vi "MultiOpto_1.2_Host.vi"() -> ()   [LabVIEW 2018]
uses:
  D:/NI LabVIEW/MultiOpto/MultiOpto_1.2/AT lib/Spels.AutomationTools.Utility.Wcf.dll
  AT lib/Spels.AutomationTools.Utility.Wcf.dll
  D:/NI LabVIEW/MultiOpto/MultiOpto_1.2/AT lib/AmateurStepperMotor.dll
  AT lib/AmateurStepperMotor.dll
  <instrlib>/niDMM/nidmm.llb/niDMM Resolution in Digits.ctl
  <instrlib>/niDMM/nidmm.llb/niDMM Function.ctl
  <instrlib>/niDCPower/nidcpower.llb/niDCPower Measurement Type.ctl
  <instrlib>/niDMM/nidmm.llb/niDMM Configure Measurement Digits.vi
  <instrlib>/niScope/Configure/Trigger/niScope Configure Trigger Window.vi
  <instrlib>/niScope/Acquire/Fetch/niScope Multi Fetch Cluster.vi
  <instrlib>/niScope/Acquire/Fetch/niScope Fetch.vi
panel:
  in  "SIM_SEL":bool
  in  "SEL path":path=path "D:/NI LabVIEW/MultiOpto/MultiOpto_1.2/Logs/SEL" caption="SEL Path"
  in  "SEL Time Cycle":u32=100
  in  "Считать SIM_SEL":bool
  in  "Desicion Panel":enum32{"Decision Panel", "System Panel"}(tab)
  in  "HMI Stop":bool
  out "SEU":bool caption="SEL"
  out "SEL":bool
  out "DC Power 2 Status":bool caption="DC Power 2"
  out "DC Power 1 Status":bool caption="DC Power 1"
  out "NI DMM 3 Status":bool caption="NI DMM 3"
  out "NI DMM 2 Status":bool caption="NI DMM 2"
  out "NI DMM 1 Status":bool caption="NI DMM 1"
  out "NI Scope Status":bool caption="NI Scope"
  out "Stepper Motor Status":bool caption="Stepper Motor"
  out "Ophir 1 Status":bool caption="Ophir 1"
  out "Ophir 2 Status":bool caption="Ophir 2"
  in  "System Stop":bool=TRUE
  out "Ready Status":bool=TRUE
  out "Power OFF":bool=TRUE
  in  "Tab DC Power 2":enum32{"DC Power 2", "System Panel"}(tab)
  in  "P2 CH2_selcur, A":dbl=0.2 caption="current limit" format="%_6p"
  out "P2 CH2_warning":bool caption="VCC_warning"
  out "P2 CH2_counter":u32 caption="VCC_counter"
  in  "P2 CH2 Used":bool caption="CH2"
  in  "P2 CH2_curlim, A":dbl=0.015 caption="current limit" min=0.01 max=1.0 format="%_6p"
  out "P2 CH2_cur, A":dbl=-2.6497095286784e-07 caption="measurement" format="%_6g"
  in  "P2 CH2, V":dbl caption="voltage level" min=-20.0 max=0.0 format="%_6p"
  out "P2 CH2_char":dbl(graph)=-2.6497095286784e-07
  in  "P2 CH2":bool
  in  "P2 CH0 Used":bool caption="CH0"
  in  "DC POWER 2":refnum<k15>="PXI1Slot3_3" caption="PRBS"
  out "P2 CH0_char":dbl(graph)=0.00011627237241327378
  in  "P2 CH0, V":dbl=1.2000000000000002 caption="voltage level" min=0.0 max=6.0 format="%_6p"
  out "P2 CH0_cur, A":dbl=0.00011627237241327378 caption="measurement" format="%_6g"
  in  "P2 CH0_curlim, A":dbl=0.04 caption="current limit" min=0.01 max=1.0 format="%_6p"
  in  "P2 CH0":bool
  out "P2 CH0_warning":bool caption="VCC_warning"
  out "P2 CH0_counter":u32 caption="VCC_counter"
  in  "P2 CH0_selcur, A":dbl=0.2 caption="current limit" format="%_6p"
  in  "P2 CH1_curlim, A":dbl=0.1 caption="current limit" min=0.01 max=1.0 format="%_6p"
  out "P2 CH1_cur, A":dbl=-6.586231837824974e-06 caption="measurement" format="%_6g"
  in  "P2 CH1, V":dbl=20.0 caption="voltage level" min=0.0 max=20.0 format="%_6p"
  out "P2 CH1_char":dbl(graph)=-6.586231837824974e-06
  in  "P2 CH1":bool
  in  "P2 CH1 Used":bool caption="CH1"
  in  "P2 CH1_selcur, A":dbl=0.2 caption="current limit" format="%_6p"
  out "P2 CH1_counter":u32 caption="VCC_counter"
  out "P2 CH1_warning":bool caption="VCC_warning"
  out "DC Power 2 error out":errorcluster
  in  "Tab DC Power 1":enum32{"DC Power 1", "System Panel"}(tab)
  out "P1 CH2_counter":u32 caption="VCC_counter"
  out "P1 CH2_warning":bool caption="VCC_warning"
  in  "P1 CH2_selcur, A":dbl=0.2 caption="current limit" format="%_6p"
  in  "P1 CH2 Used":bool caption="CH2"
  in  "P1 CH2_curlim, A":dbl=0.01 caption="current limit" min=0.01 max=1.0 format="%_6p"
  out "P1 CH2_cur, A":dbl=1.4003158139382402e-06 caption="measurement" format="%_6g"
  in  "P1 CH2, V":dbl=-5.0 caption="voltage level" min=-20.0 max=0.0 format="%_6p"
  out "P1 CH2_char":dbl(graph)=1.4003158139382402e-06
  in  "P1 CH2":bool
  in  "P1 CH1 Used":bool caption="CH1"
  in  "P1 CH0 Used":bool caption="CH0"
  in  "DC POWER 1":refnum<k15>="PXI1Slot2_2" caption="VСС_+5"
  out "P1 CH0_char":dbl(graph)=8.200132019086688e-05
  in  "P1 CH0, V":dbl=3.3000000000000003 caption="voltage level" min=0.0 max=6.0 format="%_6p"
  out "P1 CH0_cur, A":dbl=8.200132019086688e-05 caption="measurement" format="%_6g"
  in  "P1 CH0_curlim, A":dbl=0.08 caption="current limit" min=0.01 max=1.0 format="%_6p"
  out "P1 CH1_char":dbl(graph)=9.464711192498274e-07
  in  "P1 CH1, V":dbl=2.0 caption="voltage level" min=0.0 max=20.0 format="%_6p"
  out "P1 CH1_cur, A":dbl=9.464711192498274e-07 caption="measurement" format="%_6g"
  in  "P1 CH1_curlim, A":dbl=0.1 caption="current limit" min=0.01 max=1.0 format="%_6p"
  in  "P1 CH0":bool
  in  "P1 CH1":bool
  out "P1 CH0_warning":bool caption="VCC_warning"
  out "P1 CH0_counter":u32 caption="VCC_counter"
  out "P1 CH1_warning":bool caption="VCC_warning"
  out "P1 CH1_counter":u32 caption="VCC_counter"
  in  "P1 CH1_selcur, A":dbl=0.2 caption="current limit" format="%_6p"
  in  "P1 CH0_selcur, A":dbl=0.2 caption="current limit" format="%_6p"
  out "DC Power 1 error out":errorcluster
  out "SEL output file refnum":refnum<file>
  in  "Table Tab":enum32{"Glass Table", "Var", "Log"}(tab)
  in  "Add Log Remark":bool
  in  "Glass Table":string[][](table)=[["", "455 nm", "808 nm", "1550 nm"], ["Glass 1 (H-ZLaF90)", "", "", ""], ["Glass 2 (H-K9L)", "", "", ""], ["Glass 3 (H-ZF7LA)", "", "", ""], ["Glass 4 (H-LaK7A)", "", "", ""]]
  in  "Clear Table":bool
  out "Num of Meas":u32
  in  "Log Remark":string
  out "WL 808":dbl format="%#_4g"
  out "WL 455":dbl format="%#_4g"
  out "WL 1550":dbl format="%#_4g"
  out "WL 1550 Ref":dbl=1.0 format="%#_4g"
  out "WL 455 Ref":dbl=1.0 format="%#_4g"
  out "WL 808 Ref":dbl=1.0 format="%#_4g"
  out "WL 455 Absolute/Reference":string="-" caption="WL 455 Abs/Ref"
  out "WL 808 Absolute/Reference":string="-" caption="WL 808 Abs/Ref"
  out "WL 1550 Absolute/Reference":string="-" caption="WL 1550 Abs/Ref"
  in  "Set Last Meas As Ref":bool
  out "Образец №":string="0"
  in  "All Glass Path":path=path "D:/NI LabVIEW/MultiOpto/MultiOpto_1.2/Logs/All Glass"
  in  "NI Scope":refnum<k15>="PXI1Slot9_2" caption="Scope"
  in  "NI DMM 3":refnum<k15>="PXI1Slot6_3" caption="NI DMM 2"
  in  "Stepper Motor Control":enum32{"Stepper Motor", "System Panel", "Var"}(tab)
  out "Текущая позиция":dbl
  in  "Куда едем?":T1(ring)
  in  "Glass Meas":bool caption="Glass Measurement"
  out "Meas Running":bool
  out "Glass Meas Cycle Running":bool caption="Cycle Running"
  in  "Погнали!":bool
  out "Готово":bool
  in  "Glass Meas Cycle":bool caption="Glass Measament Cycle"
  out "Meas Progress Bar":u8(slide) caption="Measurement Progress Bar" scale=0.0..100.0
  in  "StepDivisor":i32(ring)=8 items=["D1"=1, "D2"=2, "D4"=4, "D8"=8, "D16"=16, "D32"=32]
  in  "Speed":dbl=1000.0
  in  "StepMultiplicationFactor":dbl=1.0
  in  "Стоп_тест":bool
  in  "Тест":bool
  in  "Стоп GoTo":bool
  in  "Meas Wait":u32=500
  out "Av Cur Data String":string="0,000016350563\t"
  out "Glass Num Output File":refnum<file>
  out "Glass 1 Output File":refnum<file>
  out "CH Data String":string="1,200000000000\t0,040047418764\t"
  out "All Cur Data String":string="0,000016366024\t0,000016373619\t0,000016386890\t0,000016310874\t0,000016315407\t"
  out "Meas Time String":string="19:17:01:,978\t"
  out "Glass Meas Path":refnum<file>
  out "Glass 2 Output File":refnum<file>
  out "Glass 3 Output File":refnum<file>
  out "Glass 4 Output File":refnum<file>
  out "Glass Full Log Output File":refnum<file>
  out "Save Glass Log Done":bool=TRUE
  in  "Save Glass Log Data":bool
  out "WL-i":i32
  out "Single Meas Output File":refnum<file>
  in  "NI DMM 3 Tab":enum32{"Amp", "Ohm", "System Panel", "Var"}(tab)
  in  "NI DMM 3 Ampermeter path":path=path "D:/NI LabVIEW/MultiOpto/MultiOpto_1.2/Logs/DMM 3" caption="Ampermeter Path"
  out "NI DMM 3 Current Char":dbl(graph)=0.00060711613514286
  in  "NI DMM 3 Current Wait":u32=100 caption="Wait"
  out "NI DMM 3 Current":dbl=0.00060711613514286 caption="Current" format="%_6g"
  in  "NI DMM 3 units":string(combo)="1000000" caption="Units"
  in  "NI DMM 3 Current Range":string(combo)="-1" caption="Range"
  in  "NI DMM 3 Ohmmeter path":path=path "D:/NI LabVIEW/MultiOpto/MultiOpto_1.2/Logs/DMM 3" caption="Ohmmeter Path"
  out "NI DMM 3 Resistance Char":dbl(graph)=6.67426339573744e-05
  in  "NI DMM 3 Resistance Wait":u32=100 caption="Wait"
  out "NI DMM 3 Resistance":dbl caption="Resistance" format="%_6g"
  in  "NI DMM 3 Resistance units":string(combo)="1" caption="Units"
  in  "NI DMM 3 Resistance Range":string(combo)="-1" caption="Range"
  out "NI DMM 3 Current output file":refnum<file>
  out "NI DMM 3 Resistance output file":refnum<file>
  in  "NI DMM 3 error in":errorcluster
  out "NI DMM 3 Option Return":enum32{"Ampermeter button", "Ohmmeter button"}(ring)
  out "NI DMM 3 error out":errorcluster
  out "DMM 3 Real Current":dbl=6.0711613514286e-10 format="%.15f"
  in  "NI DMM 1":refnum<k15>="PXI1Slot4"
  in  "NI DMM 2":refnum<k15>="PXI1Slot5"
  in  "Ophir 2 Tab":T2(tab)
  out "Ophir 2 Initialization":bool caption="Initialization"
  in  "Ophir 2 Clear":bool caption="Clear"
  out "Ophir 2 MAX":dbl caption="MAX" format="%#_5g"
  out "Ophir 2 Optical Power":dbl caption="Power" format="%#_4g"
  in  "Ophir 2 units":string(combo)="1000" caption="Units"
  in  "Ophir 2 Info":u16(ring)=1 caption="Info" items=["Device : JUNO; s/n:903794", "Head : PD300-IRG-v1; s/n:908004"]
  in  "Ophir 2 Wait":u32=100 caption="Wait"
  out "Ophir 2 Char":dbl(graph)=6.67426339573744e-05
  out "Ophir 2 Over Range":bool caption="Over Range"
  out "Ophir 2 dup Visa Session":refnum<visa-resource-name>="USB0::0x0BD3::0x0777::NI-VISA-10003::RAW" caption="dup Visa Session"
  in  "Ophir 2 GPIB Address (10)":string="10" caption="GPIB Address (10)"
  in  "Ophir 2 Select Communication Protocol":u16(ring) caption="Select Communication Protocol" items=["USB", "RS232", "GPIB"]
  in  "Ophir 2 usb channel":i16 caption="usb channel"
  in  "Ophir 2 Baud Rate (3:9600)":i16(ring)=3 caption="Baud Rate (3:9600)" items=["300", "1200", "4800", "9600", "19200", "38400"]
  in  "Ophir 2 Port Number (default 2)":i16=2 caption="Port Number (default 2)" min=0 max=20
  out "Ophir 2 Real Optical Power":dbl format="%.6e"
  out "Ophir 2 error out":errorcluster caption="error out"
  in  "Ophir 2 error in (no error)":errorcluster caption="error in (no error)"
  in  "Ophir 1 Tab":T3(tab)
  out "Ophir 1 Initialization":bool caption="Initialization"
  in  "Ophir 1 units":string(combo)="1000" caption="Units"
  out "Ophir 1 Optical Power":dbl caption="Power" format="%#_4g"
  out "Ophir 1 MAX":dbl caption="MAX" format="%#_5g"
  in  "Ophir 1 Clear":bool caption="Clear"
  in  "Ophir 1 Info":u16(ring)=1 caption="Info" items=["Device : JUNO; s/n:903795", "Head : PD300R-IR   ; s/n:873888"]
  in  "Ophir 1 Wait":u32=100 caption="Wait"
  out "Ophir 1 Char":dbl(graph)=6.67426339573744e-05
  out "Ophir 1 Over Range":bool caption="Over Range"
  in  "Ophir 1 Select Communication Protocol":u16(ring) caption="Select Communication Protocol" items=["USB", "RS232", "GPIB"]
  in  "Ophir 1 usb channel":i16 caption="usb channel"
  in  "Ophir 1 Port Number (default 2)":i16=1 caption="Port Number (default 2)" min=0 max=20
  in  "Ophir 1 Baud Rate (3:9600)":i16(ring)=3 caption="Baud Rate (3:9600)" items=["300", "1200", "4800", "9600", "19200", "38400"]
  in  "Ophir 1 GPIB Address (10)":string="10" caption="GPIB Address (10)"
  out "Ophir 1 dup Visa Session":refnum<visa-resource-name>="USB0::0x0BD3::0x0777::NI-VISA-10003::RAW" caption="dup Visa Session"
  out "Ophir 1 Real Optical Power":dbl format="%.6e"
  out "Ophir 1 error out":errorcluster caption="error out"
  in  "Ophir 1 error in (no error)":errorcluster caption="error in (no error)"
  in  "NI DMM 2 Tab":enum32{"Amp", "Ohm", "System Panel", "Var"}(tab)
  out "NI DMM 2 Current":dbl=0.7074877999002638 caption="Current" format="%_4g"
  out "NI DMM 2 Current Char":dbl(graph)=0.7074877999002638
  in  "NI DMM 2 Ampermeter path":path=path "D:/NI LabVIEW/MultiOpto/MultiOpto_1.2/Logs/DMM 2" caption="Ampermeter Path"
  in  "NI DMM 2 units":string(combo)="1000000" caption="Units"
  in  "NI DMM 2 Current Range":string(combo)="-1" caption="Range"
  in  "NI DMM 2 Current Wait":u32=100 caption="Wait"
  in  "NI DMM 2 Ohmmeter path":path=path "D:/NI LabVIEW/MultiOpto/MultiOpto_1.2/Logs/DMM 2" caption="Ohmmeter Path"
  out "NI DMM 2 Resistance":dbl caption="Resistance" format="%_6g"
  out "NI DMM 2 Resistance Char":dbl(graph)=6.67426339573744e-05
  in  "NI DMM 2 Resistance units":string(combo)="1" caption="Units"
  in  "NI DMM 2 Resistance Range":string(combo)="-1" caption="Range"
  in  "NI DMM 2 Resistance Wait":u32=100 caption="Wait"
  out "NI DMM 2 Current output file":refnum<file>
  out "NI DMM 2 error out":errorcluster
  in  "NI DMM 2 error in":errorcluster
  out "NI DMM 2 Option Return":enum32{"Ampermeter button", "Ohmmeter button"}(ring)
  out "NI DMM 2 Resistance output file":refnum<file>
  out "DMM 2 Real Current":dbl=7.074877999002638e-07 format="%.15f"
  in  "NI DMM 1 Tab":enum32{"Amp", "Ohm", "System Panel", "Var"}(tab)
  out "NI DMM 1 Current Char":dbl(graph)=0.6705812438667635
  out "NI DMM 1 Current":dbl=0.6705812438667635 caption="Current" format="%_6g"
  in  "NI DMM 1 Ampermeter path":path=path "D:/NI LabVIEW/MultiOpto/MultiOpto_1.2/Logs/DMM 1" caption="Ampermeter Path"
  in  "NI DMM 1 units":string(combo)="1000000" caption="Units"
  in  "NI DMM 1 Current Range":string(combo)="-1" caption="Range"
  in  "NI DMM 1 Current Wait":u32=100 caption="Wait"
  in  "NI DMM 1 Ohmmeter path":path=path "D:/NI LabVIEW/MultiOpto/MultiOpto_1.2/Logs/DMM 1" caption="Ohmmeter Path"
  out "NI DMM 1 Resistance":dbl caption="Resistance" format="%_6g"
  out "NI DMM 1 Resistance Char":dbl(graph)=6.67426339573744e-05
  in  "NI DMM 1 Resistance units":string(combo)="1" caption="Units"
  in  "NI DMM 1 Resistance Range":string(combo)="-1" caption="Range"
  in  "NI DMM 1 Resistance Wait":u32=100 caption="Wait"
  out "NI DMM 1 Current output file":refnum<file>
  out "NI DMM 1 error out":errorcluster
  in  "NI DMM 1 error in":errorcluster
  out "NI DMM 1 Option Return":enum32{"Ampermeter button", "Ohmmeter button"}(ring)
  out "NI DMM 1 Resistance output file":refnum<file>
  out "DMM 1 Real Current":dbl=6.705812438667635e-07 format="%.15f"
  in  "NI Scope Tab":enum32{"NI Scope", "System Panel"}(tab)
  in  "vertical range":dbl=2.0 caption="Vertical Range" format="%.2f"
  out "RealTime Waveform":T4(graph) caption="PC_MON Waveform"
  out "SEU Waveform":T4(graph) caption="SHUTDOWN Waveform"
  in  "Low Level":dbl=0.35 format="%.2f"
  in  "High Level":dbl=0.65 format="%.2f"
  in  "AC/DC/Groun":i32(ring)=1 items=["AC", "DC", "Ground"]
  in  "Trigger Source":string(combo)="0"
  in  "SEU path":path=path "D:/NI LabVIEW/MultiOpto 1.1/Logs/SEU" caption="SEU Path"
  in  "Channel for SEU":T5(radio)
  out "SEU Last Level":dbl
  out "SEU_Counter":u32 caption="SEU counter"
  out "SEU_warning":bool caption="Find SEL"
  out "SEU output file refnum":refnum<file>
  out "NI Scope error out":errorcluster
  in  "NI Scope error in":errorcluster
  # "Отожми кнопку для\nединичного промера!"
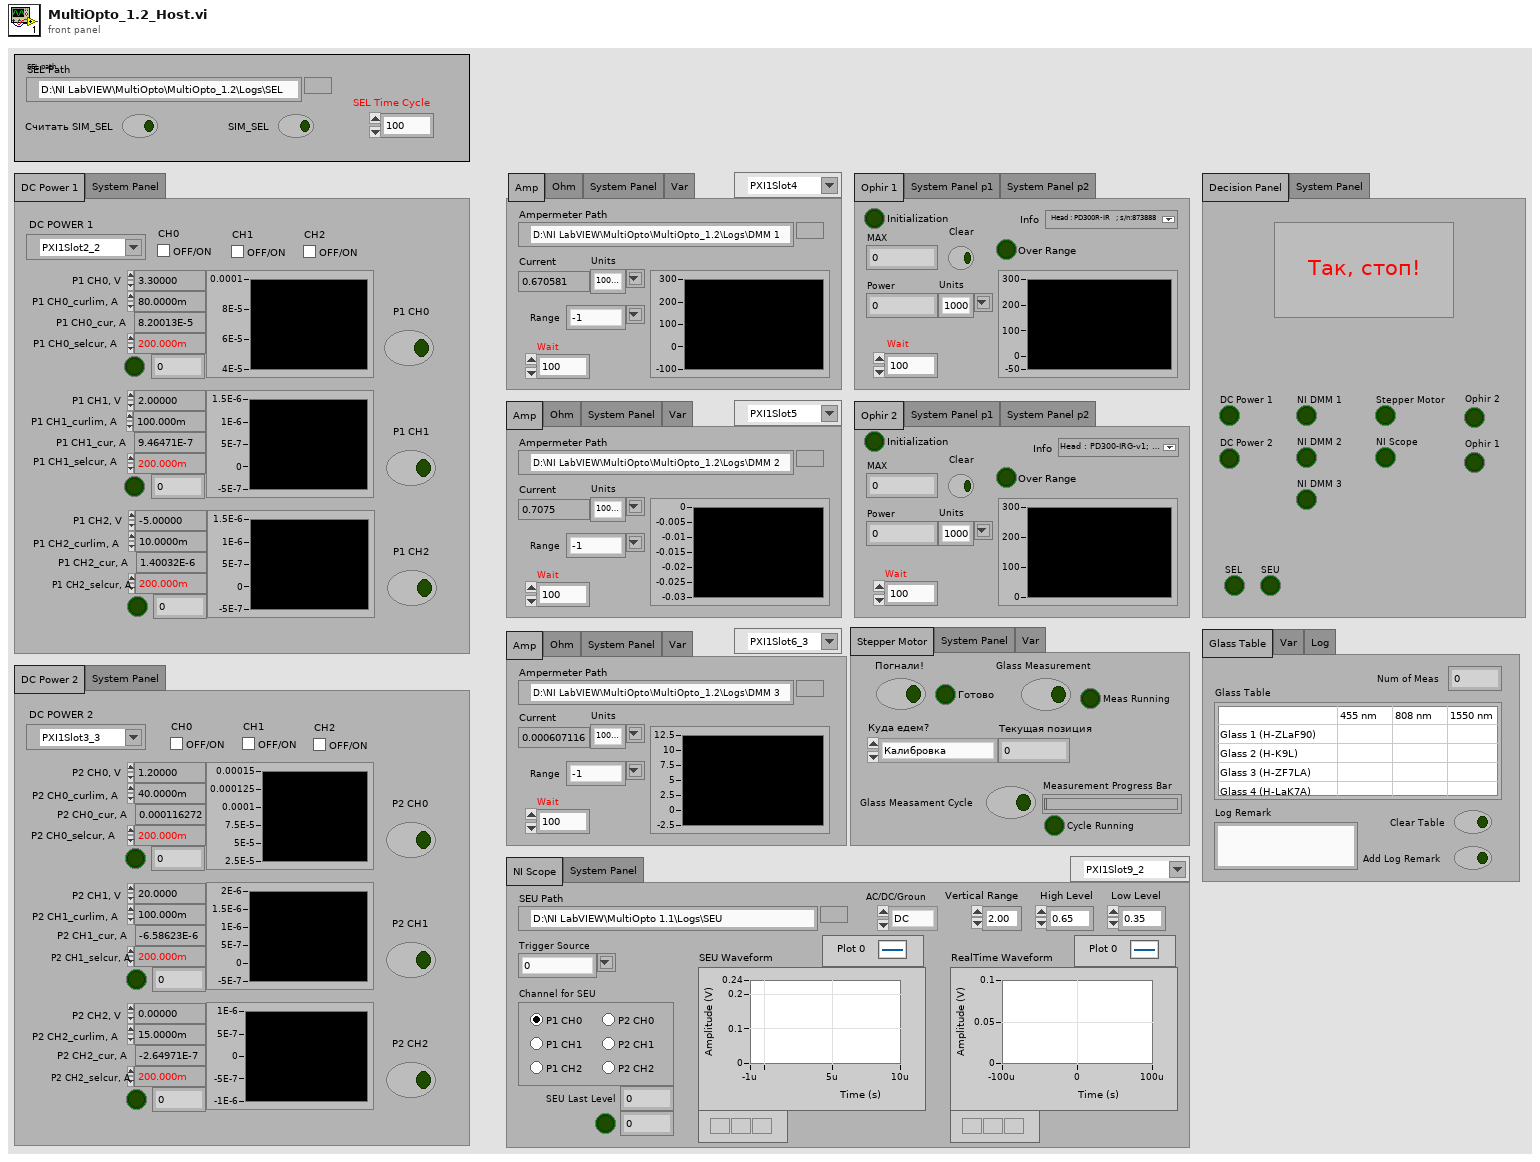
[diagram p1: front panel]
types:
  T1 = enum16{"Калибровка", "Первое стекло", "Второе стекло", "Третье стекло", "Четвертое стекло"}
  T2 = enum32{"Ophir 2", "System Panel p1", "System Panel p2"}
  T3 = enum32{"Ophir 1", "System Panel p1", "System Panel p2"}
  T4 = cluster{"relativeInitialX":dbl, "xIncrement":dbl, "wfm":dbl[]}[]
  T5 = enum32{"Radio Selection P1 CH0", "Radio Selection P1 CH1", "Radio Selection P2 CH0", "Radio Selection P2 CH1", "Radio Selection P2 CH2", "Radio Selection P1 CH2"}
  T6 = enum16{"open", "replace", "create", "open or create", "replace or create", "replace or create with confirmation"}
  T7 = enum8{"Enabled", "Disabled", "Disabled and Grayed Out"}
  T8 = typedef "niDMM Function.ctl" = enum16{"DC Volts", "AC Volts", "DC Current", "AC Current", "2-wire Resistance", "4-wire Resistance", "Diode", "Frequency", "Period", "AC Volts DC Coupled", "Capacitance", "Inductance", "Temperature"}
  T9 = typedef "niDMM Resolution in Digits.ctl" = dbl
  T10 = typedef "niDCPower Measurement Type.ctl" = i32
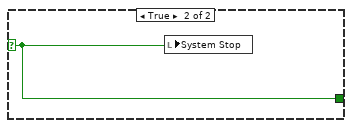
[diagram p5: hidden frame]
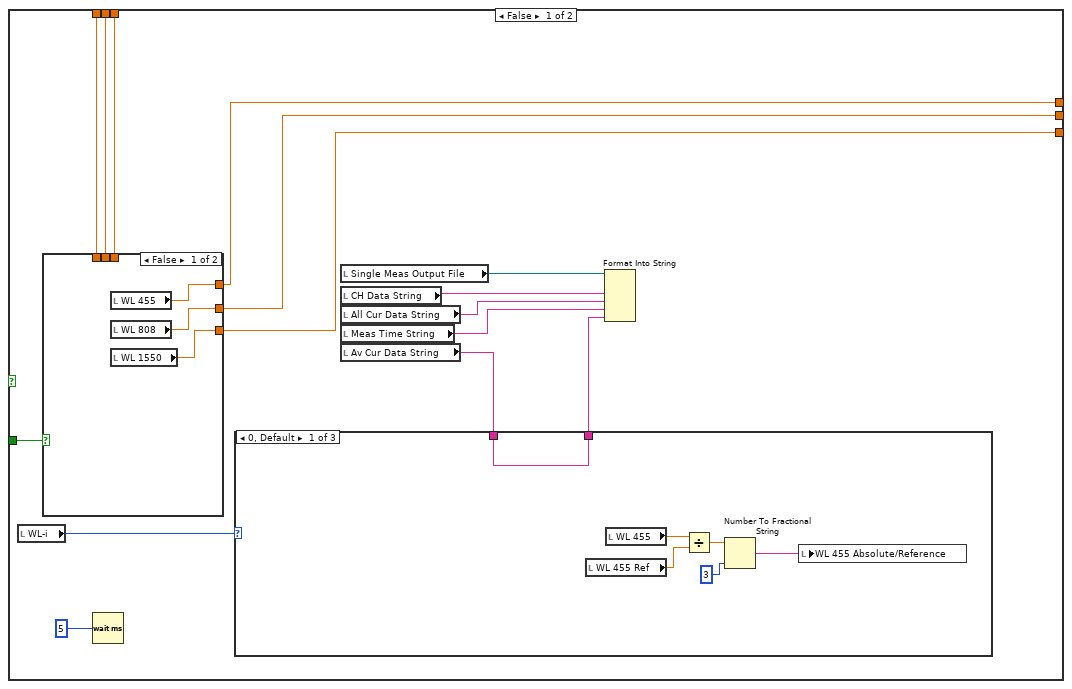
[diagram p9: hidden frame]
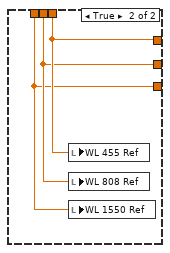
[diagram p10: hidden frame]
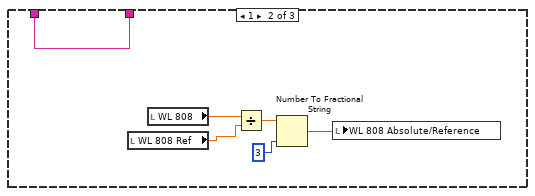
[diagram p11: hidden frame]
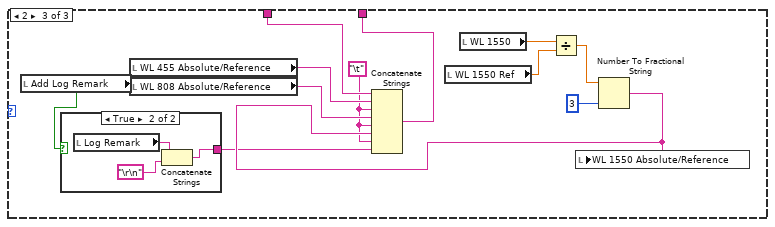
[diagram p12: hidden frame]
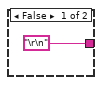
[diagram p13: hidden frame]
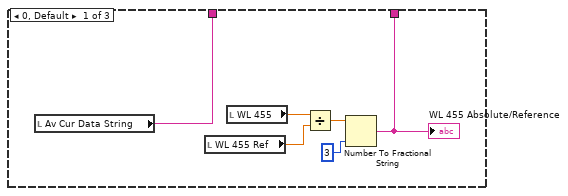
[diagram p14: hidden frame]
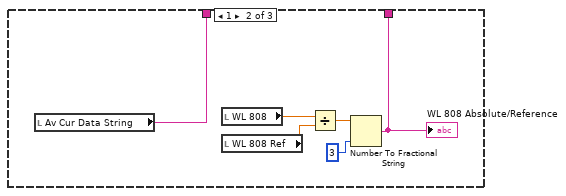
[diagram p15: hidden frame]
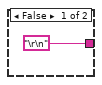
[diagram p16: hidden frame]
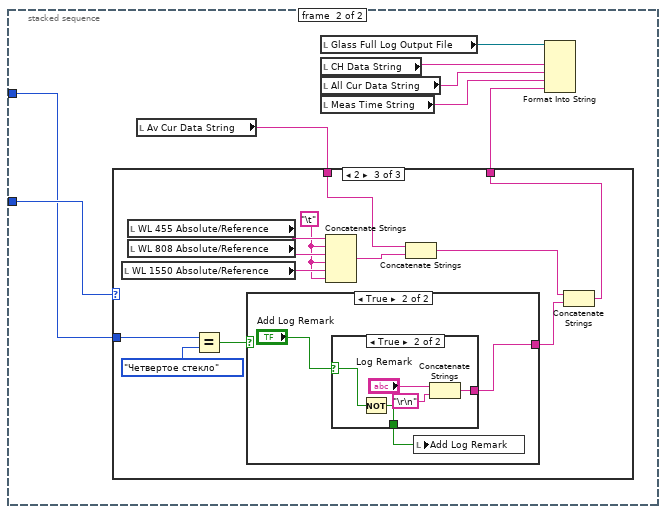
[diagram p17: hidden frame]
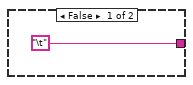
[diagram p20: hidden frame]
diagram:
  # "DMM 3"
  # "DMM 2"
  # "DMM 1"
  n1 = stacked-sequence {
    tunnel: [_ _ _ _ _ w336 _ _ _ _ _ _] -> w36
    tunnel: [_ _ _ _ _ w335 _ _ _ _ _ _] -> w34
    tunnel: [_ _ _ _ _ w334 _ _ _ _ _ _] -> w7
    tunnel: [_ _ _ _ _ _ _ _ _ _ _ w687] -> w8
    tunnel: [_ _ _ _ _ _ _ _ _ _ _ w687] -> w10
    tunnel: [_ _ _ _ _ _ w361 _ _ _ _ _] -> w33
    tunnel: [_ _ _ _ _ _ _ w420 _ _ _ _] -> w32
    tunnel: [_ _ _ _ _ _ _ w423 _ _ _ _] -> w31
    tunnel: [_ _ _ _ _ _ w360 _ _ _ _ _] -> w30
    tunnel: [_ _ _ _ _ _ _ w419 _ _ _ _] -> w29
    tunnel: [_ _ _ _ _ _ _ w418 _ _ _ _] -> w28
    tunnel: [_ _ _ _ _ _ w359 _ _ _ _ _] -> w27
    tunnel: [_ _ _ _ _ _ _ w422 _ _ _ _] -> w26
    tunnel: [_ _ _ _ _ _ _ w421 _ _ _ _] -> w25
    tunnel: [_ _ _ _ _ _ _ _ w616 _ _ _] -> w24
    tunnel: [_ _ _ _ _ _ _ _ _ w639 _ _] -> w23
    tunnel: [_ _ _ _ _ _ _ w417 _ _ _ _] -> w9
    tunnel: [_ _ _ _ _ _ _ w416 _ _ _ _] -> w22
    tunnel: [_ _ _ _ _ _ _ w415 _ _ _ _] -> w21
    tunnel: [_ _ _ _ _ _ _ _ _ _ w665 _] -> w20
    tunnel: [_ _ _ _ _ _ _ _ _ _ w664 _] -> w19
    tunnel: [_ _ _ _ _ _ _ _ _ _ w663 _] -> w18
    tunnel: [_ _ _ _ _ _ _ _ _ _ w662 _] -> w17
    tunnel: [_ _ _ _ _ w333 _ _ _ _ _ _] -> w6
    tunnel: [_ _ _ _ _ w332 _ _ _ _ _ _] -> w3
    tunnel: [_ _ _ _ _ w331 _ _ _ _ _ _] -> w2
    frame #0 {
      w51 = FALSE ("Clear Table")
      w54 = "-" ("WL 455 Absolute/Reference")
      w55 = 0.0 ("WL 455 Ref")
      w56 = 1.0 ("WL 455")
      w58 = "\t" ("Meas Time String")
      w60 = FALSE ("Save Glass Log Done")
      w62 = FALSE ("Погнали!")
      w66 = FALSE
      w65 = FALSE ("NI Scope Status")
      w69 = u32 0 ("SEU_Counter")
      w59 = FALSE ("STOP")
      # "Начальная конфигурация переменных"
      n2 = local write "Текущая позиция"(0.0 ("Текущая позиция")) -> ()
      n3 = local write "Куда едем?"(T1."Калибровка" ("Куда едем?")) -> ()
      n4 = local write "Погнали!"(w62) -> ()
      n5 = local write "Тест"(w62) -> ()
      n6 = local write "Стоп GoTo"(w62) -> ()
      n7 = local write "Стоп_тест"(w62) -> ()
      n8 = local write "Готово"(w62) -> ()
      n9 = local write "Num of Meas"(u32 0 ("Num of Meas")) -> ()
      n10 = local write "WL 455"(w56) -> ()
      n11 = local write "WL 808"(w56) -> ()
      n12 = local write "WL 1550"(w56) -> ()
      n13 = local write "WL 455 Ref"(w55) -> ()
      n14 = local write "WL 808 Ref"(w55) -> ()
      n15 = local write "WL 1550 Ref"(w55) -> ()
      n16 = local write "WL 455 Absolute/Reference"(w54) -> ()
      n17 = local write "WL 808 Absolute/Reference"(w54) -> ()
      n18 = local write "WL 1550 Absolute/Reference"(w54) -> ()
      n19 = local write "Ophir 2 Over Range"(w66) -> ()
      n20 = local write "Ophir 1 Over Range"(w66) -> ()
      n21 = local write "Ophir 1 Initialization"(w66) -> ()
      n22 = local write "Ophir 2 Initialization"(w66) -> ()
      n23 = local write "Ophir 1 Clear"(w66) -> ()
      n24 = local write "Ophir 2 Clear"(w66) -> ()
      n25 = local write "Meas Time String"(w58) -> ()
      n26 = local write "All Cur Data String"(w58) -> ()
      n27 = local write "Av Cur Data String"(w58) -> ()
      n28 = local write "CH Data String"(w58) -> ()
      n29 = local write "WL-i"(0 ("i-WL")) -> ()
      n30 = local write "Save Glass Log Data"(w60) -> ()
      n31 = local write "Save Glass Log Done"(w60) -> ()
      n32 = local write "Glass Meas Cycle"(w60) -> ()
      n33 = local write "Glass Meas"(w60) -> ()
      n34 = local write "Meas Running"(w60) -> ()
      n35 = local write "Glass Meas Cycle Running"(w60) -> ()
      n36 = local write "HMI Stop"(w59) -> ()
      n37 = local write "System Stop"(w59) -> ()
      n38 = local write "P1 CH0"(w59) -> ()
      n39 = local write "P1 CH1"(w59) -> ()
      n40 = local write "P2 CH0"(w59) -> ()
      n41 = local write "P2 CH1"(w59) -> ()
      n42 = local write "Power OFF"(w59) -> ()
      n43 = local write "P1 CH0 Used"(w59) -> ()
      n44 = local write "P1 CH1 Used"(w59) -> ()
      n45 = local write "P1 CH2 Used"(w59) -> ()
      n46 = local write "P2 CH0 Used"(w59) -> ()
      n47 = local write "P2 CH1 Used"(w59) -> ()
      n48 = local write "P2 CH2 Used"(w59) -> ()
      n49 = local write "Считать SIM_SEL"(w59) -> ()
      n50 = local write "SEL"(w59) -> ()
      n51 = local write "SEU"(w59) -> ()
      n52 = local write "SEU_warning"(w59) -> ()
      n53 = local write "P1 CH0_warning"(w59) -> ()
      n54 = local write "P1 CH1_warning"(w59) -> ()
      n55 = local write "P2 CH0_warning"(w59) -> ()
      n56 = local write "P2 CH1_warning"(w59) -> ()
      n57 = local write "SEU_warning"(w59) -> ()
      n58 = local write "Log Remark"("" ("Log Remark")) -> ()
      n59 = local write "Set Last Meas As Ref"(w51) -> ()
      n60 = local write "Clear Table"(w51) -> ()
      n61 = local write "Add Log Remark"(w51) -> ()
      n62 = local write "SEU Last Level"(0.0 ("SEU Level")) -> ()
      n63 = local write "SEU_Counter"(w69) -> ()
      n64 = local write "P1 CH0_counter"(w69) -> ()
      n65 = local write "P1 CH1_counter"(w69) -> ()
      n66 = local write "P2 CH0_counter"(w69) -> ()
      n67 = local write "P2 CH1_counter"(w69) -> ()
      n68 = local write "Образец №"("" ("Образец №")) -> ()
      n69 = local write "Ready Status"(FALSE ("Ready Status")) -> ()
      n70 = local write "NI Scope Status"(w65) -> ()
      n71 = local write "NI DMM 2 Status"(w65) -> ()
      n72 = local write "NI DMM 1 Status"(w65) -> ()
      n73 = local write "NI DMM 3 Status"(w65) -> ()
      n74 = local write "Ophir 1 Status"(w65) -> ()
      n75 = local write "Ophir 2 Status"(w65) -> ()
      n76 = local write "Stepper Motor Status"(w65) -> ()
      "Meas Progress Bar" <- u8 0 ("Measuering Progress Bar")
    }
    frame #1 {
      n77 = stacked-sequence {
        frame #0 {
          w71 = T7."Disabled and Grayed Out" ("Disabled")
          n78 = property on="P1 CH0" class="Bool (strict)"("DisabledEnum"=w71) -> ()  [unwired: 2 in, 2 out]
          n79 = property on="P1 CH0_char" class="WFChart (strict)"("DisabledEnum"=w71) -> ()  [unwired: 2 in, 2 out]
          n80 = property on="P1 CH0, V" class="DigNum (strict)"("DisabledEnum"=w71) -> ()  [unwired: 2 in, 2 out]
          n81 = property on="P1 CH0_curlim, A" class="DigNum (strict)"("DisabledEnum"=w71) -> ()  [unwired: 2 in, 2 out]
          n82 = property on="P1 CH0_cur, A" class="DigNum (strict)"("DisabledEnum"=w71) -> ()  [unwired: 2 in, 2 out]
          n83 = property on="P1 CH0_selcur, A" class="DigNum (strict)"("DisabledEnum"=w71) -> ()  [unwired: 2 in, 2 out]
          n84 = property on="P1 CH0_counter" class="DigNum (strict)"("DisabledEnum"=w71) -> ()  [unwired: 2 in, 2 out]
          n85 = property on="P1 CH0_warning" class="Bool (strict)"("DisabledEnum"=w71) -> ()  [unwired: 2 in, 2 out]
        }
        frame #1 {
          w72 = T7."Disabled and Grayed Out" ("Disabled")
          n86 = property on="P1 CH1" class="Bool (strict)"("DisabledEnum"=w72) -> ()  [unwired: 2 in, 2 out]
          n87 = property on="P1 CH1_char" class="WFChart (strict)"("DisabledEnum"=w72) -> ()  [unwired: 2 in, 2 out]
          n88 = property on="P1 CH1, V" class="DigNum (strict)"("DisabledEnum"=w72) -> ()  [unwired: 2 in, 2 out]
          n89 = property on="P1 CH1_curlim, A" class="DigNum (strict)"("DisabledEnum"=w72) -> ()  [unwired: 2 in, 2 out]
          n90 = property on="P1 CH1_cur, A" class="DigNum (strict)"("DisabledEnum"=w72) -> ()  [unwired: 2 in, 2 out]
          n91 = property on="P1 CH1_selcur, A" class="DigNum (strict)"("DisabledEnum"=w72) -> ()  [unwired: 2 in, 2 out]
          n92 = property on="P1 CH1_counter" class="DigNum (strict)"("DisabledEnum"=w72) -> ()  [unwired: 2 in, 2 out]
          n93 = property on="P1 CH1_warning" class="Bool (strict)"("DisabledEnum"=w72) -> ()  [unwired: 2 in, 2 out]
        }
        frame #2 {
          w73 = T7."Disabled and Grayed Out" ("Disabled")
          n94 = property on="P1 CH2" class="Bool (strict)"("DisabledEnum"=w73) -> ()  [unwired: 2 in, 2 out]
          n95 = property on="P1 CH2_char" class="WFChart (strict)"("DisabledEnum"=w73) -> ()  [unwired: 2 in, 2 out]
          n96 = property on="P1 CH2, V" class="DigNum (strict)"("DisabledEnum"=w73) -> ()  [unwired: 2 in, 2 out]
          n97 = property on="P1 CH2_curlim, A" class="DigNum (strict)"("DisabledEnum"=w73) -> ()  [unwired: 2 in, 2 out]
          n98 = property on="P1 CH2_cur, A" class="DigNum (strict)"("DisabledEnum"=w73) -> ()  [unwired: 2 in, 2 out]
          n99 = property on="P1 CH2_selcur, A" class="DigNum (strict)"("DisabledEnum"=w73) -> ()  [unwired: 2 in, 2 out]
          n100 = property on="P1 CH2_counter" class="DigNum (strict)"("DisabledEnum"=w73) -> ()  [unwired: 2 in, 2 out]
          n101 = property on="P1 CH2_warning" class="Bool (strict)"("DisabledEnum"=w73) -> ()  [unwired: 2 in, 2 out]
        }
        frame #3 {
          w74 = T7."Disabled and Grayed Out" ("Disabled")
          n102 = property on="P2 CH0" class="Bool (strict)"("DisabledEnum"=w74) -> ()  [unwired: 2 in, 2 out]
          n103 = property on="P2 CH0_char" class="WFChart (strict)"("DisabledEnum"=w74) -> ()  [unwired: 2 in, 2 out]
          n104 = property on="P2 CH0, V" class="DigNum (strict)"("DisabledEnum"=w74) -> ()  [unwired: 2 in, 2 out]
          n105 = property on="P2 CH0_curlim, A" class="DigNum (strict)"("DisabledEnum"=w74) -> ()  [unwired: 2 in, 2 out]
          n106 = property on="P2 CH0_cur, A" class="DigNum (strict)"("DisabledEnum"=w74) -> ()  [unwired: 2 in, 2 out]
          n107 = property on="P2 CH0_selcur, A" class="DigNum (strict)"("DisabledEnum"=w74) -> ()  [unwired: 2 in, 2 out]
          n108 = property on="P2 CH0_counter" class="DigNum (strict)"("DisabledEnum"=w74) -> ()  [unwired: 2 in, 2 out]
          n109 = property on="P2 CH0_warning" class="Bool (strict)"("DisabledEnum"=w74) -> ()  [unwired: 2 in, 2 out]
        }
        frame #4 {
          w75 = T7."Disabled and Grayed Out" ("Disabled")
          n110 = property on="P2 CH1" class="Bool (strict)"("DisabledEnum"=w75) -> ()  [unwired: 2 in, 2 out]
          n111 = property on="P2 CH1_char" class="WFChart (strict)"("DisabledEnum"=w75) -> ()  [unwired: 2 in, 2 out]
          n112 = property on="P2 CH1, V" class="DigNum (strict)"("DisabledEnum"=w75) -> ()  [unwired: 2 in, 2 out]
          n113 = property on="P2 CH1_curlim, A" class="DigNum (strict)"("DisabledEnum"=w75) -> ()  [unwired: 2 in, 2 out]
          n114 = property on="P2 CH1_cur, A" class="DigNum (strict)"("DisabledEnum"=w75) -> ()  [unwired: 2 in, 2 out]
          n115 = property on="P2 CH1_selcur, A" class="DigNum (strict)"("DisabledEnum"=w75) -> ()  [unwired: 2 in, 2 out]
          n116 = property on="P2 CH1_counter" class="DigNum (strict)"("DisabledEnum"=w75) -> ()  [unwired: 2 in, 2 out]
          n117 = property on="P2 CH1_warning" class="Bool (strict)"("DisabledEnum"=w75) -> ()  [unwired: 2 in, 2 out]
        }
        frame #5 {
          w76 = T7."Disabled and Grayed Out" ("Disabled")
          n118 = property on="P2 CH2" class="Bool (strict)"("DisabledEnum"=w76) -> ()  [unwired: 2 in, 2 out]
          n119 = property on="P2 CH2_char" class="WFChart (strict)"("DisabledEnum"=w76) -> ()  [unwired: 2 in, 2 out]
          n120 = property on="P2 CH2, V" class="DigNum (strict)"("DisabledEnum"=w76) -> ()  [unwired: 2 in, 2 out]
          n121 = property on="P2 CH2_curlim, A" class="DigNum (strict)"("DisabledEnum"=w76) -> ()  [unwired: 2 in, 2 out]
          n122 = property on="P2 CH2_cur, A" class="DigNum (strict)"("DisabledEnum"=w76) -> ()  [unwired: 2 in, 2 out]
          n123 = property on="P2 CH2_selcur, A" class="DigNum (strict)"("DisabledEnum"=w76) -> ()  [unwired: 2 in, 2 out]
          n124 = property on="P2 CH2_counter" class="DigNum (strict)"("DisabledEnum"=w76) -> ()  [unwired: 2 in, 2 out]
          n125 = property on="P2 CH2_warning" class="Bool (strict)"("DisabledEnum"=w76) -> ()  [unwired: 2 in, 2 out]
        }
        frame #6 {
          w77 = T7."Enabled" ("Disabled")
          n126 = property on="P1 CH0 Used" class="Bool (strict)"("DisabledEnum"=w77) -> ()  [unwired: 2 in, 2 out]
          n127 = property on="P1 CH1 Used" class="Bool (strict)"("DisabledEnum"=w77) -> ()  [unwired: 2 in, 2 out]
          n128 = property on="P1 CH2 Used" class="Bool (strict)"("DisabledEnum"=w77) -> ()  [unwired: 2 in, 2 out]
          n129 = property on="P2 CH0 Used" class="Bool (strict)"("DisabledEnum"=w77) -> ()  [unwired: 2 in, 2 out]
          n130 = property on="P2 CH1 Used" class="Bool (strict)"("DisabledEnum"=w77) -> ()  [unwired: 2 in, 2 out]
          n131 = property on="P2 CH2 Used" class="Bool (strict)"("DisabledEnum"=w77) -> ()  [unwired: 2 in, 2 out]
          n132 = property on="Glass Meas" class="Bool (strict)"("DisabledEnum"=w77) -> ()  [unwired: 2 in, 2 out]
        }
      }
    }
    frame #2 {
      n133 = call "MultiOpto_1.2_Begin.vi"() -> ("Текущий Образец №"=→"Образец №":string, "NI Scope Status"=→"NI Scope Status":bool, "Ophir 1 Status"=→"Ophir 1 Status":bool, "Ophir 2 Status"=→"Ophir 2 Status":bool, "DC Power 1 Status"=→"DC Power 1 Status":bool, "DC Power 2 Status"=→"DC Power 2 Status":bool, "NI DMM 1 Status"=→"NI DMM 1 Status":bool, "NI DMM 2 Status"=→"NI DMM 2 Status":bool, "Stepper Motor Status"=→"Stepper Motor Status":bool, "NI DMM 3 option return"=→"NI DMM 3 Option Return":enum32{"Ampermeter button", "Ohmmeter button"}, "NI DMM 2 option return"=→"NI DMM 2 Option Return":enum32{"Ampermeter button", "Ohmmeter button"}, "NI DMM 1 option return"=→"NI DMM 1 Option Return":enum32{"Ampermeter button", "Ohmmeter button"}, "NI DMM 3 Status"=→"NI DMM 3 Status":bool)  [unwired: 3 in]
    }
    frame #3 {
      n134 = local read "Образец №"() -> (w96:string)
      n135 = Build Path(base path="All Glass Path", name or relative path=w96) -> (appended path=w93:path)
      n136 = call <vilib>:"Check if File or Folder Exists.vi"("path"=w93) -> ("file or folder exists?"=w94:bool, "dup path"=w95:path)  [unwired: 8 in, 1 out]
      n137 = case shown="False" w94 {
        tunnel: w95 -> [w98 w99]
        tunnel: [w97 w99] -> w92
        frame False {
          n138 = Create Folder(path (use dialog)=w98) -> (created path=w97:path)  [unwired: 2 in, 2 out]
        }
        frame True {
        }
      }
      n139 = stacked-sequence {
        tunnel: w92 -> [w152 w182 w229]
        frame #0 {
          w150 = "\t"
          w102 = "\t"
          n140 = local read "Glass Table"() -> (w108:string[][])
          n141 = Index Array(array=w108, index (row)=4 ("disabled index (row)"), index (col)=0 ("disabled index (col)")) -> (element=w106:string)
          n142 = local read "Glass Table"() -> (w113:string[][])
          n143 = Index Array(array=w113, index (row)=3 ("disabled index (row)"), index (col)=0 ("disabled index (col)")) -> (element=w107:string)
          n144 = local read "Glass Table"() -> (w119:string[][])
          n145 = Index Array(array=w119, index (row)=2 ("disabled index (row)"), index (col)=0 ("disabled index (col)")) -> (element=w118:string)
          n146 = Build Path(base path=w152, name or relative path="Full Log") -> (appended path=w169:path)
          n147 = Get Date/Time In Seconds() -> (seconds since 1Jan1904=w165:timestamp)
          n148 = local read "Glass Table"() -> (w117:string[][])
          n149 = call <vilib>:"Check if File or Folder Exists.vi"("path"=w169) -> ("file or folder exists?"=w168:bool, "dup path"=w167:path)  [unwired: 8 in, 1 out]
          n150 = Index Array(array=w117, index (row)=1 ("disabled index (row)"), index (col)=0 ("disabled index (col)")) -> (element=w114:string)
          n151 = Format Date/Time String(time format string (%c)="Full Log %d %m %y %H.%M.%S", seconds (now)=w165) -> (date/time string=w164:string)  [unwired: 1 in]
          n152 = case shown="False" w168 {
            tunnel: w167 -> [w171 w172]
            tunnel: [w170 w172] -> w166
            frame False {
              n153 = Create Folder(path (use dialog)=w171) -> (created path=w170:path)  [unwired: 2 in, 2 out]
            }
            frame True {
            }
          }
          n154 = Concatenate Strings(w164, ".xls" ("string")) -> (w163:string)
          n155 = Build Path(base path=w166, name or relative path=w163) -> (appended path=w162:path)
          n156 = Concatenate Strings("P1 CH0, V" ("string"), w102, "P1 CH0 Current, A" ("string"), w102, "DMM1_1" ("string"), w102, "DMM1_2" ("string"), w102, "DMM1_3" ("string"), w102, "DMM1_4" ("string"), w102, "DMM1_5" ("string"), w102, "Time" ("string"), w102, "455 nm Current Averaged, A" ("string"), w102, "P2 CH0, V" ("string"), w102, "P2 CH0 Current, A" ("string"), w102, "DMM2_1" ("string"), w102, "DMM2_2" ("string"), w102, "DMM2_3" ("string"), w102, "DMM2_4" ("string"), w102, "DMM2_5" ("string"), w102, "Time" ("string"), w102, "808 nm Current Averaged, A" ("string"), w102, "P2 CH1, V" ("string"), w102, "P2 CH2 Current, A" ("string"), w102, "DMM3_1" ("string"), w102, "DMM3_2" ("string"), w102, "DMM3_3" ("string"), w102, "DMM3_4" ("string"), w102, "DMM3_5" ("string"), w102, "Time" ("string"), w102, "1550 nm Current Averaged, A" ("string"), w102, "455 nm Absolute/Reference" ("string"), w102, "808 nm Absolute/Reference" ("string"), w102, "1550 nm Absolute/Reference" ("string"), w102) -> (w149:string)
          n157 = Open/Create/Replace File(file path (use dialog)=w162, operation (0:open)=T6."open or create", access (0:read/write)=enum16{"read/write", "read-only", "write-only"}."read/write") -> (refnum out=w161:refnum<file>)  [unwired: 3 in, 2 out]
          n158 = Set File Position(refnum=w161, from (0:start)=enum16{"start", "end", "current"}."end") -> (refnum out=w159:refnum<file>)  [unwired: 2 in, 1 out]
          n159 = Concatenate Strings(w149, w114, w150, w149, w118, w150, w149, w107, w150, w149, w106, w150, w149, "Log Remarks" ("string"), "\r\n") -> (w158:string)
          n160 = Format Into String(initial string=w159, w158) -> (resulting string=→"Glass Full Log Output File":refnum<file>)  [unwired: 2 in, 1 out]
        }
        frame #1 {
          w175 = "\t"
          n161 = Build Path(base path=w182, name or relative path="Single Measurements") -> (appended path=w224:path)
          n162 = Get Date/Time In Seconds() -> (seconds since 1Jan1904=w220:timestamp)
          n163 = call <vilib>:"Check if File or Folder Exists.vi"("path"=w224) -> ("file or folder exists?"=w223:bool, "dup path"=w222:path)  [unwired: 8 in, 1 out]
          n164 = Format Date/Time String(time format string (%c)="Single Measurements %d %m %y %H.%M.%S", seconds (now)=w220) -> (date/time string=w219:string)  [unwired: 1 in]
          n165 = case shown="False" w223 {
            tunnel: w222 -> [w226 w227]
            tunnel: [w225 w227] -> w221
            frame False {
              n166 = Create Folder(path (use dialog)=w226) -> (created path=w225:path)  [unwired: 2 in, 2 out]
            }
            frame True {
            }
          }
          n167 = Concatenate Strings(w219, ".xls" ("string")) -> (w218:string)
          n168 = Build Path(base path=w221, name or relative path=w218) -> (appended path=w217:path)
          n169 = Concatenate Strings("P1 CH0, V" ("string"), w175, "P1 CH0 Current, A" ("string"), w175, "DMM1_1" ("string"), w175, "DMM1_2" ("string"), w175, "DMM1_3" ("string"), w175, "DMM1_4" ("string"), w175, "DMM1_5" ("string"), w175, "Time" ("string"), w175, "455 nm Current Averaged, A" ("string"), w175, "P1 CH1, V" ("string"), w175, "P1 CH1 Current, A" ("string"), w175, "DMM2_1" ("string"), w175, "DMM2_2" ("string"), w175, "DMM2_3" ("string"), w175, "DMM2_4" ("string"), w175, "DMM2_5" ("string"), w175, "Time" ("string"), w175, "808 nm Current Averaged, A" ("string"), w175, "P2 CH0, V" ("string"), w175, "P2 CH0 Current, A" ("string"), w175, "DMM3_1" ("string"), w175, "DMM3_2" ("string"), w175, "DMM3_3" ("string"), w175, "DMM3_4" ("string"), w175, "DMM3_5" ("string"), w175, "Time" ("string"), w175, "1550 nm Current Averaged, A" ("string"), w175, "455 nm Absolute/Reference" ("string"), w175, "808 nm Absolute/Reference" ("string"), w175, "1550 nm Absolute/Reference" ("string"), w175, "Log Remarks" ("string"), "\r\n") -> (w180:string)
          n170 = Open/Create/Replace File(file path (use dialog)=w217, operation (0:open)=T6."open or create", access (0:read/write)=enum16{"read/write", "read-only", "write-only"}."read/write") -> (refnum out=w216:refnum<file>)  [unwired: 3 in, 2 out]
          n171 = Set File Position(refnum=w216, from (0:start)=enum16{"start", "end", "current"}."end") -> (refnum out=w215:refnum<file>)  [unwired: 2 in, 1 out]
          n172 = Format Into String(initial string=w215, w180) -> (resulting string=→"Single Meas Output File":refnum<file>)  [unwired: 2 in, 1 out]
        }
        frame #2 {
          n173 = for {
            N: 4 -> [_]
            tunnel: w229 -> [w248]
            i -> [w240]
            w232 = "\t"
            w237 = "\t"
            n174 = local read "Glass Table"() -> (w243:string[][])
            n175 = Increment(x=w240) -> (x+1=w239:i32)
            n176 = Index Array(array=w243, index (row)=w239, index (col)=0 ("disabled index (col)")) -> (element=w242:string)
            n177 = Concatenate Strings(w242, " %d %m %y %H.%M.%S" ("time format string (%c)")) -> (w244:string)
            n178 = Build Path(base path=w248, name or relative path=w242) -> (appended path=w275:path)
            n179 = Get Date/Time In Seconds() -> (seconds since 1Jan1904=w271:timestamp)
            n180 = call <vilib>:"Check if File or Folder Exists.vi"("path"=w275) -> ("file or folder exists?"=w274:bool, "dup path"=w273:path)  [unwired: 8 in, 1 out]
            n181 = Format Date/Time String(time format string (%c)=w244, seconds (now)=w271) -> (date/time string=w270:string)  [unwired: 1 in]
            n182 = case shown="False" w274 {
              tunnel: w273 -> [w281 w282]
              tunnel: [w280 w282] -> w272
              frame False {
                n183 = Create Folder(path (use dialog)=w281) -> (created path=w280:path)  [unwired: 2 in, 2 out]
              }
              frame True {
              }
            }
            n184 = Concatenate Strings("P1 CH0, V" ("string"), w237, "P1 CH0 Current, A" ("string"), w237, "Time" ("string"), w237, "455 nm Current Averaged, A" ("string"), w237, "P1 CH1, V" ("string"), w237, "P1 CH1 Current, A" ("string"), w237, "Time" ("string"), w237, "808 nm Current Averaged, A" ("string"), w237, "P2 CH0, V" ("string"), w237, "P2 CH0 Current, A" ("string"), w237, "Time" ("string"), w237, "1550 nm Current Averaged, A" ("string"), w237) -> (w238:string)
            n185 = Concatenate Strings(w270, ".xls" ("string")) -> (w269:string)
            n186 = Build Path(base path=w272, name or relative path=w269) -> (appended path=w268:path)
            n187 = Open/Create/Replace File(file path (use dialog)=w268, operation (0:open)=T6."open or create", access (0:read/write)=enum16{"read/write", "read-only", "write-only"}."read/write") -> (refnum out=w267:refnum<file>)  [unwired: 3 in, 2 out]
            n188 = Concatenate Strings(w238, "455 nm Absolute/Reference" ("string"), w232, "808 nm Absolute/Reference" ("string"), w232, "1550 nm Absolute/Reference" ("string"), w232) -> (w233:string)
            n189 = Set File Position(refnum=w267, from (0:start)=enum16{"start", "end", "current"}."end") -> (refnum out=w262:refnum<file>)  [unwired: 2 in, 1 out]
            n190 = Concatenate Strings(w233, w242, "\t", w233, "Log Remarks" ("string"), "\r\n") -> (w249:string)
            n191 = Format Into String(initial string=w262, w249) -> (resulting string=w247:refnum<file>)  [unwired: 2 in, 1 out]
            n192 = case shown="3" w240 {
              tunnel: w247 -> [w276 w277 w278 w279]
              frame 0, Default {
                "Glass 1 Output File" <- w276
              }
              frame 1 {
                "Glass 2 Output File" <- w277
              }
              frame 2 {
                "Glass 3 Output File" <- w278
              }
              frame 3 {
                "Glass 4 Output File" <- w279
              }
            }
          }
        }
      }
    }
    frame #4 {
      w285 = "\t"
      # "Инициализация файла SEL"
      n193 = local read "Образец №"() -> (w312:string)
      n194 = Build Path(base path="SEL path", name or relative path=w312) -> (appended path=w327:path)
      n195 = Get Date/Time In Seconds() -> (seconds since 1Jan1904=w323:timestamp)
      n196 = call <vilib>:"Check if File or Folder Exists.vi"("path"=w327) -> ("file or folder exists?"=w326:bool, "dup path"=w325:path)  [unwired: 8 in, 1 out]
      n197 = Format Date/Time String(time format string (%c)="SEL %d %m %y %H.%M.%S", seconds (now)=w323) -> (date/time string=w322:string)  [unwired: 1 in]
      n198 = case shown="False" w326 {
        tunnel: w325 -> [w329 w330]
        tunnel: [w328 w330] -> w324
        frame False {
          n199 = Create Folder(path (use dialog)=w329) -> (created path=w328:path)  [unwired: 2 in, 2 out]
        }
        frame True {
        }
      }
      n200 = Concatenate Strings(w322, ".xls" ("string")) -> (w319:string)
      n201 = Build Path(base path=w324, name or relative path=w319) -> (appended path=w316:path)
      n202 = Open/Create/Replace File(file path (use dialog)=w316, operation (0:open)=T6."open or create", access (0:read/write)=enum16{"read/write", "read-only", "write-only"}."read/write") -> (refnum out=w315:refnum<file>)  [unwired: 3 in, 2 out]
      n203 = Set File Position(refnum=w315, from (0:start)=enum16{"start", "end", "current"}."end") -> (refnum out=w296:refnum<file>)  [unwired: 2 in, 1 out]
      n204 = Format Into String(initial string=w296, "Time" ("string"), w285, "P1 CH0, V" ("string"), w285, "P1 CH0_cur, A" ("string"), w285, "P1 CH0_counter" ("string"), w285, "!!!1_0" ("input 7"), w285, "P1 CH1, V" ("string"), w285, "P1 CH1_cur, A" ("string"), w285, "P1 CH1_counter" ("string"), w285, "!!!1_1" ("input 7"), w285, "P1 CH2, V" ("string"), w285, "P1 CH2_cur, A" ("string"), w285, "P1 CH2_counter" ("string"), w285, "!!!1_2" ("input 7"), w285, "P2 CH0, V" ("string"), w285, "P2 CH0_cur, A" ("string"), w285, "P2 CH0_counter" ("string"), w285, "!!!2_0" ("input 7"), w285, "P2 CH1, V" ("string"), w285, "P2 CH1_cur, A" ("string"), w285, "P2 CH1_counter" ("string"), w285, "!!!2_1" ("input 7"), w285, "P2 CH2, V" ("string"), w285, "P2 CH2_cur, A" ("string"), w285, "P2 CH2_counter" ("string"), w285, "!!!2_2" ("input 7"), "\r\n") -> (resulting string=→"SEL output file refnum":refnum<file>)  [unwired: 2 in, 1 out]
    }
    frame #5 {
      # "Инициализация источника"
      n205 = local read "DC Power 1 Status"() -> (w332:bool)
      n206 = local read "DC Power 2 Status"() -> (w331:bool)
      n207 = case shown="True" w332 {
        tunnel: [refnum<k15> refnum ("instrument handle out") w342] -> w336
        tunnel: [errorcluster {"status"=FALSE, "code"=0, "source"=""} ("error out") w341] -> w335
        frame False {
          n208 = property on="Tab DC Power 1" class="TabCtl (strict)"("DisabledEnum"=T7."Disabled and Grayed Out" ("Disabled")) -> ()  [unwired: 2 in, 2 out]
        }
        frame True {
          n209 = property on="Tab DC Power 1" class="TabCtl (strict)"("DisabledEnum"=T7."Enabled" ("Disabled")) -> ()  [unwired: 2 in, 2 out]
          n210 = call <instrlib>:"niDCPower Initialize.vi"("resource name"="DC POWER 1") -> ("error out"=w346:errorcluster, "instrument handle out"=w347:refnum<k15>)  [unwired: 3 in, 6 out]
          n211 = call <instrlib>:"niDCPower Configure Voltage Level.vi"("error in (no error)"=w346, "voltage level"=0.0, "channel name"="0,1", "instrument handle"=w347) -> ("error out"=w341:errorcluster, "instrument handle out"=w342:refnum<k15>)  [unwired: 6 in]
        }
      }
      n212 = case shown="True" w331 {
        tunnel: [refnum<k15> refnum ("instrument handle out") w353] -> w333
        tunnel: [errorcluster {"status"=FALSE, "code"=0, "source"=""} ("error out") w352] -> w334
        frame False {
          n213 = property on="Tab DC Power 2" class="TabCtl (strict)"("DisabledEnum"=T7."Disabled and Grayed Out" ("Disabled")) -> ()  [unwired: 2 in, 2 out]
        }
        frame True {
          n214 = property on="Tab DC Power 2" class="TabCtl (strict)"("DisabledEnum"=T7."Enabled" ("Disabled")) -> ()  [unwired: 2 in, 2 out]
          n215 = call <instrlib>:"niDCPower Initialize.vi"("resource name"="DC POWER 2") -> ("error out"=w357:errorcluster, "instrument handle out"=w358:refnum<k15>)  [unwired: 3 in, 6 out]
          n216 = call <instrlib>:"niDCPower Configure Voltage Level.vi"("error in (no error)"=w357, "voltage level"=0.0, "channel name"="0,1", "instrument handle"=w358) -> ("error out"=w352:errorcluster, "instrument handle out"=w353:refnum<k15>)  [unwired: 6 in]
        }
      }
    }
    frame #6 {
      n217 = local read "NI Scope Status"() -> (w359:bool)
      n218 = case shown="True" w359 {
        tunnel: [refnum<k15> refnum ("instrument handle out") w367] -> w361
        tunnel: [errorcluster {"status"=FALSE, "code"=0, "source"=""} ("error out") w366] -> w360
        frame False {
          n219 = Wait (ms)(milliseconds to wait=u32 1) -> ()  [unwired: 1 out]
          n220 = property on="NI Scope Tab" class="TabCtl (strict)"("DisabledEnum"=T7."Disabled and Grayed Out" ("Disabled")) -> ()  [unwired: 2 in, 2 out]
        }
        frame True {
          n221 = stacked-sequence {
            tunnel: [_ w399] -> w367
            tunnel: [_ w398] -> w366
            frame #0 {
              w378 = "\t"
              # "Инициализация файла SEU"
              n222 = local read "Образец №"() -> (w383:string)
              n223 = Build Path(base path="SEU path", name or relative path=w383) -> (appended path=w393:path)
              n224 = Get Date/Time In Seconds() -> (seconds since 1Jan1904=w389:timestamp)
              n225 = call <vilib>:"Check if File or Folder Exists.vi"("path"=w393) -> ("file or folder exists?"=w392:bool, "dup path"=w391:path)  [unwired: 8 in, 1 out]
              n226 = Format Date/Time String(time format string (%c)="SEU %d %m %y %H.%M.%S", seconds (now)=w389) -> (date/time string=w388:string)  [unwired: 1 in]
              n227 = case shown="True" w392 {
                tunnel: w391 -> [w395 w396]
                tunnel: [w394 w396] -> w390
                frame False {
                  n228 = Create Folder(path (use dialog)=w395) -> (created path=w394:path)  [unwired: 2 in, 2 out]
                }
                frame True {
                }
              }
              n229 = Concatenate Strings(w388, ".xls" ("string")) -> (w387:string)
              n230 = Build Path(base path=w390, name or relative path=w387) -> (appended path=w386:path)
              n231 = Open/Create/Replace File(file path (use dialog)=w386, operation (0:open)=T6."open or create", access (0:read/write)=enum16{"read/write", "read-only", "write-only"}."read/write") -> (refnum out=w385:refnum<file>)  [unwired: 3 in, 2 out]
              n232 = property on="NI Scope Tab" class="TabCtl (strict)"("DisabledEnum"=T7."Enabled" ("Disabled")) -> ()  [unwired: 2 in, 2 out]
              n233 = Set File Position(refnum=w385, from (0:start)=enum16{"start", "end", "current"}."end") -> (refnum out=w382:refnum<file>)  [unwired: 2 in, 1 out]
              n234 = Format Into String(initial string=w382, "Time" ("string"), w378, "Voltage, V" ("string"), w378, "Current, A" ("string"), w378, "SEU counter" ("string"), w378, "!!!" ("input 7"), "\r\n") -> (resulting string=→"SEU output file refnum":refnum<file>)  [unwired: 2 in, 1 out]
            }
            frame #1 {
              w404 = 2 items=["None"=1, "Auto Trigger"=2] ("Triggering:Trigger Modifier")
              w402 = u32 0 items=["1 mega ohm"=0, "50 ohms"=2] ("Input Impedance")
              w400 = FALSE  # Reset Device
              n235 = call <instrlib>:"niScope Initialize.vi"("resource name"="NI Scope", "reset device"=w400, "error in"="NI Scope error in") -> ("instrument handle"=w411:refnum<k15>, "error out"=w410:errorcluster)  [unwired: 11 in]
              n236 = call <instrlib>:"niScope Configure Chan Characteristics.vi"("instrument handle"=w411, "channels"="0" ("Channel Name"), "input impedance"=w402, "maximum input frequency"=20000000.0 ("Maximum Input Frequency"), "error in"=w410) -> ("instrument handle out"=w413:refnum<k15>, "error out"=w409:errorcluster)  [unwired: 9 in]
              n237 = call <instrlib>:"niScope Configure Horizontal Timing.vi"("instrument handle"=w413, "enforce realtime"=TRUE ("Enforce Realtime"), "min sample rate"=250000000.0 ("Min Sample Rate"), "reference position"=50.0 ("Reference\nPosition"), "error in"=w409, "min record length"=1000000 ("Min Record Length")) -> ("instrument handle out"=w412:refnum<k15>, "error out"=w398:errorcluster)  [unwired: 8 in]
              n238 = property on="Property Node" class="niScope"(reference=w412, "Trigger Modifier"=w404) -> (reference out=w399:refnum<k15>)  [unwired: 1 in, 1 out]
            }
          }
        }
      }
    }
    frame #7 {
      # "Инициализация DMM"
      n239 = local read "NI DMM 1 Status"() -> (w422:bool)
      n240 = local read "NI DMM 2 Status"() -> (w421:bool)
      n241 = local read "NI DMM 3 Status"() -> (w417:bool)
      n242 = case shown="True" w417 {
        tunnel: [refnum<k15> refnum ("instrument handle out") w428] -> w415
        tunnel: [errorcluster {"status"=FALSE, "code"=0, "source"=""} ("error out") w429] -> w416
        frame False {
          n243 = property on="NI DMM 3 Tab" class="TabCtl (strict)"("DisabledEnum"=T7."Disabled and Grayed Out" ("Disabled")) -> ()  [unwired: 2 in, 2 out]
        }
        frame True {
          n244 = local read "NI DMM 3 Option Return"() -> (w430:enum32{"Ampermeter button", "Ohmmeter button"})
          n245 = property on="NI DMM 3 Tab" class="TabCtl (strict)"("DisabledEnum"=T7."Enabled" ("Disabled")) -> ()  [unwired: 2 in, 2 out]
          n246 = stacked-sequence {
            tunnel: w430 -> [w431 _]
            tunnel: [_ w485] -> w429
            tunnel: [_ w484] -> w428
            frame #0 {
              n247 = case shown="\"Ampermeter button\", Default" w431 {
                frame "Ampermeter button", Default {
                  # "Инициализация файла SEU"
                  n248 = local read "Образец №"() -> (w447:string)
                  n249 = Build Path(base path="NI DMM 3 Ampermeter path", name or relative path=w447) -> (appended path=w454:path)
                  n250 = Get Date/Time In Seconds() -> (seconds since 1Jan1904=w450:timestamp)
                  n251 = call <vilib>:"Check if File or Folder Exists.vi"("path"=w454) -> ("file or folder exists?"=w453:bool, "dup path"=w452:path)  [unwired: 8 in, 1 out]
                  n252 = Format Date/Time String(time format string (%c)="NI DMM 3 %d %m %y %H.%M.%S", seconds (now)=w450) -> (date/time string=w449:string)  [unwired: 1 in]
                  n253 = case shown="True" w453 {
                    tunnel: w452 -> [w456 w457]
                    tunnel: [w455 w457] -> w451
                    frame False {
                      n254 = Create Folder(path (use dialog)=w456) -> (created path=w455:path)  [unwired: 2 in, 2 out]
                    }
                    frame True {
                    }
                  }
                  n255 = Concatenate Strings(w449, ".xls" ("string")) -> (w448:string)
                  n256 = Build Path(base path=w451, name or relative path=w448) -> (appended path=w433:path)
                  n257 = Open/Create/Replace File(file path (use dialog)=w433, operation (0:open)=T6."open or create", access (0:read/write)=enum16{"read/write", "read-only", "write-only"}."read/write") -> (refnum out=w444:refnum<file>)  [unwired: 3 in, 2 out]
                  n258 = Set File Position(refnum=w444, from (0:start)=enum16{"start", "end", "current"}."end") -> (refnum out=w436:refnum<file>)  [unwired: 2 in, 1 out]
                  n259 = Format Into String(initial string=w436, "Time" ("string"), "\t", "Current, A" ("string"), "\r\n") -> (resulting string=→"NI DMM 3 Current output file":refnum<file>)  [unwired: 2 in, 1 out]
                  n260 = local write "NI DMM 3 Tab"(enum32{"Amp", "Ohm", "System Panel"}."Amp" ("NI DMM 2 Tab")) -> ()
                }
                frame "Ohmmeter button" {
                  n261 = local read "Образец №"() -> (w473:string)
                  n262 = Build Path(base path="NI DMM 3 Ohmmeter path", name or relative path=w473) -> (appended path=w480:path)
                  n263 = Get Date/Time In Seconds() -> (seconds since 1Jan1904=w476:timestamp)
                  n264 = call <vilib>:"Check if File or Folder Exists.vi"("path"=w480) -> ("file or folder exists?"=w479:bool, "dup path"=w478:path)  [unwired: 8 in, 1 out]
                  n265 = Format Date/Time String(time format string (%c)="NI DMM 3 %d %m %y %H.%M.%S", seconds (now)=w476) -> (date/time string=w475:string)  [unwired: 1 in]
                  n266 = case shown="True" w479 {
                    tunnel: w478 -> [w482 w483]
                    tunnel: [w481 w483] -> w477
                    frame False {
                      n267 = Create Folder(path (use dialog)=w482) -> (created path=w481:path)  [unwired: 2 in, 2 out]
                    }
                    frame True {
                    }
                  }
                  n268 = Concatenate Strings(w475, ".xls" ("string")) -> (w474:string)
                  n269 = Build Path(base path=w477, name or relative path=w474) -> (appended path=w459:path)
                  n270 = Open/Create/Replace File(file path (use dialog)=w459, operation (0:open)=T6."open or create", access (0:read/write)=enum16{"read/write", "read-only", "write-only"}."read/write") -> (refnum out=w470:refnum<file>)  [unwired: 3 in, 2 out]
                  n271 = Set File Position(refnum=w470, from (0:start)=enum16{"start", "end", "current"}."end") -> (refnum out=w462:refnum<file>)  [unwired: 2 in, 1 out]
                  n272 = Format Into String(initial string=w462, "Time" ("string"), "\t", "Current, A" ("string"), "\r\n") -> (resulting string=→"NI DMM 3 Resistance output file":refnum<file>)  [unwired: 2 in, 1 out]
                  n273 = local write "NI DMM 3 Tab"(enum32{"Amp", "Ohm", "System Panel"}."Ohm" ("NI DMM 2 Tab")) -> ()
                }
              }
            }
            frame #1 {
              n274 = call <instrlib>:"niDMM Initialize.vi"("error in (no error)"="NI DMM 3 error in", "Instrument Descriptor"="NI DMM 3") -> ("error out"=w485:errorcluster, "instrument handle out"=w484:refnum<k15>)  [unwired: 8 in]
            }
          }
        }
      }
      "NI DMM 3 error out" <- w416
      n275 = case shown="True" w422 {
        tunnel: [refnum<k15> refnum ("instrument handle out") w556] -> w420
        tunnel: [errorcluster {"status"=FALSE, "code"=0, "source"=""} ("error out") w555] -> w419
        frame False {
          n276 = property on="NI DMM 1 Tab" class="TabCtl (strict)"("DisabledEnum"=T7."Disabled and Grayed Out" ("Disabled")) -> ()  [unwired: 2 in, 2 out]
        }
        frame True {
          n277 = local read "NI DMM 1 Option Return"() -> (w558:enum32{"Ampermeter button", "Ohmmeter button"})
          n278 = property on="NI DMM 1 Tab" class="TabCtl (strict)"("DisabledEnum"=T7."Enabled" ("Disabled")) -> ()  [unwired: 2 in, 2 out]
          n279 = stacked-sequence {
            tunnel: w558 -> [w559 _]
            tunnel: [_ w613] -> w556
            tunnel: [_ w612] -> w555
            frame #0 {
              n280 = case shown="\"Ampermeter button\", Default" w559 {
                frame "Ampermeter button", Default {
                  n281 = local read "Образец №"() -> (w575:string)
                  n282 = Build Path(base path="NI DMM 1 Ampermeter path", name or relative path=w575) -> (appended path=w582:path)
                  n283 = Get Date/Time In Seconds() -> (seconds since 1Jan1904=w578:timestamp)
                  n284 = call <vilib>:"Check if File or Folder Exists.vi"("path"=w582) -> ("file or folder exists?"=w581:bool, "dup path"=w580:path)  [unwired: 8 in, 1 out]
                  n285 = Format Date/Time String(time format string (%c)="NI DMM 1 %d %m %y %H.%M.%S", seconds (now)=w578) -> (date/time string=w577:string)  [unwired: 1 in]
                  n286 = case shown="True" w581 {
                    tunnel: w580 -> [w584 w585]
                    tunnel: [w583 w585] -> w579
                    frame False {
                      n287 = Create Folder(path (use dialog)=w584) -> (created path=w583:path)  [unwired: 2 in, 2 out]
                    }
                    frame True {
                    }
                  }
                  n288 = Concatenate Strings(w577, ".xls" ("string")) -> (w576:string)
                  n289 = Build Path(base path=w579, name or relative path=w576) -> (appended path=w561:path)
                  n290 = Open/Create/Replace File(file path (use dialog)=w561, operation (0:open)=T6."open or create", access (0:read/write)=enum16{"read/write", "read-only", "write-only"}."read/write") -> (refnum out=w572:refnum<file>)  [unwired: 3 in, 2 out]
                  n291 = local write "NI DMM 1 Tab"(enum32{"Amp", "Ohm", "System Panel"}."Amp" ("NI DMM 1 Tab")) -> ()
                  n292 = Set File Position(refnum=w572, from (0:start)=enum16{"start", "end", "current"}."end") -> (refnum out=w564:refnum<file>)  [unwired: 2 in, 1 out]
                  n293 = Format Into String(initial string=w564, "Time" ("string"), "\t", "Current, A" ("string"), "\r\n") -> (resulting string=→"NI DMM 1 Current output file":refnum<file>)  [unwired: 2 in, 1 out]
                }
                frame "Ohmmeter button" {
                  # "Инициализация файла SEU"
                  n294 = local read "Образец №"() -> (w601:string)
                  n295 = Build Path(base path="NI DMM 1 Ohmmeter path", name or relative path=w601) -> (appended path=w608:path)
                  n296 = Get Date/Time In Seconds() -> (seconds since 1Jan1904=w604:timestamp)
                  n297 = call <vilib>:"Check if File or Folder Exists.vi"("path"=w608) -> ("file or folder exists?"=w607:bool, "dup path"=w606:path)  [unwired: 8 in, 1 out]
                  n298 = Format Date/Time String(time format string (%c)="NI DMM 1 %d %m %y %H.%M.%S", seconds (now)=w604) -> (date/time string=w603:string)  [unwired: 1 in]
                  n299 = case shown="False" w607 {
                    tunnel: w606 -> [w610 w611]
                    tunnel: [w609 w611] -> w605
                    frame False {
                      n300 = Create Folder(path (use dialog)=w610) -> (created path=w609:path)  [unwired: 2 in, 2 out]
                    }
                    frame True {
                    }
                  }
                  n301 = Concatenate Strings(w603, ".xls" ("string")) -> (w602:string)
                  n302 = Build Path(base path=w605, name or relative path=w602) -> (appended path=w587:path)
                  n303 = Open/Create/Replace File(file path (use dialog)=w587, operation (0:open)=T6."open or create", access (0:read/write)=enum16{"read/write", "read-only", "write-only"}."read/write") -> (refnum out=w598:refnum<file>)  [unwired: 3 in, 2 out]
                  n304 = local write "NI DMM 1 Tab"(enum32{"Amp", "Ohm", "System Panel"}."Ohm" ("NI DMM 1 Tab")) -> ()
                  n305 = Set File Position(refnum=w598, from (0:start)=enum16{"start", "end", "current"}."end") -> (refnum out=w590:refnum<file>)  [unwired: 2 in, 1 out]
                  n306 = Format Into String(initial string=w590, "Time" ("string"), "\t", "Current, A" ("string"), "\r\n") -> (resulting string=→"NI DMM 1 Resistance output file":refnum<file>)  [unwired: 2 in, 1 out]
                }
              }
            }
            frame #1 {
              n307 = call <instrlib>:"niDMM Initialize.vi"("error in (no error)"="NI DMM 1 error in", "Instrument Descriptor"="NI DMM 1") -> ("error out"=w612:errorcluster, "instrument handle out"=w613:refnum<k15>)  [unwired: 8 in]
            }
          }
        }
      }
      "NI DMM 1 error out" <- w419
      n308 = case shown="True" w421 {
        tunnel: [refnum<k15> refnum ("instrument handle out") w491] -> w423
        tunnel: [errorcluster {"status"=FALSE, "code"=0, "source"=""} ("error out") w492] -> w418
        frame False {
          n309 = property on="NI DMM 2 Tab" class="TabCtl (strict)"("DisabledEnum"=T7."Disabled and Grayed Out" ("Disabled")) -> ()  [unwired: 2 in, 2 out]
        }
        frame True {
          n310 = local read "NI DMM 2 Option Return"() -> (w494:enum32{"Ampermeter button", "Ohmmeter button"})
          n311 = property on="NI DMM 2 Tab" class="TabCtl (strict)"("DisabledEnum"=T7."Enabled" ("Disabled")) -> ()  [unwired: 2 in, 2 out]
          n312 = stacked-sequence {
            tunnel: w494 -> [w495 _]
            tunnel: [_ w549] -> w492
            tunnel: [_ w548] -> w491
            frame #0 {
              n313 = case shown="\"Ampermeter button\", Default" w495 {
                frame "Ampermeter button", Default {
                  n314 = local read "Образец №"() -> (w511:string)
                  n315 = Build Path(base path="NI DMM 2 Ampermeter path", name or relative path=w511) -> (appended path=w518:path)
                  n316 = Get Date/Time In Seconds() -> (seconds since 1Jan1904=w514:timestamp)
                  n317 = call <vilib>:"Check if File or Folder Exists.vi"("path"=w518) -> ("file or folder exists?"=w517:bool, "dup path"=w516:path)  [unwired: 8 in, 1 out]
                  n318 = Format Date/Time String(time format string (%c)="NI DMM 2 %d %m %y %H.%M.%S", seconds (now)=w514) -> (date/time string=w513:string)  [unwired: 1 in]
                  n319 = case shown="True" w517 {
                    tunnel: w516 -> [w520 w521]
                    tunnel: [w519 w521] -> w515
                    frame False {
                      n320 = Create Folder(path (use dialog)=w520) -> (created path=w519:path)  [unwired: 2 in, 2 out]
                    }
                    frame True {
                    }
                  }
                  n321 = Concatenate Strings(w513, ".xls" ("string")) -> (w512:string)
                  n322 = Build Path(base path=w515, name or relative path=w512) -> (appended path=w497:path)
                  n323 = Open/Create/Replace File(file path (use dialog)=w497, operation (0:open)=T6."open or create", access (0:read/write)=enum16{"read/write", "read-only", "write-only"}."read/write") -> (refnum out=w508:refnum<file>)  [unwired: 3 in, 2 out]
                  n324 = Set File Position(refnum=w508, from (0:start)=enum16{"start", "end", "current"}."end") -> (refnum out=w500:refnum<file>)  [unwired: 2 in, 1 out]
                  n325 = Format Into String(initial string=w500, "Time" ("string"), "\t", "Current, A" ("string"), "\r\n") -> (resulting string=→"NI DMM 2 Current output file":refnum<file>)  [unwired: 2 in, 1 out]
                  n326 = local write "NI DMM 2 Tab"(enum32{"Amp", "Ohm", "System Panel"}."Amp" ("NI DMM 2 Tab")) -> ()
                }
                frame "Ohmmeter button" {
                  # "Инициализация файла SEU"
                  n327 = local read "Образец №"() -> (w537:string)
                  n328 = Build Path(base path="NI DMM 2 Ohmmeter path", name or relative path=w537) -> (appended path=w544:path)
                  n329 = Get Date/Time In Seconds() -> (seconds since 1Jan1904=w540:timestamp)
                  n330 = call <vilib>:"Check if File or Folder Exists.vi"("path"=w544) -> ("file or folder exists?"=w543:bool, "dup path"=w542:path)  [unwired: 8 in, 1 out]
                  n331 = Format Date/Time String(time format string (%c)="NI DMM 2 %d %m %y %H.%M.%S", seconds (now)=w540) -> (date/time string=w539:string)  [unwired: 1 in]
                  n332 = case shown="True" w543 {
                    tunnel: w542 -> [w546 w547]
                    tunnel: [w545 w547] -> w541
                    frame False {
                      n333 = Create Folder(path (use dialog)=w546) -> (created path=w545:path)  [unwired: 2 in, 2 out]
                    }
                    frame True {
                    }
                  }
                  n334 = Concatenate Strings(w539, ".xls" ("string")) -> (w538:string)
                  n335 = Build Path(base path=w541, name or relative path=w538) -> (appended path=w523:path)
                  n336 = Open/Create/Replace File(file path (use dialog)=w523, operation (0:open)=T6."open or create", access (0:read/write)=enum16{"read/write", "read-only", "write-only"}."read/write") -> (refnum out=w534:refnum<file>)  [unwired: 3 in, 2 out]
                  n337 = Set File Position(refnum=w534, from (0:start)=enum16{"start", "end", "current"}."end") -> (refnum out=w526:refnum<file>)  [unwired: 2 in, 1 out]
                  n338 = Format Into String(initial string=w526, "Time" ("string"), "\t", "Current, A" ("string"), "\r\n") -> (resulting string=→"NI DMM 2 Resistance output file":refnum<file>)  [unwired: 2 in, 1 out]
                  n339 = local write "NI DMM 2 Tab"(enum32{"Amp", "Ohm", "System Panel"}."Ohm" ("NI DMM 2 Tab")) -> ()
                }
              }
            }
            frame #1 {
              n340 = call <instrlib>:"niDMM Initialize.vi"("error in (no error)"="NI DMM 2 error in", "Instrument Descriptor"="NI DMM 2") -> ("error out"=w549:errorcluster, "instrument handle out"=w548:refnum<k15>)  [unwired: 8 in]
            }
          }
        }
      }
      "NI DMM 2 error out" <- w418
    }
    frame #8 {
      n341 = local read "Ophir 1 Status"() -> (w616:bool)
      n342 = case shown="True" w616 {
        frame False {
          n343 = property on="Ophir 1 Tab" class="TabCtl (strict)"("DisabledEnum"=T7."Disabled and Grayed Out" ("Disabled")) -> ()  [unwired: 2 in, 2 out]
        }
        frame True {
          n344 = call "Ophir InitCom.vi"("GPIB Address (default 10)"="Ophir 1 GPIB Address (10)", "Communication (default USB 0)"="Ophir 1 Select Communication Protocol", "USB Channel number (default 0)"="Ophir 1 usb channel", "Port Number (default 2)"="Ophir 1 Port Number (default 2)", "error in (no error)"="Ophir 1 error in (no error)", "Baud Rate (3:9600)"="Ophir 1 Baud Rate (3:9600)") -> ("dup Visa Session"=w624:refnum<visa-resource-name>, "error out"=w623:errorcluster)  [unwired: 1 out]
          n345 = call "Ophir InstrInfo.vi"("Visa Session"=w624, "error in (no error)"=w623) -> ("dup Visa Session"=w637:refnum<visa-resource-name>, "Instrument Info"=w633:string, "error out"=w635:errorcluster)
          n346 = call "Ophir HeadInfo.vi"("Visa Session"=w637, "error in (no error)"=w635) -> ("error out"=w634:errorcluster, "dup Visa Session"=w636:refnum<visa-resource-name>, "Head Info"=w632:string)  [unwired: 6 out]
          n347 = call "Ophir InfoStrings.vi"("error in (no error)"=w634, "Head Info"=w632, "Instrument Info"=w633) -> ("error out"=w631:errorcluster, "Strings Array"=w630:string[])
          n348 = property on="Ophir 1 Info" class="Ring (strict)"("Strings []"=w630) -> ()  [unwired: 2 in, 2 out]
          n349 = property on="Ophir 1 Tab" class="TabCtl (strict)"("DisabledEnum"=T7."Enabled" ("Disabled")) -> ()  [unwired: 2 in, 2 out]
          n350 = call "Ophir ConfigDevice.vi"("Visa Session"=w636, "Measure Choice (0:Power)"=u16 0, "error in (no error)"=w631) -> ("dup Visa Session"=→"Ophir 1 dup Visa Session":refnum<visa-resource-name>, "OK ?"=→"Ophir 1 Initialization":bool, "error out"=→"Ophir 1 error out":errorcluster)  [unwired: 1 out]
        }
      }
    }
    frame #9 {
      n351 = local read "Ophir 2 Status"() -> (w639:bool)
      n352 = case shown="True" w639 {
        frame False {
          n353 = property on="Ophir 2 Tab" class="TabCtl (strict)"("DisabledEnum"=T7."Disabled and Grayed Out" ("Disabled")) -> ()  [unwired: 2 in, 2 out]
        }
        frame True {
          n354 = call "Ophir InitCom.vi"("GPIB Address (default 10)"="Ophir 2 GPIB Address (10)", "Communication (default USB 0)"="Ophir 2 Select Communication Protocol", "USB Channel number (default 0)"="Ophir 2 usb channel", "Port Number (default 2)"="Ophir 2 Port Number (default 2)", "error in (no error)"="Ophir 2 error in (no error)", "Baud Rate (3:9600)"="Ophir 2 Baud Rate (3:9600)") -> ("dup Visa Session"=w647:refnum<visa-resource-name>, "error out"=w646:errorcluster)  [unwired: 1 out]
          n355 = call "Ophir InstrInfo.vi"("Visa Session"=w647, "error in (no error)"=w646) -> ("dup Visa Session"=w660:refnum<visa-resource-name>, "Instrument Info"=w656:string, "error out"=w658:errorcluster)
          n356 = call "Ophir HeadInfo.vi"("Visa Session"=w660, "error in (no error)"=w658) -> ("error out"=w657:errorcluster, "dup Visa Session"=w659:refnum<visa-resource-name>, "Head Info"=w655:string)  [unwired: 6 out]
          n357 = call "Ophir InfoStrings.vi"("error in (no error)"=w657, "Head Info"=w655, "Instrument Info"=w656) -> ("error out"=w654:errorcluster, "Strings Array"=w653:string[])
          n358 = property on="Ophir 2 Info" class="Ring (strict)"("Strings []"=w653) -> ()  [unwired: 2 in, 2 out]
          n359 = property on="Ophir 2 Tab" class="TabCtl (strict)"("DisabledEnum"=T7."Enabled" ("Disabled")) -> ()  [unwired: 2 in, 2 out]
          n360 = call "Ophir ConfigDevice.vi"("Visa Session"=w659, "Measure Choice (0:Power)"=u16 0, "error in (no error)"=w654) -> ("dup Visa Session"=→"Ophir 2 dup Visa Session":refnum<visa-resource-name>, "OK ?"=→"Ophir 2 Initialization":bool, "error out"=→"Ophir 2 error out":errorcluster)  [unwired: 1 out]
        }
      }
    }
    frame #10 {
      n361 = local read "Stepper Motor Status"() -> (w665:bool)
      n362 = case shown="True" w665 {
        tunnel: [_ w674] -> w664
        tunnel: [_ w673] -> w663
        tunnel: [_ w672] -> w662
        frame False {
          n363 = property on="Stepper Motor Control" class="TabCtl (strict)"("DisabledEnum"=T7."Disabled and Grayed Out" ("Disabled")) -> ()  [unwired: 2 in, 2 out]
          n364 = property on="Table Tab" class="TabCtl (strict)"("DisabledEnum"=T7."Disabled and Grayed Out" ("Disabled")) -> ()  [unwired: 2 in, 2 out]
        }
        frame True {
          n365 = property on="Stepper Motor Control" class="TabCtl (strict)"("DisabledEnum"=T7."Enabled" ("Disabled")) -> ()  [unwired: 2 in, 2 out]
          n366 = constructor class="NetTcpUrl"("host"="localhost", "port"=u32 8001, "urlPath"="AmateurStepperMotorInternal") -> (reference out=w685:refnum<k24>)  [unwired: 3 in, 5 out]
          n367 = constructor class="AmateurStepperMotorWcfClient"("serviceUrl"=w685) -> (reference out=w686:refnum<k24>)  [unwired: 3 in, 3 out]
          n368 = invoke class="AmateurStepperMotorWcfClient" method="RefreshParameters"(reference=w686) -> (reference out=w675:refnum<k24>)  [unwired: 2 in, 2 out]
          n369 = property on="Table Tab" class="TabCtl (strict)"("DisabledEnum"=T7."Enabled" ("Disabled")) -> ()  [unwired: 2 in, 2 out]
          n370 = property on="Glass Meas" class="Bool (strict)"("DisabledEnum"=T7."Enabled" ("Disabled")) -> ()  [unwired: 2 in, 2 out]
          n371 = property on="Погнали!" class="Bool (strict)"("DisabledEnum"=T7."Enabled" ("Disabled")) -> ()  [unwired: 2 in, 2 out]
          n372 = property class="AmateurStepperMotorWcfClient"(reference=w675, "Speed"="Speed", "StepDivisor"="StepDivisor", "StepMultiplicationFactor"="StepMultiplicationFactor", "AccelerationTime"=0.5, "DecelerationTime"=0.5, "HoldOn"=FALSE) -> (reference out=w674:refnum<k24>, "Position"=w673:dbl, "PositioningPrecision"=w672:dbl)  [unwired: 1 in, 1 out]
        }
      }
    }
    frame #11 {
      w687 = TRUE ("Boolean")
      "Ready Status" <- w687
    }
  }
  n373 = case shown="True" w20 {
    tunnel: w19 -> [_ w693]
    tunnel: w18 -> [_ w692]
    tunnel: w17 -> [_ w691]
    tunnel: w10 -> [_ _]
    frame False {
    }
    frame True {
      n374 = flat-sequence {
        frame #0 {
          n375 = local read "WL 455 Ref"() -> (w714:dbl)
          n376 = local read "WL 808 Ref"() -> (w713:dbl)
          n377 = local read "WL 1550 Ref"() -> (w712:dbl)
          n378 = while {
            shift-right: ["Save Glass Log Data"] -> _
            shift-left: FALSE ("Погнали!") -> [w724]
            shift-right: [w721] -> _
            shift-left: w714 -> [w717]
            shift-right: [w720] -> _
            shift-left: w713 -> [w718]
            shift-right: [w719] -> _
            shift-left: w712 -> [w716]
            stop <- w722 stop-if-true
            n379 = Wait (ms)(milliseconds to wait=u32 1) -> ()  [unwired: 1 out]
            n380 = Greater?(x="Save Glass Log Data", y=w724) -> (0:w725:bool)
            n381 = case shown="True" w725 {
              tunnel: [w729 w738] -> w721
              tunnel: [w728 w737] -> w720
              tunnel: [w727 w736] -> w719
              tunnel: w718 -> [w728 w735]
              tunnel: w717 -> [w729 w734]
              tunnel: w716 -> [w727 w733]
              frame False {
              }
              frame True {
                n382 = flat-sequence {
                  tunnel: w734 -> [w746]
                  tunnel: w735 -> [w745]
                  tunnel: w733 -> [w744]
                  tunnel: [w742] -> w732
                  tunnel: [w741] -> w731
                  tunnel: [w740] -> w730
                  tunnel: [w935] -> w738
                  tunnel: [w934] -> w737
                  tunnel: [w933] -> w736
                  tunnel: w732 -> [w935]
                  tunnel: w731 -> [w934]
                  tunnel: w730 -> [w933]
                  frame #0 {
                    "Save Glass Log Done" <- FALSE ("Save Glass Log Done")
                  }
                  frame #1 {
                    n383 = local read "Glass Meas Cycle Running"() -> (w747:bool)
                    n384 = case shown="True" w747 {
                      tunnel: w746 -> [w754 w799]
                      tunnel: w745 -> [w753 w798]
                      tunnel: w744 -> [w752 w797]
                      tunnel: "Set Last Meas As Ref" -> [w751 _]
                      tunnel: [w750 w799] -> w742
                      tunnel: [w749 w798] -> w741
                      tunnel: [w748 w797] -> w740
                      frame False {
                        n385 = local read "WL-i"() -> (w755:i32)
                        n386 = case shown="False" w751 {
                          tunnel: w754 -> [_ w768]
                          tunnel: w753 -> [_ w767]
                          tunnel: w752 -> [_ w766]
                          tunnel: [w765 w768] -> w750
                          tunnel: [w764 w767] -> w749
                          tunnel: [w763 w766] -> w748
                          frame False {
                            n387 = local read "WL 455"() -> (w765:dbl)
                            n388 = local read "WL 808"() -> (w764:dbl)
                            n389 = local read "WL 1550"() -> (w763:dbl)
                          }
                          frame True {
                            n390 = local write "WL 455 Ref"(w768) -> ()
                            n391 = local write "WL 808 Ref"(w767) -> ()
                            n392 = local write "WL 1550 Ref"(w766) -> ()
                          }
                        }
                        n393 = Wait (ms)(milliseconds to wait=u32 5) -> ()  [unwired: 1 out]
                        n394 = local read "Single Meas Output File"() -> (w759:refnum<file>)
                        n395 = local read "CH Data String"() -> (w760:string)
                        n396 = local read "All Cur Data String"() -> (w761:string)
                        n397 = local read "Meas Time String"() -> (w762:string)
                        n398 = local read "Av Cur Data String"() -> (w757:string)
                        n399 = case shown="0, Default" w755 {
                          tunnel: [w771 w777 w792] -> w756
                          tunnel: w757 -> [w771 w777 w786]
                          frame 0, Default {
                            n400 = local read "WL 455 Ref"() -> (w769:dbl)
                            n401 = local read "WL 455"() -> (w772:dbl)
                            n402 = Divide(x=w772, y=w769) -> (x/y=w774:dbl)
                            n403 = Number To Fractional String(number=w774, precision (6)=i16 3) -> (F-format string=w770:string)  [unwired: 2 in]
                            n404 = local write "WL 455 Absolute/Reference"(w770) -> ()
                          }
                          frame 1 {
                            n405 = local read "WL 808 Ref"() -> (w775:dbl)
                            n406 = local read "WL 808"() -> (w780:dbl)
                            n407 = Divide(x=w780, y=w775) -> (x/y=w779:dbl)
                            n408 = Number To Fractional String(number=w779, precision (6)=i16 3) -> (F-format string=w776:string)  [unwired: 2 in]
                            n409 = local write "WL 808 Absolute/Reference"(w776) -> ()
                          }
                          frame 2 {
                            w783 = "\t"
                            n410 = local read "Add Log Remark"() -> (w784:bool)
                            n411 = case shown="True" w784 {
                              tunnel: ["\r\n" w796] -> w782
                              frame False {
                              }
                              frame True {
                                n412 = local read "Log Remark"() -> (w794:string)
                                n413 = Concatenate Strings(w794, "\r\n") -> (w796:string)
                              }
                            }
                            n414 = local read "WL 455 Absolute/Reference"() -> (w788:string)
                            n415 = local read "WL 808 Absolute/Reference"() -> (w787:string)
                            n416 = local read "WL 1550 Ref"() -> (w781:dbl)
                            n417 = local read "WL 1550"() -> (w791:dbl)
                            n418 = Divide(x=w791, y=w781) -> (x/y=w790:dbl)
                            n419 = Number To Fractional String(number=w790, precision (6)=i16 3) -> (F-format string=w785:string)  [unwired: 2 in]
                            n420 = Concatenate Strings(w786, w788, w783, w787, w783, w785, w783, w782) -> (w792:string)
                            n421 = local write "WL 1550 Absolute/Reference"(w785) -> ()
                          }
                        }
                        n422 = Format Into String(initial string=w759, w760, w761, w762, w756) -> ()  [unwired: 2 in, 2 out]
                      }
                      frame True {
                        n423 = local read "WL-i"() -> (w804:i32)
                        n424 = local read "Куда едем?"() -> (w803:T1)
                        n425 = Wait (ms)(milliseconds to wait=u32 1) -> ()  [unwired: 1 out]
                        n426 = Equal?(x=w803, y=T1."Калибровка") -> (x = y?=w802:bool)
                        n427 = case shown="False" w802 {
                          tunnel: w804 -> [w805 w885]
                          tunnel: w803 -> [w806 _]
                          frame False {
                            n428 = stacked-sequence {
                              tunnel: w806 -> [w809 w846]
                              tunnel: w805 -> [w808 w847]
                              frame #0 {
                                n429 = case shown="2" w808 {
                                tunnel: [w823 w829 w841] -> w814
                                tunnel: [w820 w824 w833] -> w807
                                frame 0, Default {
                                n430 = local read "Av Cur Data String"() -> (w823:string)
                                n431 = local read "WL 455 Ref"() -> (w818:dbl)
                                n432 = local read "WL 455"() -> (w819:dbl)
                                n433 = Divide(x=w819, y=w818) -> (x/y=w822:dbl)
                                n434 = Number To Fractional String(number=w822, precision (6)=i16 3) -> (F-format string=w820:string)  [unwired: 2 in]
                                "WL 455 Absolute/Reference" <- w820
                                }
                                frame 1 {
                                n435 = local read "Av Cur Data String"() -> (w829:string)
                                n436 = local read "WL 808"() -> (w828:dbl)
                                n437 = local read "WL 808 Ref"() -> (w827:dbl)
                                n438 = Divide(x=w828, y=w827) -> (x/y=w826:dbl)
                                n439 = Number To Fractional String(number=w826, precision (6)=i16 3) -> (F-format string=w824:string)  [unwired: 2 in]
                                "WL 808 Absolute/Reference" <- w824
                                }
                                frame 2 {
                                w832 = "\t"
                                n440 = local read "Add Log Remark"() -> (w830:bool)
                                n441 = local read "Av Cur Data String"() -> (w836:string)
                                n442 = local read "WL 455 Absolute/Reference"() -> (w835:string)
                                n443 = local read "WL 808 Absolute/Reference"() -> (w834:string)
                                n444 = case shown="True" w830 {
                                tunnel: ["\r\n" w845] -> w831
                                frame False {
                                }
                                frame True {
                                n445 = local read "Log Remark"() -> (w843:string)
                                n446 = Concatenate Strings(w843, "\r\n") -> (w845:string)
                                }
                                }
                                n447 = local read "WL 1550 Ref"() -> (w839:dbl)
                                n448 = local read "WL 1550"() -> (w840:dbl)
                                n449 = Divide(x=w840, y=w839) -> (x/y=w838:dbl)
                                n450 = Number To Fractional String(number=w838, precision (6)=i16 3) -> (F-format string=w833:string)  [unwired: 2 in]
                                "WL 1550 Absolute/Reference" <- w833
                                n451 = Concatenate Strings(w836, w835, w832, w834, w832, w833, w832, w831) -> (w841:string)
                                }
                                }
                                n452 = local read "CH Data String"() -> (w817:string)
                                n453 = local read "Meas Time String"() -> (w816:string)
                                n454 = local read "Glass Meas Path"() -> (w815:refnum<file>)
                                n455 = Format Into String(initial string=w815, w817, w816, w814) -> ()  [unwired: 2 in, 2 out]
                                n456 = To Long Integer(number=w809) -> (32bit integer=w811:i32)
                                n457 = Increment(x=w808) -> (x+1=w810:i32)
                                n458 = Replace Array Subset(array="Glass Table", new element=w807, index (row)=w811, index (col)=w810) -> (w812:string[][])
                                n459 = local write "Glass Table"(w812) -> ()
                              }
                              frame #1 {
                                n460 = local read "Av Cur Data String"() -> (w849:string)
                                n461 = case shown="2" w847 {
                                tunnel: w846 -> [_ _ w864]
                                tunnel: [w854 w855 w863] -> w848
                                tunnel: w849 -> [w854 w855 w859]
                                frame 0, Default {
                                }
                                frame 1 {
                                }
                                frame 2 {
                                w856 = "\t"
                                n462 = local read "WL 1550 Absolute/Reference"() -> (w862:string)
                                n463 = local read "WL 455 Absolute/Reference"() -> (w860:string)
                                n464 = local read "WL 808 Absolute/Reference"() -> (w861:string)
                                n465 = Equal?(x=w864, y=T1."Четвертое стекло") -> (x = y?=w866:bool)
                                n466 = case shown="True" w866 {
                                tunnel: ["\t" w870] -> w865
                                frame False {
                                }
                                frame True {
                                n467 = case shown="True" "Add Log Remark" {
                                selector: "Add Log Remark" -> [_ w875]
                                tunnel: ["\r\n" w876] -> w870
                                tunnel: [w872 w874] -> w869
                                frame False {
                                n468 = local read "Add Log Remark"() -> (w872:bool)
                                }
                                frame True {
                                n469 = Not(x=w875) -> (.not. x?=w874:bool)
                                n470 = Concatenate Strings("Log Remark", "\r\n") -> (w876:string)
                                }
                                }
                                n471 = local write "Add Log Remark"(w869) -> ()
                                }
                                }
                                n472 = Concatenate Strings(w860, w856, w861, w856, w862, w856) -> (w858:string)
                                n473 = Concatenate Strings(w859, w858) -> (w857:string)
                                n474 = Concatenate Strings(w857, w865) -> (w863:string)
                                }
                                }
                                n475 = local read "Glass Full Log Output File"() -> (w852:refnum<file>)
                                n476 = local read "CH Data String"() -> (w850:string)
                                n477 = local read "All Cur Data String"() -> (w851:string)
                                n478 = local read "Meas Time String"() -> (w853:string)
                                n479 = Format Into String(initial string=w852, w850, w851, w853, w848) -> ()  [unwired: 2 in, 2 out]
                              }
                            }
                          }
                          frame True {
                            n480 = local read "CH Data String"() -> (w893:string)
                            n481 = local read "Meas Time String"() -> (w892:string)
                            n482 = local read "Glass 1 Output File"() -> (w891:refnum<file>)
                            n483 = local read "Glass 2 Output File"() -> (w890:refnum<file>)
                            n484 = local read "Glass 3 Output File"() -> (w889:refnum<file>)
                            n485 = local read "Glass 4 Output File"() -> (w888:refnum<file>)
                            n486 = local read "Glass Full Log Output File"() -> (w883:refnum<file>)
                            n487 = local read "CH Data String"() -> (w881:string)
                            n488 = local read "All Cur Data String"() -> (w882:string)
                            n489 = local read "Meas Time String"() -> (w884:string)
                            n490 = local read "Av Cur Data String"() -> (w880:string)
                            n491 = case shown="0, Default" w885 {
                              tunnel: [w897 w908 w916] -> w886
                              tunnel: w880 -> [w895 w907 w917]
                              tunnel: [w895 w907 w916] -> w879
                              frame 0, Default {
                                n492 = local read "Av Cur Data String"() -> (w897:string)
                                n493 = flat-sequence {
                                tunnel: [w898] -> w896
                                tunnel: w896 -> [w904]
                                tunnel: [w900] -> w894
                                frame #0 {
                                n494 = local read "WL 455 Ref"() -> (w898:dbl)
                                n495 = Wait (ms)(milliseconds to wait=u32 1) -> ()  [unwired: 1 out]
                                }
                                frame #1 {
                                n496 = local read "WL 455"() -> (w903:dbl)
                                "WL 455 Ref" <- w903
                                n497 = Divide(x=w904, y=w903) -> (x/y=w901:dbl)
                                n498 = Number To Fractional String(number=w901, precision (6)=i16 3) -> (F-format string=w900:string)  [unwired: 2 in]
                                }
                                }
                                n499 = local write "WL 455 Absolute/Reference"(w894) -> ()
                              }
                              frame 1 {
                                n500 = local read "Av Cur Data String"() -> (w908:string)
                                n501 = flat-sequence {
                                tunnel: [w909] -> w906
                                tunnel: w906 -> [w913]
                                tunnel: [w911] -> w905
                                frame #0 {
                                n502 = local read "WL 808 Ref"() -> (w909:dbl)
                                n503 = Wait (ms)(milliseconds to wait=u32 1) -> ()  [unwired: 1 out]
                                }
                                frame #1 {
                                n504 = local read "WL 808"() -> (w912:dbl)
                                "WL 808 Ref" <- w912
                                n505 = Divide(x=w913, y=w912) -> (x/y=w914:dbl)
                                n506 = Number To Fractional String(number=w914, precision (6)=i16 3) -> (F-format string=w911:string)  [unwired: 2 in]
                                }
                                }
                                n507 = local write "WL 808 Absolute/Reference"(w905) -> ()
                              }
                              frame 2 {
                                n508 = flat-sequence {
                                tunnel: [w919] -> w918
                                tunnel: w918 -> [w923]
                                tunnel: w917 -> [w928]
                                tunnel: [w927] -> w916
                                frame #0 {
                                n509 = local read "WL 1550 Ref"() -> (w919:dbl)
                                n510 = Wait (ms)(milliseconds to wait=u32 1) -> ()  [unwired: 1 out]
                                }
                                frame #1 {
                                n511 = local read "WL 1550"() -> (w922:dbl)
                                "WL 1550 Ref" <- w922
                                n512 = Divide(x=w923, y=w922) -> (x/y=w924:dbl)
                                n513 = Number To Fractional String(number=w924, precision (6)=i16 3) -> (F-format string=w921:string)  [unwired: 2 in]
                                n514 = local write "WL 1550 Absolute/Reference"(w921) -> ()
                                }
                                frame #2 {
                                w926 = "\t"
                                w929 = "\t"
                                n515 = local read "WL 455 Absolute/Reference"() -> (w932:string)
                                n516 = local read "WL 808 Absolute/Reference"() -> (w931:string)
                                n517 = local read "WL 1550 Absolute/Reference"() -> (w930:string)
                                n518 = Concatenate Strings(w928, w932, w929, w931, w929, w930, w926, w926) -> (w927:string)
                                }
                                }
                              }
                            }
                            n519 = Concatenate Strings(w893, w892, w886) -> (w887:string)
                            n520 = Format Into String(initial string=w891, w887) -> ()  [unwired: 2 in, 2 out]
                            n521 = Format Into String(initial string=w890, w887) -> ()  [unwired: 2 in, 2 out]
                            n522 = Format Into String(initial string=w889, w887) -> ()  [unwired: 2 in, 2 out]
                            n523 = Format Into String(initial string=w888, w887) -> ()  [unwired: 2 in, 2 out]
                            n524 = Format Into String(initial string=w883, w881, w882, w884, w879) -> ()  [unwired: 2 in, 2 out]
                          }
                        }
                      }
                    }
                  }
                  frame #2 {
                    n525 = local write "Save Glass Log Done"(TRUE ("Save Glass Log Done")) -> ()
                  }
                }
              }
            }
            n526 = local read "System Stop"() -> (w722:bool)
          }
        }
        frame #1 {
          n527 = local read "Glass Full Log Output File"() -> (w938:refnum<file>)
          n528 = local read "Glass 1 Output File"() -> (w942:refnum<file>)
          n529 = local read "Glass 2 Output File"() -> (w941:refnum<file>)
          n530 = local read "Glass 3 Output File"() -> (w940:refnum<file>)
          n531 = local read "Glass 4 Output File"() -> (w939:refnum<file>)
          n532 = local read "Single Meas Output File"() -> (w937:refnum<file>)
          n533 = Close File(refnum=w938) -> ()  [unwired: 1 in, 2 out]
          n534 = Close File(refnum=w942) -> ()  [unwired: 1 in, 2 out]
          n535 = Close File(refnum=w941) -> ()  [unwired: 1 in, 2 out]
          n536 = Close File(refnum=w940) -> ()  [unwired: 1 in, 2 out]
          n537 = Close File(refnum=w939) -> ()  [unwired: 1 in, 2 out]
          n538 = Close File(refnum=w937) -> ()  [unwired: 1 in, 2 out]
        }
      }
      n539 = while {
        stop <- w944 stop-if-true
        n540 = Wait (ms)(milliseconds to wait=u32 1) -> ()  [unwired: 1 out]
        n541 = case shown="True" "Glass Meas Cycle" {
          frame False {
          }
          frame True {
            n542 = while {
              stop <- w949 stop-if-true
              n543 = stacked-sequence {
                tunnel: [_ _ _ w1012] -> w947
                frame #0 {
                  n544 = flat-sequence {
                    tunnel: [w958] -> w953
                    tunnel: [w957] -> w950
                    tunnel: [w961] -> w954
                    tunnel: w953 -> [w961]
                    tunnel: [w960] -> w951
                    tunnel: w950 -> [w960]
                    tunnel: [w965] -> w955
                    tunnel: w954 -> [w965]
                    tunnel: [w964] -> w952
                    tunnel: w951 -> [w964]
                    tunnel: w955 -> [w969]
                    tunnel: w952 -> [w968]
                    frame #0 {
                      n545 = local read "P2 CH1 Used"() -> (w958:bool)
                      n546 = local read "P2 CH1"() -> (w957:bool)
                      "Glass Meas Cycle Running" <- TRUE ("Cycle Running")
                    }
                    frame #1 {
                      n547 = local write "Meas Progress Bar"(u8 0 ("Measuering Progress Bar")) -> ()
                      n548 = property on="Glass Meas" class="Bool (strict)"("DisabledEnum"=T7."Disabled and Grayed Out" ("Disabled")) -> ()  [unwired: 2 in, 2 out]
                      n549 = property on="Погнали!" class="Bool (strict)"("DisabledEnum"=T7."Disabled and Grayed Out" ("Disabled")) -> ()  [unwired: 2 in, 2 out]
                    }
                    frame #2 {
                      n550 = local write "P2 CH1 Used"(TRUE ("P1 CH0 Used")) -> ()
                      n551 = local write "P2 CH1"(TRUE ("P1 CH0")) -> ()
                    }
                    frame #3 {
                      n552 = Not(x=w969) -> (.not. x?=w971:bool)
                      n553 = Not(x=w968) -> (.not. x?=w970:bool)
                      n554 = Or(x=w971, y=w970) -> (x .or. y?=w972:bool)
                      n555 = case shown="True" w972 {
                        frame False {
                        }
                        frame True {
                          n556 = Wait (ms)(milliseconds to wait=u32 100) -> ()  [unwired: 1 out]
                        }
                      }
                    }
                  }
                }
                frame #1 {
                  n557 = for {
                    N: 5 -> [_]
                    i -> [w975]
                    n558 = flat-sequence {
                      tunnel: w975 -> [w976]
                      tunnel: w975 -> [w985]
                      tunnel: w975 -> [w999]
                      frame #0 {
                        n559 = local write "Куда едем?"(w976) -> ()
                      }
                      frame #1 {
                        n560 = local write "Погнали!"(TRUE ("Погнали!")) -> ()
                        n561 = Wait (ms)(milliseconds to wait=u32 200) -> ()  [unwired: 1 out]
                      }
                      frame #2 {
                        n562 = while {
                          stop <- w980 stop-if-true
                          n563 = local read "System Stop"() -> (w981:bool)
                          n564 = local read "Готово"() -> (w982:bool)
                          n565 = Wait (ms)(milliseconds to wait=u32 1) -> ()  [unwired: 1 out]
                          n566 = Compound Arithmetic op=OR(w982, w981) -> (w980:bool)
                        }
                      }
                      frame #3 {
                        n567 = local write "Погнали!"(FALSE ("Погнали!")) -> ()
                        n568 = Wait (ms)(milliseconds to wait=u32 200) -> ()  [unwired: 1 out]
                      }
                      frame #4 {
                        n569 = case shown="1" w985 {
                          frame 0, Default {
                          }
                          frame 1 {
                            n570 = local read "Glass 1 Output File"() -> (→"Glass Num Output File":refnum<file>)
                          }
                          frame 2 {
                            n571 = local read "Glass 2 Output File"() -> (w987:refnum<file>)
                            n572 = local write "Glass Num Output File"(w987) -> ()
                          }
                          frame 3 {
                            n573 = local read "Glass 3 Output File"() -> (w988:refnum<file>)
                            n574 = local write "Glass Num Output File"(w988) -> ()
                          }
                          frame 4 {
                            n575 = local read "Glass 4 Output File"() -> (w989:refnum<file>)
                            n576 = local write "Glass Num Output File"(w989) -> ()
                          }
                        }
                      }
                      frame #5 {
                        n577 = local write "Glass Meas"(TRUE ("Glass Measure")) -> ()
                        n578 = Wait (ms)(milliseconds to wait=u32 50) -> ()  [unwired: 1 out]
                      }
                      frame #6 {
                        n579 = while {
                          stop <- w995 stop-if-true
                          n580 = local read "Meas Running"() -> (w992:bool)
                          n581 = local read "System Stop"() -> (w996:bool)
                          n582 = Wait (ms)(milliseconds to wait=u32 1) -> ()  [unwired: 1 out]
                          n583 = Not(x=w992) -> (.not. x?=w993:bool)
                          n584 = Compound Arithmetic op=OR(w993, w996) -> (w995:bool)
                        }
                      }
                      frame #7 {
                        n585 = local write "Glass Meas"(FALSE ("Glass Measure")) -> ()
                      }
                      frame #8 {
                        n586 = Increment(x=w999) -> (x+1=w1000:i32)
                        n587 = Multiply(x=w1000, y=18) -> (x*y=w1001:i32)
                        n588 = To Unsigned Byte Integer(number=w1001) -> (unsigned 8bit integer=w1002:u8)
                        n589 = local write "Meas Progress Bar"(w1002) -> ()
                        n590 = Wait (ms)(milliseconds to wait=u32 100) -> ()  [unwired: 1 out]
                      }
                    }
                  }
                }
                frame #2 {
                  n591 = flat-sequence {
                    frame #0 {
                      n592 = local write "Куда едем?"(T1."Калибровка" ("Куда едем?")) -> ()
                    }
                    frame #1 {
                      n593 = local write "Погнали!"(TRUE ("Погнали!")) -> ()
                    }
                    frame #2 {
                      n594 = Wait (ms)(milliseconds to wait=u32 100) -> ()  [unwired: 1 out]
                    }
                    frame #3 {
                      n595 = local write "Погнали!"(FALSE ("Погнали!")) -> ()
                    }
                    frame #4 {
                      n596 = while {
                        stop <- w1008 stop-if-true
                        n597 = local read "System Stop"() -> (w1009:bool)
                        n598 = local read "Готово"() -> (w1010:bool)
                        n599 = Compound Arithmetic op=OR(w1010, w1009) -> (w1008:bool)
                      }
                    }
                    frame #5 {
                      n600 = Wait (ms)(milliseconds to wait=u32 200) -> ()  [unwired: 1 out]
                    }
                  }
                }
                frame #3 {
                  n601 = flat-sequence {
                    tunnel: [w1024] -> w1012
                    frame #0 {
                      n602 = local read "Glass Meas Cycle"() -> (w1013:bool)
                      n603 = case shown="False" w1013 {
                        frame False {
                          n604 = local write "P2 CH1 Used"(FALSE ("P1 CH0 Used")) -> ()
                        }
                        frame True {
                        }
                      }
                    }
                    frame #1 {
                      n605 = local read "Num of Meas"() -> (w1016:u32)
                      n606 = local read "Meas Progress Bar"() -> (w1020:u8)
                      n607 = Increment(x=w1016) -> (x+1=→"Num of Meas":u32)
                      n608 = Add(x=w1020, y=u8 10) -> (x+y=w1019:u8)
                      n609 = local write "Meas Progress Bar"(w1019) -> ()
                      n610 = Wait (ms)(milliseconds to wait=u32 100) -> ()  [unwired: 1 out]
                    }
                    frame #2 {
                      n611 = local write "Glass Meas Cycle Running"(FALSE ("Glass Meas Cycle Running")) -> ()
                      n612 = property on="Glass Meas" class="Bool (strict)"("DisabledEnum"=T7."Enabled" ("Disabled")) -> ()  [unwired: 2 in, 2 out]
                      n613 = property on="Погнали!" class="Bool (strict)"("DisabledEnum"=T7."Enabled" ("Disabled")) -> ()  [unwired: 2 in, 2 out]
                    }
                    frame #3 {
                      n614 = local read "Glass Meas Cycle"() -> (w1025:bool)
                      n615 = Not(x=w1025) -> (.not. x?=w1024:bool)
                    }
                  }
                }
              }
              n616 = Wait (ms)(milliseconds to wait=u32 1) -> ()  [unwired: 1 out]
              n617 = local read "System Stop"() -> (w948:bool)
              n618 = Or(x=w947, y=w948) -> (x .or. y?=w949:bool)
            }
          }
        }
        n619 = local read "System Stop"() -> (w944:bool)
      }
      n620 = while {
        shift-right: ["Glass Meas"] -> _
        shift-left: FALSE ("Glass Measure") -> [w1027]
        stop <- w1030 stop-if-true
        n621 = Wait (ms)(milliseconds to wait=u32 1) -> ()  [unwired: 1 out]
        n622 = Greater?(x="Glass Meas", y=w1027) -> (0:w1028:bool)
        n623 = case shown="True" w1028 {
          frame False {
          }
          frame True {
            n624 = stacked-sequence {
              frame #0 {
                n625 = flat-sequence {
                  frame #0 {
                    w1031 = T7."Disabled and Grayed Out" ("Disabled")
                    n626 = property on="P1 CH0 Used" class="Bool (strict)"("DisabledEnum"=w1031) -> ()  [unwired: 2 in, 2 out]
                    n627 = property on="P1 CH1 Used" class="Bool (strict)"("DisabledEnum"=w1031) -> ()  [unwired: 2 in, 2 out]
                    n628 = property on="P1 CH2 Used" class="Bool (strict)"("DisabledEnum"=w1031) -> ()  [unwired: 2 in, 2 out]
                    n629 = property on="P2 CH0 Used" class="Bool (strict)"("DisabledEnum"=w1031) -> ()  [unwired: 2 in, 2 out]
                    n630 = property on="P2 CH1 Used" class="Bool (strict)"("DisabledEnum"=w1031) -> ()  [unwired: 2 in, 2 out]
                    n631 = property on="P2 CH2 Used" class="Bool (strict)"("DisabledEnum"=w1031) -> ()  [unwired: 2 in, 2 out]
                    "Meas Running" <- TRUE ("Done")
                  }
                  frame #1 {
                    n632 = local write "P1 CH2 Used"(TRUE ("P1 CH0 Used")) -> ()
                    n633 = local write "P1 CH2"(TRUE ("P1 CH2")) -> ()
                    n634 = Wait (ms)(milliseconds to wait=u32 100) -> ()  [unwired: 1 out]
                  }
                }
              }
              frame #1 {
                n635 = for {
                  N: 3 -> [_]
                  i -> [w1038]
                  n636 = flat-sequence {
                    tunnel: w1038 -> [w1043]
                    tunnel: w1038 -> [w1047]
                    tunnel: w1038 -> [w1056]
                    tunnel: [w1054] -> w1037
                    tunnel: [w1074] -> w1041
                    tunnel: [w1073] -> w1040
                    tunnel: [w1072] -> w1039
                    tunnel: w1038 -> [w1070]
                    tunnel: w1037 -> [w1069]
                    tunnel: w1041 -> [w1109]
                    tunnel: w1040 -> [w1107]
                    tunnel: w1039 -> [w1098]
                    tunnel: w1038 -> [w1096]
                    tunnel: w1038 -> [w1115]
                    frame #0 {
                      n637 = case shown="0, Default" w1043 {
                        frame 0, Default {
                          n638 = local write "P1 CH0 Used"(TRUE ("P1 CH0 Used")) -> ()
                        }
                        frame 1 {
                          n639 = local write "P1 CH1 Used"(TRUE ("P1 CH0 Used")) -> ()
                        }
                        frame 2 {
                          n640 = local write "P2 CH0 Used"(TRUE ("P1 CH0 Used")) -> ()
                        }
                      }
                      n641 = Wait (ms)(milliseconds to wait=u32 100) -> ()  [unwired: 1 out]
                    }
                    frame #1 {
                      n642 = case shown="2" w1047 {
                        frame 0, Default {
                          n643 = local write "P1 CH0"(TRUE ("P1 CH0")) -> ()
                          n644 = Wait (ms)(milliseconds to wait=u32 2000) -> ()  [unwired: 1 out]
                        }
                        frame 1 {
                          n645 = local write "P1 CH1"(TRUE ("P1 CH0")) -> ()
                          n646 = Wait (ms)(milliseconds to wait=u32 2000) -> ()  [unwired: 1 out]
                        }
                        frame 2 {
                          n647 = local write "P2 CH0"(TRUE ("P1 CH0")) -> ()
                          n648 = Wait (ms)(milliseconds to wait=u32 12000) -> ()  [unwired: 1 out]
                        }
                      }
                    }
                    frame #2 {
                      w1062 = "\t"
                      w1057 = i16 12 ("precision (6)")
                      n649 = case shown="0, Default" w1056 {
                        tunnel: [w1064 w1066 w1068] -> w1061
                        tunnel: [w1063 w1065 w1067] -> w1059
                        frame 0, Default {
                          n650 = local read "P1 CH0, V"() -> (w1064:dbl)
                          n651 = local read "P1 CH0_cur, A"() -> (w1063:dbl)
                        }
                        frame 1 {
                          n652 = local read "P1 CH1_cur, A"() -> (w1065:dbl)
                          n653 = local read "P1 CH1, V"() -> (w1066:dbl)
                        }
                        frame 2 {
                          n654 = local read "P2 CH0_cur, A"() -> (w1067:dbl)
                          n655 = local read "P2 CH0, V"() -> (w1068:dbl)
                        }
                      }
                      n656 = local read "Glass Meas Cycle Running"() -> (w1054:bool)
                      n657 = Number To Fractional String(number=w1061, precision (6)=w1057) -> (F-format string=w1060:string)  [unwired: 2 in]
                      n658 = Number To Fractional String(number=w1059, precision (6)=w1057) -> (F-format string=w1058:string)  [unwired: 2 in]
                      n659 = Concatenate Strings(w1060, w1062, w1058, w1062) -> (→"CH Data String":string)
                    }
                    frame #3 {
                      w1073 = 5
                      n660 = for {
                        N: w1073 -> [_]
                        shift-right: [w1090] -> w1072
                        shift-left: "" -> [w1089]
                        shift-right: [w1086] -> w1074
                        shift-left: 0.0 -> [w1084]
                        tunnel: w1070 -> [w1083]
                        n661 = case shown="0, Default" w1083 {
                          tunnel: [w1092 w1093 w1094] -> w1085
                          frame 0, Default {
                            n662 = local read "DMM 1 Real Current"() -> (w1092:dbl)
                          }
                          frame 1 {
                            n663 = local read "DMM 2 Real Current"() -> (w1093:dbl)
                          }
                          frame 2 {
                            n664 = local read "DMM 3 Real Current"() -> (w1094:dbl)
                          }
                        }
                        n665 = Wait (ms)(milliseconds to wait="Meas Wait") -> ()  [unwired: 1 out]
                        n666 = Add(x=w1084, y=w1085) -> (x+y=w1086:dbl)
                        n667 = Number To Fractional String(number=w1085, precision (6)=i16 12) -> (F-format string=w1088:string)  [unwired: 2 in]
                        n668 = Concatenate Strings(w1089, w1088, "\t") -> (w1090:string)
                      }
                      n669 = case shown="False" w1069 {
                        tunnel: w1070 -> [w1076 _]
                        frame False {
                          n670 = local read "Set Last Meas As Ref"() -> (w1077:bool)
                          n671 = case shown="False" w1077 {
                            tunnel: w1076 -> [w1078 _]
                            frame False {
                              n672 = case shown="0, Default" w1078 {
                                frame 0, Default {
                                n673 = local read "WL 455"() -> (w1079:dbl)
                                n674 = local write "WL 455 Ref"(w1079) -> ()
                                }
                                frame 1 {
                                n675 = local read "WL 808"() -> (w1080:dbl)
                                n676 = local write "WL 808 Ref"(w1080) -> ()
                                }
                                frame 2 {
                                n677 = local read "WL 1550"() -> (w1081:dbl)
                                n678 = local write "WL 1550 Ref"(w1081) -> ()
                                }
                              }
                            }
                            frame True {
                            }
                          }
                        }
                        frame True {
                        }
                      }
                    }
                    frame #4 {
                      n679 = local read "Glass Meas Cycle Running"() -> (w1097:bool)
                      n680 = To Double Precision Float(number=w1107) -> (double precision float=w1108:dbl)
                      n681 = Divide(x=w1109, y=w1108) -> (x/y=w1106:dbl)
                      n682 = Wait (ms)(milliseconds to wait=u32 1) -> ()  [unwired: 1 out]
                      n683 = Number To Fractional String(number=w1106, precision (6)=i16 12) -> (F-format string=w1101:string)  [unwired: 2 in]
                      n684 = case shown="2" w1096 {
                        tunnel: w1106 -> [w1111 w1112 w1113]
                        frame 0, Default {
                          "WL 455" <- w1111
                        }
                        frame 1 {
                          "WL 808" <- w1112
                        }
                        frame 2 {
                          "WL 1550" <- w1113
                        }
                      }
                      n685 = case shown="True" w1097 {
                        frame False {
                        }
                        frame True {
                          n686 = local read "Glass Num Output File"() -> (→"Glass Meas Path":refnum<file>)
                        }
                      }
                      n687 = Concatenate Strings(w1101, "\t") -> (→"Av Cur Data String":string)
                      n688 = Format Date/Time String(time format string (%c)="%H:%M:%S:%3u") -> (date/time string=w1104:string)  [unwired: 2 in]
                      n689 = Concatenate Strings(w1104, "\t") -> (→"Meas Time String":string)
                      "All Cur Data String" <- w1098
                    }
                    frame #5 {
                      n690 = case shown="0, Default" w1115 {
                        frame 0, Default {
                          n691 = local write "P1 CH0 Used"(FALSE ("P1 CH0 Used")) -> ()
                        }
                        frame 1 {
                          n692 = local write "P1 CH1 Used"(FALSE ("P1 CH0 Used")) -> ()
                        }
                        frame 2 {
                          n693 = local write "P2 CH0 Used"(FALSE ("P1 CH0 Used")) -> ()
                        }
                      }
                      n694 = Wait (ms)(milliseconds to wait=u32 500) -> ()  [unwired: 1 out]
                    }
                    frame #6 {
                      n695 = local write "Save Glass Log Data"(TRUE ("Save Glass Log Data")) -> ()
                      n696 = Wait (ms)(milliseconds to wait=u32 50) -> ()  [unwired: 1 out]
                    }
                    frame #7 {
                      n697 = while {
                        stop <- w1123 stop-if-true
                        n698 = local read "System Stop"() -> (w1124:bool)
                        n699 = local read "Save Glass Log Done"() -> (w1125:bool)
                        n700 = Wait (ms)(milliseconds to wait=u32 1) -> ()  [unwired: 1 out]
                        n701 = Compound Arithmetic op=OR(w1125, w1124) -> (w1123:bool)
                      }
                    }
                    frame #8 {
                      n702 = local write "Save Glass Log Data"(FALSE ("Save Glass Log Data")) -> ()
                    }
                  }
                  "WL-i" <- w1038
                }
              }
              frame #2 {
                n703 = flat-sequence {
                  frame #0 {
                    n704 = local write "P1 CH2 Used"(FALSE ("P1 CH0 Used")) -> ()
                    n705 = Wait (ms)(milliseconds to wait=u32 100) -> ()  [unwired: 1 out]
                  }
                  frame #1 {
                    w1129 = T7."Enabled" ("Disabled")
                    n706 = local write "Meas Running"(FALSE ("Done")) -> ()
                    n707 = property on="P1 CH0 Used" class="Bool (strict)"("DisabledEnum"=w1129) -> ()  [unwired: 2 in, 2 out]
                    n708 = property on="P1 CH1 Used" class="Bool (strict)"("DisabledEnum"=w1129) -> ()  [unwired: 2 in, 2 out]
                    n709 = property on="P1 CH2 Used" class="Bool (strict)"("DisabledEnum"=w1129) -> ()  [unwired: 2 in, 2 out]
                    n710 = property on="P2 CH0 Used" class="Bool (strict)"("DisabledEnum"=w1129) -> ()  [unwired: 2 in, 2 out]
                    n711 = property on="P2 CH1 Used" class="Bool (strict)"("DisabledEnum"=w1129) -> ()  [unwired: 2 in, 2 out]
                    n712 = property on="P2 CH2 Used" class="Bool (strict)"("DisabledEnum"=w1129) -> ()  [unwired: 2 in, 2 out]
                  }
                }
              }
            }
          }
        }
        n713 = local read "System Stop"() -> (w1030:bool)
      }
      n714 = while {
        tunnel: w693 -> [w1177]
        shift-right: [w1167] -> _
        shift-left: FALSE ("Погнали!") -> [w1178]
        tunnel: [w1176] -> w694
        shift-right: [w1174] -> _
        shift-left: w692 -> [w1175]
        tunnel: w691 -> [w1173]
        stop <- w1170 stop-if-true
        n715 = Wait (ms)(milliseconds to wait=u32 1) -> ()  [unwired: 1 out]
        n716 = case shown="True" "Погнали!" {
          selector: "Погнали!" -> [w1179 _]
          tunnel: [w1179 w1180] -> w1167
          frame False {
          }
          frame True {
            n717 = local read "P2 CH1"() -> (w1181:bool)
            n718 = case shown="True" w1181 {
              selector: w1181 -> [_ w1185]
              tunnel: [w1182 w1185] -> w1180
              frame False {
                n719 = One Button Dialog(message="Power up the stepper motor.") -> (true=w1183:bool)  [unwired: 1 in]
                n720 = Not(x=w1183) -> (.not. x?=w1182:bool)
                n721 = local write "Погнали!"(w1182) -> ()
              }
              frame True {
              }
            }
          }
        }
        n722 = local read "System Stop"() -> (w1170:bool)
        n723 = case shown="\"Первое стекло\"" "Куда едем?" {
          tunnel: [0.0 -1550.0 -2700.0 -4100.0 -5250.0] -> w1171
          frame "Калибровка", Default {
          }
          frame "Первое стекло" {
          }
          frame "Второе стекло" {
          }
          frame "Третье стекло" {
          }
          frame "Четвертое стекло" {
          }
        }
        n724 = Greater?(x=w1167, y=w1178) -> (0:w1166:bool)
        n725 = case shown="True" w1166 {
          tunnel: w1171 -> [_ w1198]
          tunnel: w1177 -> [w1192 w1197]
          tunnel: [w1192 w1196] -> w1176
          tunnel: w1175 -> [w1191 _]
          tunnel: [w1191 w1195] -> w1174
          tunnel: w1173 -> [_ w1194]
          frame False {
            n726 = Wait (ms)(milliseconds to wait=u32 1) -> ()  [unwired: 1 out]
            "Текущая позиция" <- w1191
          }
          frame True {
            n727 = while {
              tunnel: w1198 -> [w1203]
              tunnel: w1197 -> [w1206]
              tunnel: [w1200] -> w1196
              tunnel: [w1205] -> w1195
              tunnel: w1194 -> [w1202]
              stop <- w1204 stop-if-true
              n728 = invoke class="AmateurStepperMotorWcfClient" method="GoTo"(reference=w1206, "destinationPosition"=w1203) -> (reference out=w1208:refnum<k24>, "GoTo"=w1209:refnum<k24>)  [unwired: 2 in, 2 out]
              n729 = invoke class="Task" method="ConfigureAwait"(reference=w1209, "continueOnCapturedContext"=FALSE) -> ()  [unwired: 2 in, 4 out]
              n730 = Wait (ms)(milliseconds to wait=u32 1) -> ()  [unwired: 1 out]
              n731 = while {
                tunnel: [w1212] -> w1205
                tunnel: w1208 -> [w1220]
                tunnel: [w1219] -> w1201
                tunnel: [w1211] -> w1204
                tunnel: w1203 -> [w1217]
                tunnel: w1202 -> [w1215]
                stop <- w1211 stop-if-true
                n732 = property class="AmateurStepperMotorWcfClient"(reference=w1220) -> (reference out=w1219:refnum<k24>, "Position"=w1212:dbl)  [unwired: 1 in, 1 out]
                n733 = Subtract(x=w1212, y=w1217) -> (x-y=w1218:dbl)
                n734 = Wait (ms)(milliseconds to wait=u32 1) -> ()  [unwired: 1 out]
                n735 = Absolute Value(x=w1218) -> (abs(x)=w1216:dbl)
                n736 = Less Or Equal?(x=w1216, y=w1215) -> (x <= y?=w1214:bool)
                n737 = local write "Текущая позиция"(w1212) -> ()
                n738 = Or(x=w1214, y="Стоп GoTo") -> (x .or. y?=w1211:bool)
                "Готово" <- w1211
              }
              n739 = invoke class="AmateurStepperMotorWcfClient" method="Stop"(reference=w1201) -> (reference out=w1200:refnum<k24>)  [unwired: 2 in, 2 out]
            }
          }
        }
      }
      n740 = while {
        stop <- w700 stop-if-true
        n741 = Wait (ms)(milliseconds to wait=u32 1) -> ()  [unwired: 1 out]
        n742 = case shown="True" "Clear Table" {
          frame False {
          }
          frame True {
            n743 = for {
              N: 4 -> [_]
              i -> [w703]
              n744 = for {
                N: 3 -> [_]
                tunnel: w703 -> [w705]
                i -> [w708]
                n745 = Increment(x=w705) -> (x+1=w706:i32)
                n746 = local read "Glass Table"() -> (w710:string[][])
                n747 = Increment(x=w708) -> (x+1=w707:i32)
                n748 = Replace Array Subset(array=w710, new element="" ("new element/subarray"), index (row)=w706, index (col)=w707) -> (w709:string[][])
                n749 = local write "Glass Table"(w709) -> ()
              }
            }
          }
        }
        n750 = local read "System Stop"() -> (w700:bool)
      }
      n751 = while {
        shift-right: [w1131] -> _
        shift-left: 0 ("t") -> [w1132]
        stop <- w1135 stop-if-true
        n752 = Wait (ms)(milliseconds to wait=u32 5) -> ()  [unwired: 1 out]
        n753 = case shown="True" "Тест" {
          tunnel: w1132 -> [w1138 w1145]
          tunnel: [w1138 w1142] -> w1131
          frame False {
          }
          frame True {
            n754 = flat-sequence {
              tunnel: w1145 -> [w1147]
              tunnel: [w1146] -> w1140
              tunnel: [w1152] -> w1141
              tunnel: w1140 -> [w1152]
              tunnel: [w1154] -> w1143
              tunnel: w1141 -> [w1154]
              tunnel: [w1155] -> w1144
              tunnel: w1143 -> [w1155]
              tunnel: w1144 -> [w1160]
              tunnel: [w1158] -> w1139
              tunnel: [w1165] -> w1142
              tunnel: w1139 -> [w1165]
              frame #0 {
                n755 = while {
                  tunnel: w1147 -> [w1150]
                  tunnel: [w1150] -> w1146
                  stop <- w1149 stop-if-true
                  n756 = local read "Готово"() -> (w1149:bool)
                  n757 = Wait (ms)(milliseconds to wait=u32 1) -> ()  [unwired: 1 out]
                }
              }
              frame #1 {
                n758 = local write "Куда едем?"(w1152) -> ()
                n759 = Wait (ms)(milliseconds to wait=u32 500) -> ()  [unwired: 1 out]
              }
              frame #2 {
                n760 = local write "Погнали!"(TRUE ("Погнали!")) -> ()
              }
              frame #3 {
                n761 = Wait (ms)(milliseconds to wait=u32 50) -> ()  [unwired: 1 out]
              }
              frame #4 {
                n762 = local write "Погнали!"(FALSE ("Погнали!")) -> ()
                n763 = Equal?(x=4, y=w1160) -> (x = y?=w1162:bool)
                n764 = Increment(x=w1160) -> (x+1=w1159:i32)
                n765 = Select(t=0, s=w1162, f=w1159) -> (s? t:f=w1158:i32)
              }
              frame #5 {
                n766 = Wait (ms)(milliseconds to wait=u32 50) -> ()  [unwired: 1 out]
              }
            }
          }
        }
        n767 = local read "System Stop"() -> (w1134:bool)
        n768 = Or(x=w1134, y="Стоп_тест") -> (x .or. y?=w1135:bool)
      }
      n769 = invoke class="AmateurStepperMotorWcfClient" method="Stop"(reference=w694) -> (reference out=w697:refnum<k24>, "Stop"=w698:refnum<k24>)  [unwired: 2 in, 1 out]
      n770 = invoke class="Task" method="Wait"(reference=w698) -> ()  [unwired: 2 in, 3 out]
      n771 = property class="AmateurStepperMotorWcfClient"(reference=w697, "HoldOn"=FALSE) -> (reference out=w696:refnum<k24>)  [unwired: 1 in, 1 out]
      n772 = invoke class="AmateurStepperMotorWcfClient" method="Dispose"(reference=w696) -> ()  [unwired: 2 in, 3 out]
    }
  }
  n773 = case shown="True" w26 {
    tunnel: w32 -> [_ w1227]
    tunnel: w10 -> [_ _]
    tunnel: w29 -> [_ w1224]
    frame False {
    }
    frame True {
      n774 = local read "NI DMM 1 Option Return"() -> (w1221:enum32{"Ampermeter button", "Ohmmeter button"})
      n775 = case shown="\"Ohmmeter button\"" w1221 {
        tunnel: w1227 -> [w1232 w1278]
        tunnel: [w1231 w1277] -> w1226
        tunnel: [w1230 w1276] -> w1225
        tunnel: w1224 -> [w1229 w1279]
        tunnel: [w1228 w1275] -> w1223
        frame "Ampermeter button", Default {
          n776 = while {
            tunnel: w1232 -> [w1244]
            tunnel: [w1242] -> w1231
            tunnel: [w1241] -> w1230
            tunnel: w1229 -> [w1239]
            tunnel: [w1235] -> w1228
            stop <- w1240 stop-if-true
            n777 = flat-sequence {
              tunnel: [w1250] -> w1245
              tunnel: w1244 -> [w1248]
              tunnel: w1239 -> [w1252]
              tunnel: [w1249] -> w1238
              tunnel: w1245 -> [w1255]
              tunnel: [w1260] -> w1243
              tunnel: w1238 -> [w1259]
              tunnel: [w1258] -> w1237
              tunnel: [w1254] -> w1233
              tunnel: w1243 -> [w1265]
              tunnel: [w1266] -> w1242
              tunnel: [w1265] -> w1241
              tunnel: [w1264] -> w1240
              tunnel: w1237 -> [w1263]
              tunnel: [w1263] -> w1236
              tunnel: w1233 -> [w1262]
              frame #0 {
                w1246 = T9 6.5 items=["3 1/2"=3.5, "4 1/2"=4.5, "5 1/2"=5.5, "6 1/2"=6.5, "7 1/2"=7.5] ("Resolution in Digits")
                n778 = Fract/Exp String To Number(string="NI DMM 1 Current Range") -> (number=w1251:dbl)  [unwired: 3 in, 1 out]
                n779 = call-poly <instrlib>:"niDMM Config Measurement.vi"("Range"=w1251, "Resolution in Digits"=w1246, "error in (no error)"=w1252, "Function"=niDMM_Function."DC Current" ("Measurement Type"), "instrument handle"=w1248) -> ("error out"=w1249:errorcluster, "instrument handle out"=w1250:refnum<k15>)  [unwired: 5 in]
              }
              frame #1 {
                n780 = call <instrlib>:"niDMM Read.vi"("error in (no error)"=w1259, "instrument handle"=w1255) -> ("error out"=w1258:errorcluster, "Measurement"=w1254:dbl, "instrument handle out"=w1260:refnum<k15>)  [unwired: 7 in]
                "DMM 1 Real Current" <- w1254
                n781 = Fract/Exp String To Number(string="NI DMM 1 units") -> (number=w1256:dbl)  [unwired: 3 in, 1 out]
                n782 = Multiply(x=w1256, y=w1254) -> (x*y=→"NI DMM 1 Current" →"NI DMM 1 Current Char":dbl)
              }
              frame #2 {
                w1274 = 15
                n783 = local read "NI DMM 1 Current output file"() -> (w1267:refnum<file>)
                n784 = Format Date/Time String(time format string (%c)="%H:%M:%S:%3u") -> (date/time string=w1272:string)  [unwired: 2 in]
                n785 = Number To Fractional String(number=w1262, width (-)=w1274, precision (6)=w1274) -> (F-format string=w1269:string)  [unwired: 1 in]
                n786 = local read "System Stop"() -> (w1264:bool)
                n787 = Concatenate Strings(w1272, "\t", w1269, "\r\n") -> (w1270:string)
                n788 = Format Into String(initial string=w1267, w1270) -> (resulting string=w1266:refnum<file>)  [unwired: 2 in, 1 out]
              }
            }
            n789 = Wait (ms)(milliseconds to wait="NI DMM 1 Current Wait") -> ()  [unwired: 1 out]
            n790 = call <vilib>:"Simple Error Handler.vi"("error in (no error)"=w1236) -> ("error out"=w1235:errorcluster)  [unwired: 1 in, 7 out]
          }
        }
        frame "Ohmmeter button" {
          n791 = while {
            tunnel: w1278 -> [w1291]
            tunnel: [w1289] -> w1277
            tunnel: [w1288] -> w1276
            tunnel: w1279 -> [w1286]
            tunnel: [w1282] -> w1275
            stop <- w1287 stop-if-true
            n792 = flat-sequence {
              tunnel: [w1298] -> w1292
              tunnel: w1291 -> [w1297]
              tunnel: w1286 -> [w1296]
              tunnel: [w1295] -> w1285
              tunnel: w1292 -> [w1308]
              tunnel: [w1306] -> w1290
              tunnel: w1285 -> [w1305]
              tunnel: [w1304] -> w1284
              tunnel: [w1301] -> w1280
              tunnel: w1290 -> [w1313]
              tunnel: [w1314] -> w1289
              tunnel: [w1313] -> w1288
              tunnel: [w1312] -> w1287
              tunnel: [w1311] -> w1283
              tunnel: w1284 -> [w1311]
              tunnel: w1280 -> [w1310]
              frame #0 {
                w1300 = T9 6.5 items=["3 1/2"=3.5, "4 1/2"=4.5, "5 1/2"=5.5, "6 1/2"=6.5, "7 1/2"=7.5] ("Resolution in Digits")
                n793 = Fract/Exp String To Number(string="NI DMM 1 Resistance Range") -> (number=w1293:dbl)  [unwired: 3 in, 1 out]
                n794 = call-poly <instrlib>:"niDMM Config Measurement.vi"("Range"=w1293, "Resolution in Digits"=w1300, "error in (no error)"=w1296, "Function"=niDMM_Function."2-wire Resistance" ("Measurement Type"), "instrument handle"=w1297) -> ("error out"=w1295:errorcluster, "instrument handle out"=w1298:refnum<k15>)  [unwired: 5 in]
              }
              frame #1 {
                n795 = call <instrlib>:"niDMM Read.vi"("error in (no error)"=w1305, "instrument handle"=w1308) -> ("error out"=w1304:errorcluster, "Measurement"=w1301:dbl, "instrument handle out"=w1306:refnum<k15>)  [unwired: 7 in]
                n796 = Fract/Exp String To Number(string="NI DMM 1 Resistance units") -> (number=w1302:dbl)  [unwired: 3 in, 1 out]
                n797 = Multiply(x=w1302, y=w1301) -> (x*y=→"NI DMM 1 Resistance" →"NI DMM 1 Resistance Char":dbl)
              }
              frame #2 {
                w1315 = 15
                n798 = local read "NI DMM 1 Resistance output file"() -> (w1321:refnum<file>)
                n799 = Format Date/Time String(time format string (%c)="%H:%M:%S:%3u") -> (date/time string=w1317:string)  [unwired: 2 in]
                n800 = Number To Fractional String(number=w1310, width (-)=w1315, precision (6)=w1315) -> (F-format string=w1309:string)  [unwired: 1 in]
                n801 = Concatenate Strings(w1317, "\t", w1309, "\r\n") -> (w1319:string)
                n802 = local read "System Stop"() -> (w1312:bool)
                n803 = Format Into String(initial string=w1321, w1319) -> (resulting string=w1314:refnum<file>)  [unwired: 2 in, 1 out]
              }
            }
            n804 = Wait (ms)(milliseconds to wait="NI DMM 1 Resistance Wait") -> ()  [unwired: 1 out]
            n805 = call <vilib>:"Simple Error Handler.vi"("error in (no error)"=w1283) -> ("error out"=w1282:errorcluster)  [unwired: 1 in, 7 out]
          }
        }
      }
      n806 = call <instrlib>:"niDMM Close.vi"("error in (no error)"=w1223, "instrument handle"=w1225) -> ("error out"=w1222:errorcluster)  [unwired: 9 in]
      n807 = local write "NI DMM 1 error out"(w1222) -> ()
      n808 = Close File(refnum=w1226) -> ()  [unwired: 1 in, 2 out]
      n809 = call <vilib>:"Simple Error Handler.vi"("error in (no error)"=w1222) -> ()  [unwired: 1 in, 8 out]
    }
  }
  n810 = case shown="True" w25 {
    tunnel: w31 -> [_ w1328]
    tunnel: w10 -> [_ _]
    tunnel: w28 -> [_ w1325]
    frame False {
    }
    frame True {
      n811 = local read "NI DMM 2 Option Return"() -> (w1322:enum32{"Ampermeter button", "Ohmmeter button"})
      n812 = case shown="\"Ohmmeter button\"" w1322 {
        tunnel: w1328 -> [w1333 w1380]
        tunnel: [w1332 w1378] -> w1327
        tunnel: [w1331 w1377] -> w1326
        tunnel: w1325 -> [w1330 w1379]
        tunnel: [w1329 w1376] -> w1324
        frame "Ampermeter button", Default {
          n813 = while {
            tunnel: w1333 -> [w1345]
            tunnel: [w1343] -> w1332
            tunnel: [w1342] -> w1331
            tunnel: w1330 -> [w1340]
            tunnel: [w1336] -> w1329
            stop <- w1341 stop-if-true
            n814 = flat-sequence {
              tunnel: [w1349] -> w1346
              tunnel: w1345 -> [w1347]
              tunnel: w1340 -> [w1353]
              tunnel: [w1348] -> w1339
              tunnel: w1346 -> [w1356]
              tunnel: [w1361] -> w1344
              tunnel: w1339 -> [w1360]
              tunnel: [w1359] -> w1338
              tunnel: [w1355] -> w1334
              tunnel: w1344 -> [w1366]
              tunnel: [w1367] -> w1343
              tunnel: [w1366] -> w1342
              tunnel: [w1365] -> w1341
              tunnel: [w1364] -> w1337
              tunnel: w1338 -> [w1364]
              tunnel: w1334 -> [w1363]
              frame #0 {
                w1350 = T9 6.5 items=["3 1/2"=3.5, "4 1/2"=4.5, "5 1/2"=5.5, "6 1/2"=6.5, "7 1/2"=7.5] ("Resolution in Digits")
                n815 = Fract/Exp String To Number(string="NI DMM 2 Current Range") -> (number=w1352:dbl)  [unwired: 3 in, 1 out]
                n816 = call-poly <instrlib>:"niDMM Config Measurement.vi"("Range"=w1352, "Resolution in Digits"=w1350, "error in (no error)"=w1353, "Function"=niDMM_Function."DC Current" ("Measurement Type"), "instrument handle"=w1347) -> ("error out"=w1348:errorcluster, "instrument handle out"=w1349:refnum<k15>)  [unwired: 5 in]
              }
              frame #1 {
                n817 = call <instrlib>:"niDMM Read.vi"("error in (no error)"=w1360, "instrument handle"=w1356) -> ("error out"=w1359:errorcluster, "Measurement"=w1355:dbl, "instrument handle out"=w1361:refnum<k15>)  [unwired: 7 in]
                "DMM 2 Real Current" <- w1355
                n818 = Fract/Exp String To Number(string="NI DMM 2 units") -> (number=w1357:dbl)  [unwired: 3 in, 1 out]
                n819 = Multiply(x=w1357, y=w1355) -> (x*y=→"NI DMM 2 Current" →"NI DMM 2 Current Char":dbl)
              }
              frame #2 {
                w1368 = 15
                n820 = local read "NI DMM 2 Current output file"() -> (w1375:refnum<file>)
                n821 = Format Date/Time String(time format string (%c)="%H:%M:%S:%3u") -> (date/time string=w1370:string)  [unwired: 2 in]
                n822 = Number To Fractional String(number=w1363, width (-)=w1368, precision (6)=w1368) -> (F-format string=w1373:string)  [unwired: 1 in]
                n823 = local read "System Stop"() -> (w1365:bool)
                n824 = Concatenate Strings(w1370, "\t", w1373, "\r\n") -> (w1372:string)
                n825 = Format Into String(initial string=w1375, w1372) -> (resulting string=w1367:refnum<file>)  [unwired: 2 in, 1 out]
              }
            }
            n826 = Wait (ms)(milliseconds to wait="NI DMM 2 Current Wait") -> ()  [unwired: 1 out]
            n827 = call <vilib>:"Simple Error Handler.vi"("error in (no error)"=w1337) -> ("error out"=w1336:errorcluster)  [unwired: 1 in, 7 out]
          }
        }
        frame "Ohmmeter button" {
          n828 = while {
            tunnel: w1380 -> [w1392]
            tunnel: [w1390] -> w1378
            tunnel: [w1389] -> w1377
            tunnel: w1379 -> [w1387]
            tunnel: [w1383] -> w1376
            stop <- w1388 stop-if-true
            n829 = flat-sequence {
              tunnel: [w1399] -> w1393
              tunnel: w1392 -> [w1398]
              tunnel: w1387 -> [w1397]
              tunnel: [w1396] -> w1386
              tunnel: w1393 -> [w1404]
              tunnel: [w1403] -> w1391
              tunnel: w1386 -> [w1408]
              tunnel: [w1407] -> w1385
              tunnel: [w1402] -> w1381
              tunnel: w1391 -> [w1414]
              tunnel: [w1415] -> w1390
              tunnel: [w1414] -> w1389
              tunnel: [w1413] -> w1388
              tunnel: [w1412] -> w1384
              tunnel: w1385 -> [w1412]
              tunnel: w1381 -> [w1411]
              frame #0 {
                w1401 = T9 6.5 items=["3 1/2"=3.5, "4 1/2"=4.5, "5 1/2"=5.5, "6 1/2"=6.5, "7 1/2"=7.5] ("Resolution in Digits")
                n830 = Fract/Exp String To Number(string="NI DMM 2 Resistance Range") -> (number=w1395:dbl)  [unwired: 3 in, 1 out]
                n831 = call-poly <instrlib>:"niDMM Config Measurement.vi"("Range"=w1395, "Resolution in Digits"=w1401, "error in (no error)"=w1397, "Function"=niDMM_Function."2-wire Resistance" ("Measurement Type"), "instrument handle"=w1398) -> ("error out"=w1396:errorcluster, "instrument handle out"=w1399:refnum<k15>)  [unwired: 5 in]
              }
              frame #1 {
                n832 = call <instrlib>:"niDMM Read.vi"("error in (no error)"=w1408, "instrument handle"=w1404) -> ("error out"=w1407:errorcluster, "Measurement"=w1402:dbl, "instrument handle out"=w1403:refnum<k15>)  [unwired: 7 in]
                n833 = Fract/Exp String To Number(string="NI DMM 2 Resistance units") -> (number=w1405:dbl)  [unwired: 3 in, 1 out]
                n834 = Multiply(x=w1405, y=w1402) -> (x*y=→"NI DMM 2 Resistance" →"NI DMM 2 Resistance Char":dbl)
              }
              frame #2 {
                w1416 = 15
                n835 = local read "NI DMM 2 Resistance output file"() -> (w1422:refnum<file>)
                n836 = Format Date/Time String(time format string (%c)="%H:%M:%S:%3u") -> (date/time string=w1418:string)  [unwired: 2 in]
                n837 = Number To Fractional String(number=w1411, width (-)=w1416, precision (6)=w1416) -> (F-format string=w1410:string)  [unwired: 1 in]
                n838 = Concatenate Strings(w1418, "\t", w1410, "\r\n") -> (w1420:string)
                n839 = Format Into String(initial string=w1422, w1420) -> (resulting string=w1415:refnum<file>)  [unwired: 2 in, 1 out]
                n840 = local read "System Stop"() -> (w1413:bool)
              }
            }
            n841 = Wait (ms)(milliseconds to wait="NI DMM 2 Resistance Wait") -> ()  [unwired: 1 out]
            n842 = call <vilib>:"Simple Error Handler.vi"("error in (no error)"=w1384) -> ("error out"=w1383:errorcluster)  [unwired: 1 in, 7 out]
          }
        }
      }
      n843 = call <instrlib>:"niDMM Close.vi"("error in (no error)"=w1324, "instrument handle"=w1326) -> ("error out"=w1323:errorcluster)  [unwired: 9 in]
      n844 = local write "NI DMM 2 error out"(w1323) -> ()
      n845 = Close File(refnum=w1327) -> ()  [unwired: 1 in, 2 out]
      n846 = call <vilib>:"Simple Error Handler.vi"("error in (no error)"=w1323) -> ()  [unwired: 1 in, 8 out]
    }
  }
  n847 = case shown="True" w9 {
    tunnel: w21 -> [_ w1429]
    tunnel: w22 -> [_ w1426]
    tunnel: w10 -> [_ _]
    frame False {
    }
    frame True {
      n848 = local read "NI DMM 3 Option Return"() -> (w1423:enum32{"Ampermeter button", "Ohmmeter button"})
      n849 = case shown="\"Ampermeter button\", Default" w1423 {
        tunnel: w1429 -> [w1434 w1481]
        tunnel: [w1433 w1479] -> w1428
        tunnel: [w1432 w1478] -> w1427
        tunnel: w1426 -> [w1431 w1480]
        tunnel: [w1430 w1477] -> w1425
        frame "Ampermeter button", Default {
          n850 = while {
            tunnel: w1434 -> [w1446]
            tunnel: [w1444] -> w1433
            tunnel: [w1443] -> w1432
            tunnel: w1431 -> [w1441]
            tunnel: [w1437] -> w1430
            stop <- w1442 stop-if-true
            n851 = flat-sequence {
              tunnel: [w1450] -> w1447
              tunnel: w1446 -> [w1448]
              tunnel: w1441 -> [w1454]
              tunnel: [w1449] -> w1440
              tunnel: w1447 -> [w1456]
              tunnel: [w1462] -> w1445
              tunnel: w1440 -> [w1461]
              tunnel: [w1460] -> w1439
              tunnel: [w1457] -> w1435
              tunnel: w1445 -> [w1468]
              tunnel: [w1469] -> w1444
              tunnel: [w1468] -> w1443
              tunnel: [w1467] -> w1442
              tunnel: [w1466] -> w1438
              tunnel: w1439 -> [w1466]
              tunnel: w1435 -> [w1464]
              frame #0 {
                w1451 = T9 6.5 items=["3 1/2"=3.5, "4 1/2"=4.5, "5 1/2"=5.5, "6 1/2"=6.5, "7 1/2"=7.5] ("Resolution in Digits")
                n852 = Fract/Exp String To Number(string="NI DMM 3 Current Range") -> (number=w1453:dbl)  [unwired: 3 in, 1 out]
                n853 = call-poly <instrlib>:"niDMM Config Measurement.vi"("Range"=w1453, "Resolution in Digits"=w1451, "error in (no error)"=w1454, "Function"=niDMM_Function."DC Current" ("Measurement Type"), "instrument handle"=w1448) -> ("error out"=w1449:errorcluster, "instrument handle out"=w1450:refnum<k15>)  [unwired: 5 in]
              }
              frame #1 {
                n854 = call <instrlib>:"niDMM Read.vi"("error in (no error)"=w1461, "instrument handle"=w1456) -> ("error out"=w1460:errorcluster, "Measurement"=w1457:dbl, "instrument handle out"=w1462:refnum<k15>)  [unwired: 7 in]
                "DMM 3 Real Current" <- w1457
                n855 = Fract/Exp String To Number(string="NI DMM 3 units") -> (number=w1458:dbl)  [unwired: 3 in, 1 out]
                n856 = Multiply(x=w1458, y=w1457) -> (x*y=→"NI DMM 3 Current" →"NI DMM 3 Current Char":dbl)
              }
              frame #2 {
                w1470 = 15
                n857 = local read "NI DMM 3 Current output file"() -> (w1476:refnum<file>)
                n858 = Format Date/Time String(time format string (%c)="%H:%M:%S:%3u") -> (date/time string=w1472:string)  [unwired: 2 in]
                n859 = Number To Fractional String(number=w1464, width (-)=w1470, precision (6)=w1470) -> (F-format string=w1465:string)  [unwired: 1 in]
                n860 = Concatenate Strings(w1472, "\t", w1465, "\r\n") -> (w1474:string)
                n861 = Format Into String(initial string=w1476, w1474) -> (resulting string=w1469:refnum<file>)  [unwired: 2 in, 1 out]
                n862 = local read "System Stop"() -> (w1467:bool)
              }
            }
            n863 = Wait (ms)(milliseconds to wait="NI DMM 3 Current Wait") -> ()  [unwired: 1 out]
            n864 = call <vilib>:"Simple Error Handler.vi"("error in (no error)"=w1438) -> ("error out"=w1437:errorcluster)  [unwired: 1 in, 7 out]
          }
        }
        frame "Ohmmeter button" {
          n865 = while {
            tunnel: w1481 -> [w1493]
            tunnel: [w1491] -> w1479
            tunnel: [w1490] -> w1478
            tunnel: w1480 -> [w1488]
            tunnel: [w1484] -> w1477
            stop <- w1489 stop-if-true
            n866 = flat-sequence {
              tunnel: [w1500] -> w1494
              tunnel: w1493 -> [w1499]
              tunnel: w1488 -> [w1498]
              tunnel: [w1497] -> w1487
              tunnel: w1494 -> [w1505]
              tunnel: [w1504] -> w1492
              tunnel: w1487 -> [w1509]
              tunnel: [w1508] -> w1486
              tunnel: [w1503] -> w1482
              tunnel: w1492 -> [w1514]
              tunnel: [w1515] -> w1491
              tunnel: [w1514] -> w1490
              tunnel: [w1513] -> w1489
              tunnel: [w1512] -> w1485
              tunnel: w1486 -> [w1512]
              tunnel: w1482 -> [w1511]
              frame #0 {
                w1502 = T9 6.5 items=["3 1/2"=3.5, "4 1/2"=4.5, "5 1/2"=5.5, "6 1/2"=6.5, "7 1/2"=7.5] ("Resolution in Digits")
                n867 = Fract/Exp String To Number(string="NI DMM 3 Resistance Range") -> (number=w1496:dbl)  [unwired: 3 in, 1 out]
                n868 = call-poly <instrlib>:"niDMM Config Measurement.vi"("Range"=w1496, "Resolution in Digits"=w1502, "error in (no error)"=w1498, "Function"=niDMM_Function."2-wire Resistance" ("Measurement Type"), "instrument handle"=w1499) -> ("error out"=w1497:errorcluster, "instrument handle out"=w1500:refnum<k15>)  [unwired: 5 in]
              }
              frame #1 {
                n869 = call <instrlib>:"niDMM Read.vi"("error in (no error)"=w1509, "instrument handle"=w1505) -> ("error out"=w1508:errorcluster, "Measurement"=w1503:dbl, "instrument handle out"=w1504:refnum<k15>)  [unwired: 7 in]
                n870 = Fract/Exp String To Number(string="NI DMM 3 Resistance units") -> (number=w1506:dbl)  [unwired: 3 in, 1 out]
                n871 = Multiply(x=w1506, y=w1503) -> (x*y=→"NI DMM 3 Resistance" →"NI DMM 3 Resistance Char":dbl)
              }
              frame #2 {
                w1516 = 15
                n872 = local read "NI DMM 3 Resistance output file"() -> (w1523:refnum<file>)
                n873 = Format Date/Time String(time format string (%c)="%H:%M:%S:%3u") -> (date/time string=w1518:string)  [unwired: 2 in]
                n874 = Number To Fractional String(number=w1511, width (-)=w1516, precision (6)=w1516) -> (F-format string=w1521:string)  [unwired: 1 in]
                n875 = local read "System Stop"() -> (w1513:bool)
                n876 = Concatenate Strings(w1518, "\t", w1521, "\r\n") -> (w1520:string)
                n877 = Format Into String(initial string=w1523, w1520) -> (resulting string=w1515:refnum<file>)  [unwired: 2 in, 1 out]
              }
            }
            n878 = Wait (ms)(milliseconds to wait="NI DMM 3 Resistance Wait") -> ()  [unwired: 1 out]
            n879 = call <vilib>:"Simple Error Handler.vi"("error in (no error)"=w1485) -> ("error out"=w1484:errorcluster)  [unwired: 1 in, 7 out]
          }
        }
      }
      n880 = call <instrlib>:"niDMM Close.vi"("error in (no error)"=w1425, "instrument handle"=w1427) -> ("error out"=w1424:errorcluster)  [unwired: 9 in]
      n881 = local write "NI DMM 3 error out"(w1424) -> ()
      n882 = Close File(refnum=w1428) -> ()  [unwired: 1 in, 2 out]
      n883 = call <vilib>:"Simple Error Handler.vi"("error in (no error)"=w1424) -> ()  [unwired: 1 in, 8 out]
    }
  }
  n884 = case shown="True" w27 {
    tunnel: w10 -> [_ w1529]
    tunnel: w33 -> [_ w1525]
    tunnel: w30 -> [_ w1524]
    frame False {
    }
    frame True {
      n885 = while {
        tunnel: w1525 -> [w1556]
        tunnel: [w1561] -> w1528
        tunnel: [w1550] -> w1527
        tunnel: [w1535] -> w1526
        tunnel: w1529 -> [_]
        tunnel: w1524 -> [w1537]
        stop <- w1557 stop-if-true
        n886 = flat-sequence {
          tunnel: w1556 -> [w1569]
          tunnel: [w1566] -> w1545
          tunnel: w1537 -> [w1563]
          tunnel: [w1562] -> w1543
          tunnel: [w1576] -> w1560
          tunnel: w1545 -> [w1575]
          tunnel: w1543 -> [w1572]
          tunnel: [w1571] -> w1542
          tunnel: [w1585] -> w1559
          tunnel: w1560 -> [w1584]
          tunnel: w1542 -> [w1583]
          tunnel: [w1582] -> w1541
          tunnel: w1559 -> [w1589]
          tunnel: [w1588] -> w1558
          tunnel: w1541 -> [w1587]
          tunnel: [w1586] -> w1540
          tunnel: [w1606] -> w1554
          tunnel: w1558 -> [w1608]
          tunnel: [w1605] -> w1552
          tunnel: [w1598] -> w1548
          tunnel: [w1600] -> w1547
          tunnel: [w1599] -> w1546
          tunnel: [w1595] -> w1544
          tunnel: w1540 -> [w1594]
          tunnel: [w1593] -> w1538
          tunnel: w1554 -> [w1670]
          tunnel: [w1670] -> w1553
          tunnel: w1552 -> [w1653]
          tunnel: [w1660] -> w1551
          tunnel: [w1658] -> w1549
          tunnel: w1548 -> [w1657]
          tunnel: w1547 -> [w1656]
          tunnel: w1546 -> [w1655]
          tunnel: w1544 -> [w1651]
          tunnel: [w1648] -> w1539
          tunnel: w1538 -> [w1648]
          tunnel: [w1676] -> w1561
          tunnel: w1553 -> [w1676]
          tunnel: [w1677] -> w1557
          tunnel: w1551 -> [w1675]
          tunnel: [w1675] -> w1550
          tunnel: w1549 -> [_]
          tunnel: w1539 -> [w1674]
          tunnel: [w1674] -> w1536
          frame #0 {
            n887 = call <instrlib>:"niScope Configure Vertical.vi"("instrument handle"=w1569, "probe attenuation"=1.0 ("Probe Attenuation"), "vertical coupling"="AC/DC/Groun", "channels"="0" ("Channel Name"), "vertical range"="vertical range", "vertical offset"=0.0, "error in"=w1563) -> ("instrument handle out"=w1566:refnum<k15>, "error out"=w1562:errorcluster)  [unwired: 7 in]
          }
          frame #1 {
            w1581 = 0 items=["Positive", "Negative"] ("Trigger Slope")
            w1580 = u16 1 items=["AC"=0, "DC"=1, "HF Reject"=3, "LF Reject"=4, "AC Plus HF Reject"=1001] ("Coupling")
            n888 = call-poly <instrlib>:"niScope Configure Trigger (poly).vi"("instrument handle"=w1575, "trigger window mode"=w1581, "trigger coupling"=w1580, "trigger source"="Trigger Source", "low level"="Low Level", "high level"="High Level", "error in"=w1572, "trigger holdoff"=0.0, "trigger delay"=0.0 ("Trigger Delay")) -> ("instrument handle out"=w1576:refnum<k15>, "error out"=w1571:errorcluster)  [unwired: 5 in]
          }
          frame #2 {
            n889 = call <instrlib>:"niScope Initiate Acquisition.vi"("instrument handle"=w1584, "error in"=w1583) -> ("instrument handle out"=w1585:refnum<k15>, "error out"=w1582:errorcluster)  [unwired: 12 in]
          }
          frame #3 {
            n890 = call-poly <instrlib>:"niScope Fetch (poly).vi"("timeout"=1.0, "error in"=w1587, "channels"="0", "instrument handle"=w1589) -> ("error out"=w1586:errorcluster, "waveform"=→"RealTime Waveform":T4, "instrument handle out"=w1588:refnum<k15>)  [unwired: 4 in, 1 out]
          }
          frame #4 {
            # "Во время триггера FALSE"
            n891 = property class="niScope" props=["Auto Triggered", "Trigger Hysteresis"](reference=w1608) -> (reference out=w1607:refnum<k15>, "Auto Triggered"=w1604:bool)  [unwired: 1 in, 2 out]
            n892 = case shown="\"Radio Selection P1 CH1\"" "Channel for SEU" {
              tunnel: [w1610 w1616 w1618 w1622] -> w1600
              tunnel: [w1611 w1615 w1619 w1623] -> w1599
              tunnel: [w1612 w1614 w1620 w1624] -> w1598
              tunnel: [w1609 w1613 w1617 w1621] -> w1596
              frame "Radio Selection P1 CH0", Default {
                n893 = local read "P1 CH0_warning"() -> (w1609:bool)
                n894 = local read "P1 CH0_cur, A"() -> (w1610:dbl)
                n895 = local read "P1 CH0, V"() -> (w1611:dbl)
                n896 = Get Date/Time In Seconds() -> (seconds since 1Jan1904=w1612:timestamp)
              }
              frame "Radio Selection P1 CH1" {
                n897 = local read "P1 CH1_warning"() -> (w1613:bool)
                n898 = local read "P1 CH1_cur, A"() -> (w1616:dbl)
                n899 = local read "P1 CH1, V"() -> (w1615:dbl)
                n900 = Get Date/Time In Seconds() -> (seconds since 1Jan1904=w1614:timestamp)
              }
              frame "Radio Selection P2 CH0" {
                n901 = local read "P2 CH0_warning"() -> (w1617:bool)
                n902 = local read "P2 CH0_cur, A"() -> (w1618:dbl)
                n903 = local read "P2 CH0, V"() -> (w1619:dbl)
                n904 = Get Date/Time In Seconds() -> (seconds since 1Jan1904=w1620:timestamp)
              }
              frame "Radio Selection P2 CH1" {
                n905 = local read "P1 CH1_warning"() -> (w1621:bool)
                n906 = local read "P2 CH1_cur, A"() -> (w1622:dbl)
                n907 = local read "P2 CH1, V"() -> (w1623:dbl)
                n908 = Get Date/Time In Seconds() -> (seconds since 1Jan1904=w1624:timestamp)
              }
            }
            n909 = Not(x=w1604) -> (.not. x?=w1603:bool)
            n910 = Not(x=w1596) -> (.not. x?=w1601:bool)
            n911 = And(x=w1601, y=w1603) -> (x .and. y?=w1602:bool)
            n912 = case shown="True" w1602 {
              tunnel: w1607 -> [w1628 w1643]
              tunnel: [w1628 w1635] -> w1606
              tunnel: [FALSE TRUE] -> w1605
              tunnel: ["" w1632] -> w1595
              tunnel: w1594 -> [w1625 w1631]
              tunnel: [w1625 w1629] -> w1593
              frame False {
              }
              frame True {
                w1634 = 6
                # "Регистрация SEU"
                n913 = call-poly <instrlib>:"niScope Fetch (poly).vi"("timeout"=1.0, "error in"=w1631, "channels"="0", "instrument handle"=w1643) -> ("error out"=w1630:errorcluster, "waveform"=→"SEU Waveform":T4, "instrument handle out"=w1636:refnum<k15>)  [unwired: 4 in, 1 out]
                n914 = call-poly <instrlib>:"niScope Fetch (poly).vi"("timeout"=1.0, "error in"=w1630, "numSamples"=1, "channels"="0", "instrument handle"=w1636) -> ("error out"=w1629:errorcluster, "wfm"=w1641:dbl[], "instrument handle out"=w1635:refnum<k15>)  [unwired: 3 in, 1 out]
                n915 = Index Array(array=w1641, index=0) -> (element=w1633:dbl)
                "SEU Last Level" <- w1633
                n916 = Number To Fractional String(number=w1633, width (-)=w1634, precision (6)=w1634) -> (F-format string=w1632:string)  [unwired: 1 in]
              }
            }
          }
          frame #5 {
            w1661 = 6
            w1665 = 0
            w1664 = 6
            w1652 = "\t"
            # "Регистрация SEU"
            n917 = case shown="True" w1653 {
              tunnel: [w1671 w1672] -> w1654
              frame False {
                n918 = local read "SEU_Counter"() -> (w1671:u32)
              }
              frame True {
                n919 = local read "SEU_Counter"() -> (w1673:u32)
                n920 = Increment(x=w1673) -> (x+1=w1672:u32)
                "SEU_Counter" <- w1672
              }
            }
            n921 = Format Date/Time String(time format string (%c)="%H:%M:%S:%3u", seconds (now)=w1657) -> (date/time string=w1667:string)  [unwired: 1 in]
            n922 = local read "SEU output file refnum"() -> (w1647:refnum<file>)
            n923 = Number To Fractional String(number=w1655, width (-)=w1661, precision (6)=w1661) -> (F-format string=w1666:string)  [unwired: 1 in]
            n924 = Number To Fractional String(number=w1656, width (-)=w1664, precision (6)=w1664) -> (F-format string=w1668:string)  [unwired: 1 in]
            n925 = Number To Fractional String(number=w1654, width (-)=w1665, precision (6)=w1665) -> (F-format string=w1669:string)  [unwired: 1 in]
            n926 = Select(t="???", s=w1653, f="") -> (s? t:f=w1650:string)
            n927 = Concatenate Strings(w1667, w1652, w1666, w1652, w1668, w1652, w1669, w1652, w1651, w1652, w1650, "\r\n") -> (w1658:string)
            n928 = Format Into String(initial string=w1647, w1658) -> (resulting string=w1660:refnum<file>)  [unwired: 2 in, 1 out]
            "SEU_warning" <- w1653
            "SEU" <- w1653
          }
          frame #6 {
            n929 = local read "System Stop"() -> (w1677:bool)
          }
        }
        n930 = Wait (ms)(milliseconds to wait=u32 1) -> ()  [unwired: 1 out]
        n931 = call <vilib>:"Simple Error Handler.vi"("error in (no error)"=w1536) -> ("error out"=w1535:errorcluster)  [unwired: 1 in, 7 out]
        "NI Scope error out" <- w1535
      }
      n932 = flat-sequence {
        tunnel: w1528 -> [w1534]
        tunnel: w1527 -> [w1533]
        tunnel: w1526 -> [w1532]
        frame #0 {
          n933 = Close File(refnum=w1533) -> ()  [unwired: 1 in, 2 out]
          n934 = call <instrlib>:"niScope Close.vi"("instrument handle"=w1534, "error in"=w1532) -> ("error out"=w1531:errorcluster)  [unwired: 13 in]
          n935 = call <vilib>:"Simple Error Handler.vi"("error in (no error)"=w1531) -> ("error out"=w1530:errorcluster)  [unwired: 1 in, 7 out]
          n936 = local write "NI Scope error out"(w1530) -> ()
        }
      }
    }
  }
  n937 = case shown="True" w2 {
    tunnel: w7 -> [w1678 w1683]
    tunnel: w6 -> [w1679 w1682]
    tunnel: [w1679 w1681] -> w5
    tunnel: [w1678 w1680] -> w4
    frame False {
    }
    frame True {
      n938 = while {
        tunnel: [w1689] -> _
        tunnel: w1683 -> [w1688]
        tunnel: w1682 -> [w1687]
        tunnel: [w1686] -> w1681
        tunnel: [w1684] -> w1680
        stop <- w1689 stop-if-true
        n939 = Wait (ms)(milliseconds to wait=u32 1) -> ()  [unwired: 1 out]
        n940 = flat-sequence {
          tunnel: [w1695] -> w1689
          tunnel: w1688 -> [w1694]
          tunnel: w1687 -> [w1693]
          tunnel: [w1692] -> w1686
          tunnel: [w1691] -> w1685
          frame #0 {
            w1696 = T10 0 items=["Current", "Voltage"] ("measurement type")
            n941 = call <instrlib>:"niDCPower Configure Current Limit.vi"("current limit"="P2 CH0_curlim, A", "channel name"="0", "instrument handle"=w1693) -> ("error out"=w1721:errorcluster, "instrument handle out"=w1740:refnum<k15>)  [unwired: 7 in]
            n942 = call <instrlib>:"niDCPower Configure Current Limit.vi"("error in (no error)"=w1694, "current limit"="P2 CH1_curlim, A", "channel name"="1", "instrument handle"=w1693) -> ("instrument handle out"=w1726:refnum<k15>)  [unwired: 6 in, 1 out]
            n943 = call <instrlib>:"niDCPower Configure Current Limit.vi"("current limit"="P2 CH2_curlim, A", "channel name"="2", "instrument handle"=w1693) -> ("instrument handle out"=w1706:refnum<k15>)  [unwired: 7 in, 1 out]
            n944 = local read "Power OFF"() -> (w1723:bool)
            n945 = local read "Power OFF"() -> (w1709:bool)
            n946 = local read "Power OFF"() -> (w1733:bool)
            n947 = call <instrlib>:"niDCPower Configure Voltage Level.vi"("error in (no error)"=w1721, "voltage level"="P2 CH0, V", "channel name"="0", "instrument handle"=w1740) -> ("error out"=w1737:errorcluster, "instrument handle out"=w1736:refnum<k15>)  [unwired: 6 in]
            n948 = call <instrlib>:"niDCPower Configure Voltage Level.vi"("voltage level"="P2 CH1, V", "channel name"="1", "instrument handle"=w1726) -> ("instrument handle out"=w1729:refnum<k15>)  [unwired: 7 in, 1 out]
            n949 = call <instrlib>:"niDCPower Configure Voltage Level.vi"("voltage level"="P2 CH2, V", "channel name"="2", "instrument handle"=w1706) -> ("instrument handle out"=w1703:refnum<k15>)  [unwired: 7 in, 1 out]
            n950 = Select(t=FALSE, s=w1723, f="P2 CH1") -> (s? t:f=w1722:bool)
            n951 = Select(t=FALSE, s=w1709, f="P2 CH2") -> (s? t:f=w1710:bool)
            n952 = Select(t=FALSE, s=w1733, f="P2 CH0") -> (s? t:f=w1732:bool)
            n953 = call <instrlib>:"niDCPower Configure Output Enabled.vi"("error in (no error)"=w1737, "output enabled"=w1732, "channel name"="0", "instrument handle"=w1736) -> ("error out"=w1734:errorcluster, "instrument handle out"=w1735:refnum<k15>)  [unwired: 6 in]
            n954 = call <instrlib>:"niDCPower Configure Output Enabled.vi"("output enabled"=w1722, "channel name"="1", "instrument handle"=w1729) -> ("instrument handle out"=w1730:refnum<k15>)  [unwired: 7 in, 1 out]
            n955 = call <instrlib>:"niDCPower Configure Output Enabled.vi"("output enabled"=w1710, "channel name"="2", "instrument handle"=w1703) -> ("instrument handle out"=w1702:refnum<k15>)  [unwired: 7 in, 1 out]
            n956 = call <instrlib>:"niDCPower Measure.vi"("error in (no error)"=w1734, "measurement type"=w1696, "channel name"="0", "instrument handle"=w1735) -> ("error out"=w1691:errorcluster, "measurement"=→"P2 CH0_cur, A" →"P2 CH0_char":dbl, "instrument handle out"=w1692:refnum<k15>)  [unwired: 5 in]
            n957 = call <instrlib>:"niDCPower Measure.vi"("measurement type"=w1696, "channel name"="1", "instrument handle"=w1730) -> ("measurement"=→"P2 CH1_cur, A" →"P2 CH1_char":dbl)  [unwired: 6 in, 2 out]
            n958 = call <instrlib>:"niDCPower Measure.vi"("measurement type"=w1696, "channel name"="2", "instrument handle"=w1702) -> ("measurement"=→"P2 CH2_cur, A" →"P2 CH2_char":dbl)  [unwired: 6 in, 2 out]
            n959 = local read "Power OFF"() -> (w1695:bool)
          }
        }
        n960 = call <vilib>:"Simple Error Handler.vi"("error in (no error)"=w1685) -> ("error out"=w1684:errorcluster)  [unwired: 1 in, 7 out]
        "DC Power 2 error out" <- w1684
      }
    }
  }
  n961 = case shown="True" w3 {
    tunnel: [w1743 w1748] -> w37
    tunnel: w36 -> [w1743 w1747]
    tunnel: [w1742 w1746] -> w35
    tunnel: w34 -> [w1742 w1745]
    tunnel: w8 -> [_ w1744]
    frame False {
    }
    frame True {
      n962 = while {
        tunnel: w1747 -> [w1755]
        tunnel: [w1754] -> _
        tunnel: [w1752] -> w1748
        tunnel: [w1749] -> w1746
        tunnel: w1745 -> [w1751]
        tunnel: w1744 -> [_]
        stop <- w1754 stop-if-true
        # "Инициализация источников"
        n963 = Wait (ms)(milliseconds to wait=u32 1) -> ()  [unwired: 1 out]
        n964 = flat-sequence {
          tunnel: w1755 -> [w1756]
          tunnel: [w1784] -> w1754
          tunnel: [w1775] -> w1752
          tunnel: [w1774] -> w1750
          tunnel: w1751 -> [w1773]
          frame #0 {
            w1757 = T10 0 items=["Current", "Voltage"] ("measurement type")
            n965 = local read "Power OFF"() -> (w1777:bool)
            n966 = call <instrlib>:"niDCPower Configure Current Limit.vi"("current limit"="P1 CH2_curlim, A", "channel name"="2", "instrument handle"=w1756) -> ("instrument handle out"=w1763:refnum<k15>)  [unwired: 7 in, 1 out]
            n967 = call <instrlib>:"niDCPower Configure Current Limit.vi"("error in (no error)"=w1773, "current limit"="P1 CH0_curlim, A", "channel name"="0", "instrument handle"=w1756) -> ("error out"=w1772:errorcluster, "instrument handle out"=w1798:refnum<k15>)  [unwired: 6 in]
            n968 = call <instrlib>:"niDCPower Configure Current Limit.vi"("current limit"="P1 CH1_curlim, A", "channel name"="1", "instrument handle"=w1756) -> ("instrument handle out"=w1795:refnum<k15>)  [unwired: 7 in, 1 out]
            n969 = local read "Power OFF"() -> (w1783:bool)
            n970 = local read "Power OFF"() -> (w1769:bool)
            n971 = call <instrlib>:"niDCPower Configure Voltage Level.vi"("voltage level"="P1 CH2, V", "channel name"="2", "instrument handle"=w1763) -> ("instrument handle out"=w1766:refnum<k15>)  [unwired: 7 in, 1 out]
            n972 = call <instrlib>:"niDCPower Configure Voltage Level.vi"("error in (no error)"=w1772, "voltage level"="P1 CH0, V", "channel name"="0", "instrument handle"=w1798) -> ("error out"=w1802:errorcluster, "instrument handle out"=w1803:refnum<k15>)  [unwired: 6 in]
            n973 = call <instrlib>:"niDCPower Configure Voltage Level.vi"("voltage level"="P1 CH1, V", "channel name"="1", "instrument handle"=w1795) -> ("instrument handle out"=w1801:refnum<k15>)  [unwired: 7 in, 1 out]
            n974 = Select(t=FALSE, s=w1777, f="P1 CH0") -> (s? t:f=w1776:bool)
            n975 = Select(t=FALSE, s=w1783, f="P1 CH1") -> (s? t:f=w1780:bool)
            n976 = Select(t=FALSE, s=w1769, f="P1 CH2") -> (s? t:f=w1770:bool)
            n977 = call <instrlib>:"niDCPower Configure Output Enabled.vi"("output enabled"=w1770, "channel name"="2", "instrument handle"=w1766) -> ("instrument handle out"=w1767:refnum<k15>)  [unwired: 7 in, 1 out]
            n978 = call <instrlib>:"niDCPower Configure Output Enabled.vi"("error in (no error)"=w1802, "output enabled"=w1776, "channel name"="0", "instrument handle"=w1803) -> ("error out"=w1805:errorcluster, "instrument handle out"=w1804:refnum<k15>)  [unwired: 6 in]
            n979 = call <instrlib>:"niDCPower Configure Output Enabled.vi"("output enabled"=w1780, "channel name"="1", "instrument handle"=w1801) -> ("instrument handle out"=w1806:refnum<k15>)  [unwired: 7 in, 1 out]
            n980 = call <instrlib>:"niDCPower Measure.vi"("measurement type"=w1757, "channel name"="2", "instrument handle"=w1767) -> ("measurement"=→"P1 CH2_cur, A" →"P1 CH2_char":dbl)  [unwired: 6 in, 2 out]
            n981 = call <instrlib>:"niDCPower Measure.vi"("error in (no error)"=w1805, "measurement type"=w1757, "channel name"="0", "instrument handle"=w1804) -> ("error out"=w1774:errorcluster, "measurement"=→"P1 CH0_cur, A" →"P1 CH0_char":dbl, "instrument handle out"=w1775:refnum<k15>)  [unwired: 5 in]
            n982 = call <instrlib>:"niDCPower Measure.vi"("measurement type"=w1757, "channel name"="1", "instrument handle"=w1806) -> ("measurement"=→"P1 CH1_cur, A" →"P1 CH1_char":dbl)  [unwired: 6 in, 2 out]
            n983 = local read "Power OFF"() -> (w1784:bool)
          }
        }
        n984 = call <vilib>:"Simple Error Handler.vi"("error in (no error)"=w1750) -> ("error out"=w1749:errorcluster)  [unwired: 1 in, 7 out]
        "DC Power 1 error out" <- w1749
      }
    }
  }
  n985 = while {
    tunnel: w10 -> [_]
    stop <- w1826 stop-if-true
    n986 = Wait (ms)(milliseconds to wait=u32 100) -> ()  [unwired: 1 out]
    n987 = local read "System Stop"() -> (w1819:bool)
    n988 = local read "System Stop"() -> (w1816:bool)
    n989 = Or(x="P2 CH0 Used", y=w1819) -> (x .or. y?=w1821:bool)
    n990 = Or(x="P1 CH0 Used", y=w1816) -> (x .or. y?=w1818:bool)
    n991 = case shown="True" w1818 {
      frame False {
        w1833 = T7."Disabled and Grayed Out" ("Disabled")
        n992 = property on="P1 CH0" class="Bool (strict)"("DisabledEnum"=w1833) -> ()  [unwired: 2 in, 2 out]
        n993 = property on="P1 CH0_char" class="WFChart (strict)"("DisabledEnum"=w1833) -> ()  [unwired: 2 in, 2 out]
        n994 = property on="P1 CH0, V" class="DigNum (strict)"("DisabledEnum"=w1833) -> ()  [unwired: 2 in, 2 out]
        n995 = property on="P1 CH0_curlim, A" class="DigNum (strict)"("DisabledEnum"=w1833) -> ()  [unwired: 2 in, 2 out]
        n996 = property on="P1 CH0_cur, A" class="DigNum (strict)"("DisabledEnum"=w1833) -> ()  [unwired: 2 in, 2 out]
        n997 = property on="P1 CH0_selcur, A" class="DigNum (strict)"("DisabledEnum"=w1833) -> ()  [unwired: 2 in, 2 out]
        n998 = property on="P1 CH0_counter" class="DigNum (strict)"("DisabledEnum"=w1833) -> ()  [unwired: 2 in, 2 out]
        n999 = property on="P1 CH0_warning" class="Bool (strict)"("DisabledEnum"=w1833) -> ()  [unwired: 2 in, 2 out]
      }
      frame True {
        w1834 = T7."Enabled" ("Disabled")
        n1000 = property on="P1 CH0" class="Bool (strict)"("DisabledEnum"=w1834) -> ()  [unwired: 2 in, 2 out]
        n1001 = property on="P1 CH0_char" class="WFChart (strict)"("DisabledEnum"=w1834) -> ()  [unwired: 2 in, 2 out]
        n1002 = property on="P1 CH0, V" class="DigNum (strict)"("DisabledEnum"=w1834) -> ()  [unwired: 2 in, 2 out]
        n1003 = property on="P1 CH0_curlim, A" class="DigNum (strict)"("DisabledEnum"=w1834) -> ()  [unwired: 2 in, 2 out]
        n1004 = property on="P1 CH0_cur, A" class="DigNum (strict)"("DisabledEnum"=w1834) -> ()  [unwired: 2 in, 2 out]
        n1005 = property on="P1 CH0_selcur, A" class="DigNum (strict)"("DisabledEnum"=w1834) -> ()  [unwired: 2 in, 2 out]
        n1006 = property on="P1 CH0_counter" class="DigNum (strict)"("DisabledEnum"=w1834) -> ()  [unwired: 2 in, 2 out]
        n1007 = property on="P1 CH0_warning" class="Bool (strict)"("DisabledEnum"=w1834) -> ()  [unwired: 2 in, 2 out]
      }
    }
    n1008 = case shown="True" w1821 {
      frame False {
        w1835 = T7."Disabled and Grayed Out" ("Disabled")
        n1009 = property on="P2 CH0" class="Bool (strict)"("DisabledEnum"=w1835) -> ()  [unwired: 2 in, 2 out]
        n1010 = property on="P2 CH0_char" class="WFChart (strict)"("DisabledEnum"=w1835) -> ()  [unwired: 2 in, 2 out]
        n1011 = property on="P2 CH0, V" class="DigNum (strict)"("DisabledEnum"=w1835) -> ()  [unwired: 2 in, 2 out]
        n1012 = property on="P2 CH0_curlim, A" class="DigNum (strict)"("DisabledEnum"=w1835) -> ()  [unwired: 2 in, 2 out]
        n1013 = property on="P2 CH0_cur, A" class="DigNum (strict)"("DisabledEnum"=w1835) -> ()  [unwired: 2 in, 2 out]
        n1014 = property on="P2 CH0_selcur, A" class="DigNum (strict)"("DisabledEnum"=w1835) -> ()  [unwired: 2 in, 2 out]
        n1015 = property on="P2 CH0_counter" class="DigNum (strict)"("DisabledEnum"=w1835) -> ()  [unwired: 2 in, 2 out]
        n1016 = property on="P2 CH0_warning" class="Bool (strict)"("DisabledEnum"=w1835) -> ()  [unwired: 2 in, 2 out]
      }
      frame True {
        w1836 = T7."Enabled" ("Disabled")
        n1017 = property on="P2 CH0" class="Bool (strict)"("DisabledEnum"=w1836) -> ()  [unwired: 2 in, 2 out]
        n1018 = property on="P2 CH0_char" class="WFChart (strict)"("DisabledEnum"=w1836) -> ()  [unwired: 2 in, 2 out]
        n1019 = property on="P2 CH0, V" class="DigNum (strict)"("DisabledEnum"=w1836) -> ()  [unwired: 2 in, 2 out]
        n1020 = property on="P2 CH0_curlim, A" class="DigNum (strict)"("DisabledEnum"=w1836) -> ()  [unwired: 2 in, 2 out]
        n1021 = property on="P2 CH0_cur, A" class="DigNum (strict)"("DisabledEnum"=w1836) -> ()  [unwired: 2 in, 2 out]
        n1022 = property on="P2 CH0_selcur, A" class="DigNum (strict)"("DisabledEnum"=w1836) -> ()  [unwired: 2 in, 2 out]
        n1023 = property on="P2 CH0_counter" class="DigNum (strict)"("DisabledEnum"=w1836) -> ()  [unwired: 2 in, 2 out]
        n1024 = property on="P2 CH0_warning" class="Bool (strict)"("DisabledEnum"=w1836) -> ()  [unwired: 2 in, 2 out]
      }
    }
    n1025 = local read "System Stop"() -> (w1822:bool)
    n1026 = local read "System Stop"() -> (w1813:bool)
    n1027 = Or(x="P2 CH1 Used", y=w1822) -> (x .or. y?=w1823:bool)
    n1028 = Or(x="P1 CH1 Used", y=w1813) -> (x .or. y?=w1815:bool)
    n1029 = case shown="True" w1823 {
      frame False {
        w1837 = T7."Disabled and Grayed Out" ("Disabled")
        n1030 = property on="P2 CH1" class="Bool (strict)"("DisabledEnum"=w1837) -> ()  [unwired: 2 in, 2 out]
        n1031 = property on="P2 CH1_char" class="WFChart (strict)"("DisabledEnum"=w1837) -> ()  [unwired: 2 in, 2 out]
        n1032 = property on="P2 CH1, V" class="DigNum (strict)"("DisabledEnum"=w1837) -> ()  [unwired: 2 in, 2 out]
        n1033 = property on="P2 CH1_curlim, A" class="DigNum (strict)"("DisabledEnum"=w1837) -> ()  [unwired: 2 in, 2 out]
        n1034 = property on="P2 CH1_cur, A" class="DigNum (strict)"("DisabledEnum"=w1837) -> ()  [unwired: 2 in, 2 out]
        n1035 = property on="P2 CH1_selcur, A" class="DigNum (strict)"("DisabledEnum"=w1837) -> ()  [unwired: 2 in, 2 out]
        n1036 = property on="P2 CH1_counter" class="DigNum (strict)"("DisabledEnum"=w1837) -> ()  [unwired: 2 in, 2 out]
        n1037 = property on="P2 CH1_warning" class="Bool (strict)"("DisabledEnum"=w1837) -> ()  [unwired: 2 in, 2 out]
      }
      frame True {
        w1838 = T7."Enabled" ("Disabled")
        n1038 = property on="P2 CH1" class="Bool (strict)"("DisabledEnum"=w1838) -> ()  [unwired: 2 in, 2 out]
        n1039 = property on="P2 CH1_char" class="WFChart (strict)"("DisabledEnum"=w1838) -> ()  [unwired: 2 in, 2 out]
        n1040 = property on="P2 CH1, V" class="DigNum (strict)"("DisabledEnum"=w1838) -> ()  [unwired: 2 in, 2 out]
        n1041 = property on="P2 CH1_curlim, A" class="DigNum (strict)"("DisabledEnum"=w1838) -> ()  [unwired: 2 in, 2 out]
        n1042 = property on="P2 CH1_cur, A" class="DigNum (strict)"("DisabledEnum"=w1838) -> ()  [unwired: 2 in, 2 out]
        n1043 = property on="P2 CH1_selcur, A" class="DigNum (strict)"("DisabledEnum"=w1838) -> ()  [unwired: 2 in, 2 out]
        n1044 = property on="P2 CH1_counter" class="DigNum (strict)"("DisabledEnum"=w1838) -> ()  [unwired: 2 in, 2 out]
        n1045 = property on="P2 CH1_warning" class="Bool (strict)"("DisabledEnum"=w1838) -> ()  [unwired: 2 in, 2 out]
      }
    }
    n1046 = case shown="True" w1815 {
      frame False {
        w1831 = T7."Disabled and Grayed Out" ("Disabled")
        n1047 = property on="P1 CH1" class="Bool (strict)"("DisabledEnum"=w1831) -> ()  [unwired: 2 in, 2 out]
        n1048 = property on="P1 CH1_char" class="WFChart (strict)"("DisabledEnum"=w1831) -> ()  [unwired: 2 in, 2 out]
        n1049 = property on="P1 CH1, V" class="DigNum (strict)"("DisabledEnum"=w1831) -> ()  [unwired: 2 in, 2 out]
        n1050 = property on="P1 CH1_curlim, A" class="DigNum (strict)"("DisabledEnum"=w1831) -> ()  [unwired: 2 in, 2 out]
        n1051 = property on="P1 CH1_cur, A" class="DigNum (strict)"("DisabledEnum"=w1831) -> ()  [unwired: 2 in, 2 out]
        n1052 = property on="P1 CH1_selcur, A" class="DigNum (strict)"("DisabledEnum"=w1831) -> ()  [unwired: 2 in, 2 out]
        n1053 = property on="P1 CH1_counter" class="DigNum (strict)"("DisabledEnum"=w1831) -> ()  [unwired: 2 in, 2 out]
        n1054 = property on="P1 CH1_warning" class="Bool (strict)"("DisabledEnum"=w1831) -> ()  [unwired: 2 in, 2 out]
      }
      frame True {
        w1832 = T7."Enabled" ("Disabled")
        n1055 = property on="P1 CH1" class="Bool (strict)"("DisabledEnum"=w1832) -> ()  [unwired: 2 in, 2 out]
        n1056 = property on="P1 CH1_char" class="WFChart (strict)"("DisabledEnum"=w1832) -> ()  [unwired: 2 in, 2 out]
        n1057 = property on="P1 CH1, V" class="DigNum (strict)"("DisabledEnum"=w1832) -> ()  [unwired: 2 in, 2 out]
        n1058 = property on="P1 CH1_curlim, A" class="DigNum (strict)"("DisabledEnum"=w1832) -> ()  [unwired: 2 in, 2 out]
        n1059 = property on="P1 CH1_cur, A" class="DigNum (strict)"("DisabledEnum"=w1832) -> ()  [unwired: 2 in, 2 out]
        n1060 = property on="P1 CH1_selcur, A" class="DigNum (strict)"("DisabledEnum"=w1832) -> ()  [unwired: 2 in, 2 out]
        n1061 = property on="P1 CH1_counter" class="DigNum (strict)"("DisabledEnum"=w1832) -> ()  [unwired: 2 in, 2 out]
        n1062 = property on="P1 CH1_warning" class="Bool (strict)"("DisabledEnum"=w1832) -> ()  [unwired: 2 in, 2 out]
      }
    }
    n1063 = local read "System Stop"() -> (w1809:bool)
    n1064 = local read "System Stop"() -> (w1812:bool)
    n1065 = Or(x="P1 CH2 Used", y=w1812) -> (x .or. y?=w1810:bool)
    n1066 = Or(x="P2 CH2 Used", y=w1809) -> (x .or. y?=w1808:bool)
    n1067 = case shown="True" w1810 {
      frame False {
        w1829 = T7."Disabled and Grayed Out" ("Disabled")
        n1068 = property on="P1 CH2" class="Bool (strict)"("DisabledEnum"=w1829) -> ()  [unwired: 2 in, 2 out]
        n1069 = property on="P1 CH2_char" class="WFChart (strict)"("DisabledEnum"=w1829) -> ()  [unwired: 2 in, 2 out]
        n1070 = property on="P1 CH2, V" class="DigNum (strict)"("DisabledEnum"=w1829) -> ()  [unwired: 2 in, 2 out]
        n1071 = property on="P1 CH2_curlim, A" class="DigNum (strict)"("DisabledEnum"=w1829) -> ()  [unwired: 2 in, 2 out]
        n1072 = property on="P1 CH2_cur, A" class="DigNum (strict)"("DisabledEnum"=w1829) -> ()  [unwired: 2 in, 2 out]
        n1073 = property on="P1 CH2_selcur, A" class="DigNum (strict)"("DisabledEnum"=w1829) -> ()  [unwired: 2 in, 2 out]
        n1074 = property on="P1 CH2_counter" class="DigNum (strict)"("DisabledEnum"=w1829) -> ()  [unwired: 2 in, 2 out]
        n1075 = property on="P1 CH2_warning" class="Bool (strict)"("DisabledEnum"=w1829) -> ()  [unwired: 2 in, 2 out]
      }
      frame True {
        w1830 = T7."Enabled" ("Disabled")
        n1076 = property on="P1 CH2_char" class="WFChart (strict)"("DisabledEnum"=w1830) -> ()  [unwired: 2 in, 2 out]
        n1077 = property on="P1 CH2, V" class="DigNum (strict)"("DisabledEnum"=w1830) -> ()  [unwired: 2 in, 2 out]
        n1078 = property on="P1 CH2_curlim, A" class="DigNum (strict)"("DisabledEnum"=w1830) -> ()  [unwired: 2 in, 2 out]
        n1079 = property on="P1 CH2_cur, A" class="DigNum (strict)"("DisabledEnum"=w1830) -> ()  [unwired: 2 in, 2 out]
        n1080 = property on="P1 CH2_selcur, A" class="DigNum (strict)"("DisabledEnum"=w1830) -> ()  [unwired: 2 in, 2 out]
        n1081 = property on="P1 CH2_counter" class="DigNum (strict)"("DisabledEnum"=w1830) -> ()  [unwired: 2 in, 2 out]
        n1082 = property on="P1 CH2_warning" class="Bool (strict)"("DisabledEnum"=w1830) -> ()  [unwired: 2 in, 2 out]
        n1083 = property on="P1 CH2" class="Bool (strict)"("DisabledEnum"=w1830) -> ()  [unwired: 2 in, 2 out]
      }
    }
    n1084 = case shown="True" w1808 {
      frame False {
        w1827 = T7."Disabled and Grayed Out" ("Disabled")
        n1085 = property on="P2 CH2" class="Bool (strict)"("DisabledEnum"=w1827) -> ()  [unwired: 2 in, 2 out]
        n1086 = property on="P2 CH2_char" class="WFChart (strict)"("DisabledEnum"=w1827) -> ()  [unwired: 2 in, 2 out]
        n1087 = property on="P2 CH2, V" class="DigNum (strict)"("DisabledEnum"=w1827) -> ()  [unwired: 2 in, 2 out]
        n1088 = property on="P2 CH2_curlim, A" class="DigNum (strict)"("DisabledEnum"=w1827) -> ()  [unwired: 2 in, 2 out]
        n1089 = property on="P2 CH2_cur, A" class="DigNum (strict)"("DisabledEnum"=w1827) -> ()  [unwired: 2 in, 2 out]
        n1090 = property on="P2 CH2_selcur, A" class="DigNum (strict)"("DisabledEnum"=w1827) -> ()  [unwired: 2 in, 2 out]
        n1091 = property on="P2 CH2_counter" class="DigNum (strict)"("DisabledEnum"=w1827) -> ()  [unwired: 2 in, 2 out]
        n1092 = property on="P2 CH2_warning" class="Bool (strict)"("DisabledEnum"=w1827) -> ()  [unwired: 2 in, 2 out]
      }
      frame True {
        w1828 = T7."Enabled" ("Disabled")
        n1093 = property on="P2 CH2" class="Bool (strict)"("DisabledEnum"=w1828) -> ()  [unwired: 2 in, 2 out]
        n1094 = property on="P2 CH2_char" class="WFChart (strict)"("DisabledEnum"=w1828) -> ()  [unwired: 2 in, 2 out]
        n1095 = property on="P2 CH2, V" class="DigNum (strict)"("DisabledEnum"=w1828) -> ()  [unwired: 2 in, 2 out]
        n1096 = property on="P2 CH2_curlim, A" class="DigNum (strict)"("DisabledEnum"=w1828) -> ()  [unwired: 2 in, 2 out]
        n1097 = property on="P2 CH2_cur, A" class="DigNum (strict)"("DisabledEnum"=w1828) -> ()  [unwired: 2 in, 2 out]
        n1098 = property on="P2 CH2_selcur, A" class="DigNum (strict)"("DisabledEnum"=w1828) -> ()  [unwired: 2 in, 2 out]
        n1099 = property on="P2 CH2_counter" class="DigNum (strict)"("DisabledEnum"=w1828) -> ()  [unwired: 2 in, 2 out]
        n1100 = property on="P2 CH2_warning" class="Bool (strict)"("DisabledEnum"=w1828) -> ()  [unwired: 2 in, 2 out]
      }
    }
    n1101 = local read "System Stop"() -> (w1826:bool)
  }
  n1102 = while {
    shift-right: [w1858] -> _
    shift-left: FALSE -> [w1864]
    shift-right: [w1857] -> _
    shift-left: FALSE -> [w1863]
    shift-right: [w1859] -> _
    shift-left: FALSE -> [w1862]
    shift-right: [w1860] -> _
    shift-left: FALSE -> [w1861]
    shift-right: [w1853] -> _
    shift-left: FALSE -> [w1854]
    shift-right: [w1851] -> _
    shift-left: FALSE -> [w1852]
    shift-right: [w1849] -> _
    shift-left: FALSE -> [w1850]
    shift-right: [w1847] -> _
    shift-left: FALSE -> [w1848]
    tunnel: w10 -> [_]
    shift-right: [w1844] -> _
    shift-left: FALSE -> [w1843]
    shift-right: [w1846] -> _
    shift-left: FALSE -> [w1845]
    shift-right: [w1841] -> _
    shift-left: FALSE -> [w1842]
    shift-right: [w1839] -> _
    shift-left: FALSE -> [w1840]
    stop <- w1855 stop-if-true
    # "Включение / выключение каналов"
    n1103 = stacked-sequence {
      tunnel: w1864 -> [w1930 _]
      tunnel: [w1926 _] -> w1858
      tunnel: w1863 -> [w1922 _]
      tunnel: [w1921 _] -> w1857
      tunnel: w1862 -> [w1920 _]
      tunnel: w1861 -> [w1914 _]
      tunnel: [w1912 _] -> w1860
      tunnel: [w1911 _] -> w1859
      tunnel: [_ w1955] -> w1855
      tunnel: w1854 -> [w1908 _]
      tunnel: [w1905 _] -> w1853
      tunnel: w1852 -> [w1904 _]
      tunnel: [w1899 _] -> w1851
      tunnel: w1850 -> [w1894 _]
      tunnel: [w1893 _] -> w1849
      tunnel: w1848 -> [w1888 _]
      tunnel: [w1889 _] -> w1847
      tunnel: w1843 -> [w1877 _]
      tunnel: [w1881 _] -> w1844
      tunnel: w1845 -> [w1885 _]
      tunnel: [w1884 _] -> w1846
      tunnel: w1842 -> [w1876 _]
      tunnel: [w1872 _] -> w1841
      tunnel: w1840 -> [w1868 _]
      tunnel: [w1869 _] -> w1839
      frame #0 {
        n1104 = local read "P1 CH0 Used"() -> (w1905:bool)
        n1105 = local read "P1 CH1 Used"() -> (w1899:bool)
        n1106 = local read "P1 CH2 Used"() -> (w1869:bool)
        n1107 = local read "P2 CH0 Used"() -> (w1893:bool)
        n1108 = local read "P2 CH1 Used"() -> (w1889:bool)
        n1109 = local read "P2 CH2 Used"() -> (w1884:bool)
        n1110 = local read "P1 CH1"() -> (w1911:bool)
        n1111 = local read "P1 CH2"() -> (w1872:bool)
        n1112 = local read "P2 CH1"() -> (w1926:bool)
        n1113 = local read "P2 CH2"() -> (w1881:bool)
        n1114 = local read "P2 CH0"() -> (w1921:bool)
        n1115 = local read "P1 CH0"() -> (w1912:bool)
        n1116 = local read "System Stop"() -> (w1901:bool)
        n1117 = local read "System Stop"() -> (w1866:bool)
        n1118 = local read "System Stop"() -> (w1865:bool)
        n1119 = local read "System Stop"() -> (w1896:bool)
        n1120 = local read "System Stop"() -> (w1909:bool)
        n1121 = Less?(x=w1911, y=w1920) -> (x < y?=w1902:bool)
        n1122 = Less?(x=w1872, y=w1876) -> (x < y?=w1871:bool)
        n1123 = Less?(x=w1926, y=w1930) -> (x < y?=w1892:bool)
        n1124 = Less?(x=w1881, y=w1877) -> (x < y?=w1882:bool)
        n1125 = Less?(x=w1921, y=w1922) -> (x < y?=w1898:bool)
        n1126 = Less?(x=w1893, y=w1894) -> (x < y?=w1895:bool)
        n1127 = Less?(x=w1912, y=w1914) -> (x < y?=w1910:bool)
        n1128 = Not(x=w1901) -> (.not. x?=w1919:bool)
        n1129 = Greater?(x=w1911, y=w1920) -> (0:w1918:bool)
        n1130 = Not(x=w1866) -> (.not. x?=w1874:bool)
        n1131 = Not(x="System Stop") -> (.not. x?=w1928:bool)
        n1132 = Not(x=w1865) -> (.not. x?=w1879:bool)
        n1133 = Not(x=w1896) -> (.not. x?=w1924:bool)
        n1134 = Greater?(x=w1872, y=w1876) -> (0:w1873:bool)
        n1135 = Greater?(x=w1926, y=w1930) -> (0:w1927:bool)
        n1136 = Greater?(x=w1881, y=w1877) -> (0:w1880:bool)
        n1137 = Not(x=w1909) -> (.not. x?=w1915:bool)
        n1138 = Greater?(x=w1921, y=w1922) -> (0:w1925:bool)
        n1139 = Greater?(x=w1912, y=w1914) -> (0:w1916:bool)
        n1140 = Less?(x=w1869, y=w1868) -> (x < y?=w1867:bool)
        n1141 = Less?(x=w1889, y=w1888) -> (x < y?=w1887:bool)
        n1142 = Less?(x=w1884, y=w1885) -> (x < y?=w1886:bool)
        n1143 = Less?(x=w1905, y=w1908) -> (x < y?=w1907:bool)
        n1144 = Less?(x=w1899, y=w1904) -> (x < y?=w1900:bool)
        n1145 = And(x=w1919, y=w1918) -> (x .and. y?=w1917:bool)
        n1146 = And(x=w1874, y=w1873) -> (x .and. y?=w1875:bool)
        n1147 = Compound Arithmetic op=OR(w1898, w1896, w1895) -> (w1897:bool)
        n1148 = And(x=w1928, y=w1927) -> (x .and. y?=w1929:bool)
        n1149 = And(x=w1879, y=w1880) -> (x .and. y?=w1878:bool)
        n1150 = And(x=w1924, y=w1925) -> (x .and. y?=w1923:bool)
        n1151 = Compound Arithmetic op=OR(w1871, w1866, w1867) -> (w1870:bool)
        n1152 = Compound Arithmetic op=OR(w1892, "System Stop", w1887) -> (w1890:bool)
        n1153 = Compound Arithmetic op=OR(w1882, w1865, w1886) -> (w1883:bool)
        n1154 = And(x=w1915, y=w1916) -> (x .and. y?=w1913:bool)
        n1155 = Compound Arithmetic op=OR(w1910, w1909, w1907) -> (w1906:bool)
        n1156 = Compound Arithmetic op=OR(w1902, w1901, w1900) -> (w1903:bool)
        n1157 = stacked-sequence {
          tunnel: w1913 -> [w1944]
          tunnel: w1906 -> [w1943]
          frame #0 {
            n1158 = case shown="True" w1944 {
              frame False {
              }
              frame True {
                # "ON"
                n1159 = local write "P1 CH0"(TRUE ("P1 CH0")) -> ()
              }
            }
            n1160 = case shown="True" w1943 {
              frame False {
              }
              frame True {
                # "OFF"
                n1161 = local write "P1 CH0"(FALSE ("P1 CH0")) -> ()
              }
            }
          }
        }
        n1162 = stacked-sequence {
          tunnel: w1917 -> [w1940]
          tunnel: w1903 -> [w1939]
          frame #0 {
            n1163 = case shown="True" w1940 {
              frame False {
              }
              frame True {
                # "ON"
                n1164 = local write "P1 CH1"(TRUE ("P1 CH1")) -> ()
              }
            }
            n1165 = case shown="True" w1939 {
              frame False {
              }
              frame True {
                # "OFF"
                n1166 = local write "P1 CH1"(FALSE ("P1 CH0")) -> ()
              }
            }
          }
        }
        n1167 = stacked-sequence {
          tunnel: w1923 -> [w1948]
          tunnel: w1897 -> [w1947]
          frame #0 {
            n1168 = case shown="True" w1948 {
              frame False {
              }
              frame True {
                # "ON"
                n1169 = local write "P2 CH0"(TRUE ("P2 CH0")) -> ()
              }
            }
            n1170 = case shown="True" w1947 {
              frame False {
              }
              frame True {
                # "OFF"
                n1171 = local write "P2 CH0"(FALSE ("P1 CH0")) -> ()
              }
            }
          }
        }
        n1172 = stacked-sequence {
          tunnel: w1875 -> [w1932]
          tunnel: w1870 -> [w1931]
          frame #0 {
            n1173 = case shown="True" w1932 {
              frame False {
              }
              frame True {
                # "ON"
                n1174 = local write "P1 CH2"(TRUE ("P2 CH1")) -> ()
              }
            }
            n1175 = case shown="True" w1931 {
              frame False {
              }
              frame True {
                # "OFF"
                n1176 = local write "P1 CH2"(FALSE ("P1 CH0")) -> ()
              }
            }
          }
        }
        n1177 = stacked-sequence {
          tunnel: w1929 -> [w1952]
          tunnel: w1890 -> [w1951]
          frame #0 {
            n1178 = case shown="True" w1952 {
              frame False {
              }
              frame True {
                # "ON"
                n1179 = local write "P2 CH1"(TRUE ("P2 CH1")) -> ()
              }
            }
            n1180 = case shown="True" w1951 {
              frame False {
              }
              frame True {
                # "OFF"
                n1181 = local write "P2 CH1"(FALSE ("P1 CH0")) -> ()
              }
            }
          }
        }
        n1182 = stacked-sequence {
          tunnel: w1878 -> [w1936]
          tunnel: w1883 -> [w1935]
          frame #0 {
            n1183 = case shown="True" w1936 {
              frame False {
              }
              frame True {
                # "ON"
                n1184 = local write "P2 CH2"(TRUE ("P2 CH1")) -> ()
              }
            }
            n1185 = case shown="True" w1935 {
              frame False {
              }
              frame True {
                # "OFF"
                n1186 = local write "P2 CH2"(FALSE ("P1 CH0")) -> ()
              }
            }
          }
        }
      }
      frame #1 {
        n1187 = local read "System Stop"() -> (w1955:bool)
      }
    }
    "Power OFF" <- w1855
    n1188 = Wait (ms)(milliseconds to wait=u32 1) -> ()  [unwired: 1 out]
  }
  n1189 = while {
    shift-right: [w1968] -> _
    shift-left: FALSE -> [w1970]
    tunnel: [w1960] -> w1
    tunnel: [w1969] -> w42
    shift-right: [w1966] -> _
    shift-left: FALSE -> [w1967]
    shift-right: [w1964] -> _
    shift-left: FALSE -> [w1965]
    shift-right: [w1963] -> _
    shift-left: FALSE -> [w1962]
    tunnel: w10 -> [_]
    tunnel: w10 -> [_]
    tunnel: w10 -> [_]
    shift-right: [w1957] -> _
    shift-left: FALSE -> [w1959]
    shift-right: [w1956] -> _
    shift-left: FALSE -> [w1958]
    stop <- w1960 stop-if-true
    n1190 = Wait (ms)(milliseconds to wait="SEL Time Cycle") -> ()  [unwired: 1 out]
    n1191 = stacked-sequence {
      seq-local: [w1980 _ _ _] -> [_ _ w2221 _]
      seq-local: [w1979 _ _ _] -> [_ _ w2218 _]
      seq-local: [w1978 _ _ _] -> [_ _ w2216 _]
      seq-local: [w1977 _ _ _] -> [_ _ w2215 _]
      seq-local: [w1976 _ _ _] -> [_ _ w2208 _]
      seq-local: [w1971 _ _ _] -> [_ _ w2209 _]
      tunnel: w1970 -> [w1988 _ _ _]
      tunnel: [_ _ _ w2260] -> w1960
      tunnel: [_ w2198 _ _] -> w1969
      tunnel: [_ _ w2223 _] -> w1968
      tunnel: w1967 -> [w1986 _ _ _]
      tunnel: [_ _ w2217 _] -> w1966
      tunnel: w1965 -> [w1985 _ _ _]
      tunnel: [_ _ w2219 _] -> w1964
      tunnel: [_ _ w2220 _] -> w1963
      tunnel: w1962 -> [w1981 _ _ _]
      tunnel: w1959 -> [w1975 _ _ _]
      tunnel: w1958 -> [w1972 _ _ _]
      tunnel: [_ _ w2207 _] -> w1957
      tunnel: [_ _ w2206 _] -> w1956
      frame #0 {
        # "Детектирование SEL"
        n1192 = local read "P2 CH0"() -> (w1979:bool)
        n1193 = local read "P2 CH2"() -> (w1971:bool)
        n1194 = local read "P1 CH1"() -> (w1978:bool)
        n1195 = local read "P2 CH1"() -> (w1980:bool)
        n1196 = local read "P1 CH2"() -> (w1976:bool)
        n1197 = flat-sequence {
          tunnel: w1983 -> [w2053]
          frame #0 {
            n1198 = case shown="True" w2053 {
              frame False {
              }
              frame True {
                n1199 = Wait (ms)(milliseconds to wait=u32 50) -> ()  [unwired: 1 out]
              }
            }
          }
          frame #1 {
            n1200 = local read "P1 CH1_cur, A"() -> (w2058:dbl)
            n1201 = local read "SIM_SEL"() -> (w2056:bool)
            n1202 = Greater Or Equal?(x=w2058, y="P1 CH1_selcur, A") -> (x >= y?=w2059:bool)
            n1203 = Or(x=w2056, y=w2059) -> (x .or. y?=→"P1 CH1_warning":bool)
          }
          frame #2 {
            n1204 = local read "Считать SIM_SEL"() -> (w2065:bool)
            n1205 = local read "SIM_SEL"() -> (w2064:bool)
            n1206 = local read "P1 CH1_warning"() -> (w2060:bool)
            n1207 = Not(x=w2064) -> (.not. x?=w2063:bool)
            n1208 = Select(t=TRUE, s=w2065, f=w2063) -> (s? t:f=w2061:bool)
            n1209 = And(x=w2060, y=w2061) -> (x .and. y?=w2066:bool)
            n1210 = case shown="True" w2066 {
              frame False {
              }
              frame True {
                n1211 = local read "P1 CH1_counter"() -> (w2068:u32)
                n1212 = Increment(x=w2068) -> (x+1=→"P1 CH1_counter":u32)
              }
            }
          }
        }
        n1213 = flat-sequence {
          tunnel: w1984 -> [w2037]
          frame #0 {
            n1214 = case shown="True" w2037 {
              frame False {
              }
              frame True {
                n1215 = Wait (ms)(milliseconds to wait=u32 50) -> ()  [unwired: 1 out]
              }
            }
          }
          frame #1 {
            n1216 = local read "P2 CH0_cur, A"() -> (w2043:dbl)
            n1217 = local read "SIM_SEL"() -> (w2040:bool)
            n1218 = Greater Or Equal?(x=w2043, y="P2 CH0_selcur, A") -> (x >= y?=w2042:bool)
            n1219 = Or(x=w2040, y=w2042) -> (x .or. y?=→"P2 CH0_warning":bool)
          }
          frame #2 {
            n1220 = local read "Считать SIM_SEL"() -> (w2047:bool)
            n1221 = local read "SIM_SEL"() -> (w2048:bool)
            n1222 = local read "P2 CH0_warning"() -> (w2044:bool)
            n1223 = Not(x=w2048) -> (.not. x?=w2049:bool)
            n1224 = Select(t=TRUE, s=w2047, f=w2049) -> (s? t:f=w2046:bool)
            n1225 = And(x=w2044, y=w2046) -> (x .and. y?=w2045:bool)
            n1226 = case shown="True" w2045 {
              frame False {
              }
              frame True {
                n1227 = local read "P2 CH0_counter"() -> (w2052:u32)
                n1228 = Increment(x=w2052) -> (x+1=→"P2 CH0_counter":u32)
              }
            }
          }
        }
        n1229 = flat-sequence {
          tunnel: w1987 -> [w2069]
          frame #0 {
            n1230 = case shown="True" w2069 {
              frame False {
              }
              frame True {
                n1231 = Wait (ms)(milliseconds to wait=u32 50) -> ()  [unwired: 1 out]
              }
            }
          }
          frame #1 {
            n1232 = local read "P1 CH0_cur, A"() -> (w2075:dbl)
            n1233 = Greater Or Equal?(x=w2075, y="P1 CH0_selcur, A") -> (x >= y?=w2074:bool)
            n1234 = Or(x="SIM_SEL", y=w2074) -> (x .or. y?=→"P1 CH0_warning":bool)
          }
          frame #2 {
            n1235 = local read "SIM_SEL"() -> (w2081:bool)
            n1236 = local read "P1 CH0_warning"() -> (w2076:bool)
            n1237 = Not(x=w2081) -> (.not. x?=w2080:bool)
            n1238 = Select(t=TRUE, s="Считать SIM_SEL", f=w2080) -> (s? t:f=w2077:bool)
            n1239 = And(x=w2076, y=w2077) -> (x .and. y?=w2082:bool)
            n1240 = case shown="True" w2082 {
              frame False {
              }
              frame True {
                n1241 = local read "P1 CH0_counter"() -> (w2084:u32)
                n1242 = Increment(x=w2084) -> (x+1=→"P1 CH0_counter":u32)
              }
            }
          }
        }
        n1243 = flat-sequence {
          tunnel: w1973 -> [w1989]
          frame #0 {
            n1244 = case shown="True" w1989 {
              frame False {
              }
              frame True {
                n1245 = Wait (ms)(milliseconds to wait=u32 50) -> ()  [unwired: 1 out]
              }
            }
          }
          frame #1 {
            n1246 = local read "P2 CH2_cur, A"() -> (w1993:dbl)
            n1247 = local read "SIM_SEL"() -> (w1991:bool)
            n1248 = Greater Or Equal?(x=w1993, y="P2 CH2_selcur, A") -> (x >= y?=w1994:bool)
            n1249 = Or(x=w1991, y=w1994) -> (x .or. y?=→"P2 CH2_warning":bool)
          }
          frame #2 {
            n1250 = local read "Считать SIM_SEL"() -> (w2002:bool)
            n1251 = local read "SIM_SEL"() -> (w2001:bool)
            n1252 = local read "P2 CH2_warning"() -> (w1996:bool)
            n1253 = Not(x=w2001) -> (.not. x?=w2000:bool)
            n1254 = Select(t=TRUE, s=w2002, f=w2000) -> (s? t:f=w1998:bool)
            n1255 = And(x=w1996, y=w1998) -> (x .and. y?=w1997:bool)
            n1256 = case shown="True" w1997 {
              frame False {
              }
              frame True {
                n1257 = local read "P2 CH2_counter"() -> (w2004:u32)
                n1258 = Increment(x=w2004) -> (x+1=→"P2 CH2_counter":u32)
              }
            }
          }
        }
        n1259 = flat-sequence {
          tunnel: w1982 -> [w2021]
          frame #0 {
            n1260 = case shown="True" w2021 {
              frame False {
              }
              frame True {
                n1261 = Wait (ms)(milliseconds to wait=u32 50) -> ()  [unwired: 1 out]
              }
            }
          }
          frame #1 {
            n1262 = local read "P2 CH1_cur, A"() -> (w2025:dbl)
            n1263 = local read "SIM_SEL"() -> (w2023:bool)
            n1264 = Greater Or Equal?(x=w2025, y="P2 CH1_selcur, A") -> (x >= y?=w2026:bool)
            n1265 = Or(x=w2023, y=w2026) -> (x .or. y?=→"P2 CH1_warning":bool)
          }
          frame #2 {
            n1266 = local read "Считать SIM_SEL"() -> (w2034:bool)
            n1267 = local read "SIM_SEL"() -> (w2033:bool)
            n1268 = local read "P2 CH1_warning"() -> (w2028:bool)
            n1269 = Not(x=w2033) -> (.not. x?=w2032:bool)
            n1270 = Select(t=TRUE, s=w2034, f=w2032) -> (s? t:f=w2030:bool)
            n1271 = And(x=w2028, y=w2030) -> (x .and. y?=w2029:bool)
            n1272 = case shown="True" w2029 {
              frame False {
              }
              frame True {
                n1273 = local read "P2 CH1_counter"() -> (w2036:u32)
                n1274 = Increment(x=w2036) -> (x+1=→"P2 CH1_counter":u32)
              }
            }
          }
        }
        n1275 = local read "P1 CH0"() -> (w1977:bool)
        n1276 = flat-sequence {
          tunnel: w1974 -> [w2005]
          frame #0 {
            n1277 = case shown="True" w2005 {
              frame False {
              }
              frame True {
                n1278 = Wait (ms)(milliseconds to wait=u32 50) -> ()  [unwired: 1 out]
              }
            }
          }
          frame #1 {
            n1279 = local read "P1 CH2_cur, A"() -> (w2009:dbl)
            n1280 = local read "SIM_SEL"() -> (w2007:bool)
            n1281 = Greater Or Equal?(x=w2009, y="P1 CH2_selcur, A") -> (x >= y?=w2010:bool)
            n1282 = Or(x=w2007, y=w2010) -> (x .or. y?=→"P1 CH2_warning":bool)
          }
          frame #2 {
            n1283 = local read "Считать SIM_SEL"() -> (w2018:bool)
            n1284 = local read "SIM_SEL"() -> (w2017:bool)
            n1285 = local read "P1 CH2_warning"() -> (w2012:bool)
            n1286 = Not(x=w2017) -> (.not. x?=w2016:bool)
            n1287 = Select(t=TRUE, s=w2018, f=w2016) -> (s? t:f=w2014:bool)
            n1288 = And(x=w2012, y=w2014) -> (x .and. y?=w2013:bool)
            n1289 = case shown="True" w2013 {
              frame False {
              }
              frame True {
                n1290 = local read "P1 CH2_counter"() -> (w2020:u32)
                n1291 = Increment(x=w2020) -> (x+1=→"P1 CH2_counter":u32)
              }
            }
          }
        }
        n1292 = Greater?(x=w1979, y=w1985) -> (0:w1984:bool)
        n1293 = Greater?(x=w1977, y=w1988) -> (0:w1987:bool)
        n1294 = Greater?(x=w1971, y=w1972) -> (0:w1973:bool)
        n1295 = Greater?(x=w1978, y=w1986) -> (0:w1983:bool)
        n1296 = Greater?(x=w1980, y=w1981) -> (0:w1982:bool)
        n1297 = Greater?(x=w1976, y=w1975) -> (0:w1974:bool)
      }
      frame #1 {
        w2107 = "\t"
        w2090 = "\t"
        w2093 = 0
        w2094 = 6
        w2098 = 6
        w2124 = "\t"
        w2108 = "\t"
        w2110 = 0
        w2111 = 6
        w2116 = 6
        w2127 = "\t"
        w2137 = "\t"
        w2139 = "\t"
        w2141 = "\t"
        w2128 = "\t"
        w2129 = "\t"
        w2130 = "\t"
        w2131 = "\t"
        w2172 = 0
        w2171 = 6
        w2167 = 6
        w2177 = 0
        w2178 = 6
        w2182 = 6
        w2191 = 0
        w2190 = 6
        w2185 = 6
        w2194 = 0
        w2195 = 6
        w2201 = 6
        # "Запись логов"
        n1298 = local read "P1 CH2_cur, A"() -> (w2112:dbl)
        n1299 = local read "P1 CH1_cur, A"() -> (w2189:dbl)
        n1300 = local read "P1 CH2, V"() -> (w2114:dbl)
        n1301 = local read "P1 CH2_counter"() -> (w2109:u32)
        n1302 = local read "P1 CH2_warning"() -> (w2113:bool)
        n1303 = local read "P2 CH1, V"() -> (w2174:dbl)
        n1304 = local read "P2 CH1_cur, A"() -> (w2170:dbl)
        n1305 = local read "P2 CH1_counter"() -> (w2173:u32)
        n1306 = local read "P2 CH1_warning"() -> (w2169:bool)
        n1307 = local read "P2 CH2, V"() -> (w2091:dbl)
        n1308 = local read "P2 CH2_cur, A"() -> (w2095:dbl)
        n1309 = local read "P2 CH2_counter"() -> (w2092:u32)
        n1310 = local read "P2 CH2_warning"() -> (w2096:bool)
        n1311 = local read "P1 CH0, V"() -> (w2199:dbl)
        n1312 = local read "P1 CH0_cur, A"() -> (w2196:dbl)
        n1313 = local read "P1 CH0_counter"() -> (w2193:u32)
        n1314 = local read "P1 CH0_warning"() -> (w2197:bool)
        n1315 = local read "P1 CH1, V"() -> (w2187:dbl)
        n1316 = local read "P1 CH1_counter"() -> (w2192:u32)
        n1317 = local read "P1 CH1_warning"() -> (w2188:bool)
        n1318 = local read "P2 CH0, V"() -> (w2175:dbl)
        n1319 = local read "P2 CH0_cur, A"() -> (w2179:dbl)
        n1320 = local read "P2 CH0_counter"() -> (w2176:u32)
        n1321 = local read "P2 CH0_warning"() -> (w2180:bool)
        n1322 = Number To Fractional String(number=w2114, width (-)=w2116, precision (6)=w2116) -> (F-format string=w2118:string)  [unwired: 1 in]
        n1323 = Number To Fractional String(number=w2112, width (-)=w2111, precision (6)=w2111) -> (F-format string=w2119:string)  [unwired: 1 in]
        n1324 = Number To Fractional String(number=w2109, width (-)=w2110, precision (6)=w2110) -> (F-format string=w2120:string)  [unwired: 1 in]
        n1325 = Number To Fractional String(number=w2174, width (-)=w2167, precision (6)=w2167) -> (F-format string=w2153:string)  [unwired: 1 in]
        n1326 = Number To Fractional String(number=w2170, width (-)=w2171, precision (6)=w2171) -> (F-format string=w2152:string)  [unwired: 1 in]
        n1327 = Number To Fractional String(number=w2173, width (-)=w2172, precision (6)=w2172) -> (F-format string=w2151:string)  [unwired: 1 in]
        n1328 = Number To Fractional String(number=w2091, width (-)=w2098, precision (6)=w2098) -> (F-format string=w2100:string)  [unwired: 1 in]
        n1329 = Number To Fractional String(number=w2095, width (-)=w2094, precision (6)=w2094) -> (F-format string=w2101:string)  [unwired: 1 in]
        n1330 = Number To Fractional String(number=w2092, width (-)=w2093, precision (6)=w2093) -> (F-format string=w2102:string)  [unwired: 1 in]
        n1331 = Number To Fractional String(number=w2199, width (-)=w2201, precision (6)=w2201) -> (F-format string=w2165:string)  [unwired: 1 in]
        n1332 = Number To Fractional String(number=w2196, width (-)=w2195, precision (6)=w2195) -> (F-format string=w2164:string)  [unwired: 1 in]
        n1333 = Number To Fractional String(number=w2193, width (-)=w2194, precision (6)=w2194) -> (F-format string=w2163:string)  [unwired: 1 in]
        n1334 = Number To Fractional String(number=w2187, width (-)=w2185, precision (6)=w2185) -> (F-format string=w2161:string)  [unwired: 1 in]
        n1335 = Number To Fractional String(number=w2189, width (-)=w2190, precision (6)=w2190) -> (F-format string=w2160:string)  [unwired: 1 in]
        n1336 = Number To Fractional String(number=w2192, width (-)=w2191, precision (6)=w2191) -> (F-format string=w2159:string)  [unwired: 1 in]
        n1337 = Number To Fractional String(number=w2175, width (-)=w2182, precision (6)=w2182) -> (F-format string=w2157:string)  [unwired: 1 in]
        n1338 = Number To Fractional String(number=w2179, width (-)=w2178, precision (6)=w2178) -> (F-format string=w2156:string)  [unwired: 1 in]
        n1339 = Number To Fractional String(number=w2176, width (-)=w2177, precision (6)=w2177) -> (F-format string=w2155:string)  [unwired: 1 in]
        n1340 = Select(t="!!!2", s=w2113, f="") -> (s? t:f=w2121:string)
        n1341 = Select(t="!!!4", s=w2169, f="") -> (s? t:f=w2150:string)
        n1342 = Select(t="!!!5", s=w2096, f="") -> (s? t:f=w2103:string)
        n1343 = Select(t="!!!0", s=w2197, f="") -> (s? t:f=w2162:string)
        n1344 = Select(t="!!!1", s=w2188, f="") -> (s? t:f=w2158:string)
        n1345 = Select(t="!!!3", s=w2180, f="") -> (s? t:f=w2154:string)
        n1346 = local read "P1 CH2 Used"() -> (w2123:bool)
        n1347 = local read "P1 CH0 Used"() -> (w2146:bool)
        n1348 = local read "P1 CH1 Used"() -> (w2145:bool)
        n1349 = local read "P2 CH0 Used"() -> (w2144:bool)
        n1350 = local read "P2 CH1 Used"() -> (w2143:bool)
        n1351 = local read "P2 CH2 Used"() -> (w2104:bool)
        n1352 = Concatenate Strings(w2108, w2118, w2108, w2119, w2108, w2120, w2108, w2121) -> (w2122:string)
        n1353 = Concatenate Strings(w2131, w2165, w2131, w2164, w2131, w2163, w2131, w2162) -> (w2148:string)
        n1354 = Concatenate Strings(w2130, w2161, w2130, w2160, w2130, w2159, w2130, w2158) -> (w2149:string)
        n1355 = Concatenate Strings(w2129, w2157, w2129, w2156, w2129, w2155, w2129, w2154) -> (w2147:string)
        n1356 = Concatenate Strings(w2128, w2153, w2128, w2152, w2128, w2151, w2128, w2150) -> (w2142:string)
        n1357 = Concatenate Strings(w2090, w2100, w2090, w2101, w2090, w2102, w2090, w2103) -> (w2105:string)
        n1358 = Concatenate Strings(w2124, w2124, w2124, w2124) -> (w2125:string)
        n1359 = Concatenate Strings(w2141, w2141, w2141, w2141) -> (w2140:string)
        n1360 = Concatenate Strings(w2139, w2139, w2139, w2139) -> (w2138:string)
        n1361 = Concatenate Strings(w2137, w2137, w2137, w2137) -> (w2136:string)
        n1362 = Concatenate Strings(w2127, w2127, w2127, w2127) -> (w2135:string)
        n1363 = Concatenate Strings(w2107, w2107, w2107, w2107) -> (w2106:string)
        n1364 = Select(t=w2122, s=w2123, f=w2125) -> (s? t:f=w2089:string)
        n1365 = Select(t=w2148, s=w2146, f=w2140) -> (s? t:f=w2134:string)
        n1366 = Select(t=w2149, s=w2145, f=w2138) -> (s? t:f=w2133:string)
        n1367 = Select(t=w2147, s=w2144, f=w2136) -> (s? t:f=w2088:string)
        n1368 = Select(t=w2142, s=w2143, f=w2135) -> (s? t:f=w2087:string)
        n1369 = Select(t=w2105, s=w2104, f=w2106) -> (s? t:f=w2086:string)
        n1370 = Get Date/Time In Seconds() -> (seconds since 1Jan1904=w2204:timestamp)
        n1371 = Format Date/Time String(time format string (%c)="%H:%M:%S:%3u", seconds (now)=w2204) -> (date/time string=w2202:string)  [unwired: 1 in]
        n1372 = local read "SEL output file refnum"() -> (w2126:refnum<file>)
        n1373 = Concatenate Strings(w2202, w2134, w2133, w2089, w2088, w2087, w2086, "\r\n") -> (w2132:string)
        n1374 = Format Into String(initial string=w2126, w2132) -> (resulting string=w2198:refnum<file>)  [unwired: 2 in, 1 out]
      }
      frame #2 {
        n1375 = local read "P1 CH0_warning"() -> (w2222:bool)
        "SEL" <- w2222
        n1376 = local read "P1 CH1_warning"() -> (w2214:bool)
        n1377 = local read "P2 CH0_warning"() -> (w2212:bool)
        n1378 = local read "P2 CH1_warning"() -> (w2213:bool)
        n1379 = local read "P1 CH2_warning"() -> (w2211:bool)
        n1380 = local read "P2 CH2_warning"() -> (w2210:bool)
        n1381 = local write "SEL"(w2212) -> ()
        n1382 = local write "SEL"(w2214) -> ()
        n1383 = local write "SEL"(w2213) -> ()
        n1384 = local write "SEL"(w2211) -> ()
        n1385 = local write "SEL"(w2210) -> ()
        n1386 = case shown="True" w2222 {
          tunnel: [w2254 w2255] -> w2223
          tunnel: w2215 -> [w2254 _]
          frame False {
          }
          frame True {
            n1387 = flat-sequence {
              tunnel: [FALSE] -> w2255
              frame #0 {
                n1388 = local write "P1 CH0"(FALSE ("Power")) -> ()
              }
              frame #1 {
                n1389 = Wait (ms)(milliseconds to wait=u32 100 ("Wait_parry, ms")) -> ()  [unwired: 1 out]
              }
              frame #2 {
                n1390 = local write "P1 CH0"(TRUE ("Power")) -> ()
              }
            }
          }
        }
        n1391 = case shown="True" w2214 {
          tunnel: [w2248 w2249] -> w2217
          tunnel: w2216 -> [w2248 _]
          frame False {
          }
          frame True {
            n1392 = flat-sequence {
              tunnel: [FALSE] -> w2249
              frame #0 {
                n1393 = local write "P1 CH1"(FALSE ("Power")) -> ()
              }
              frame #1 {
                n1394 = Wait (ms)(milliseconds to wait=u32 100 ("Wait_parry, ms")) -> ()  [unwired: 1 out]
              }
              frame #2 {
                n1395 = local write "P1 CH1"(TRUE ("Power")) -> ()
              }
            }
          }
        }
        n1396 = case shown="True" w2212 {
          tunnel: [w2242 w2243] -> w2219
          tunnel: w2218 -> [w2242 _]
          frame False {
          }
          frame True {
            n1397 = flat-sequence {
              tunnel: [FALSE] -> w2243
              frame #0 {
                n1398 = local write "P2 CH0"(FALSE ("Power")) -> ()
              }
              frame #1 {
                n1399 = Wait (ms)(milliseconds to wait=u32 100 ("Wait_parry, ms")) -> ()  [unwired: 1 out]
              }
              frame #2 {
                n1400 = local write "P2 CH0"(TRUE ("Power")) -> ()
              }
            }
          }
        }
        n1401 = case shown="True" w2213 {
          tunnel: [w2236 w2237] -> w2220
          tunnel: w2221 -> [w2236 _]
          frame False {
          }
          frame True {
            n1402 = flat-sequence {
              tunnel: [FALSE] -> w2237
              frame #0 {
                n1403 = local write "P2 CH1"(FALSE ("Power")) -> ()
              }
              frame #1 {
                n1404 = Wait (ms)(milliseconds to wait=u32 100 ("Wait_parry, ms")) -> ()  [unwired: 1 out]
              }
              frame #2 {
                n1405 = local write "P2 CH1"(TRUE ("Power")) -> ()
              }
            }
          }
        }
        n1406 = case shown="True" w2211 {
          tunnel: [w2230 w2231] -> w2207
          tunnel: w2208 -> [w2230 _]
          frame False {
          }
          frame True {
            n1407 = flat-sequence {
              tunnel: [FALSE] -> w2231
              frame #0 {
                n1408 = local write "P1 CH2"(FALSE ("Power")) -> ()
              }
              frame #1 {
                n1409 = Wait (ms)(milliseconds to wait=u32 100 ("Wait_parry, ms")) -> ()  [unwired: 1 out]
              }
              frame #2 {
                n1410 = local write "P1 CH2"(TRUE ("Power")) -> ()
              }
            }
          }
        }
        n1411 = case shown="True" w2210 {
          tunnel: [w2224 w2225] -> w2206
          tunnel: w2209 -> [w2224 _]
          frame False {
          }
          frame True {
            n1412 = flat-sequence {
              tunnel: [FALSE] -> w2225
              frame #0 {
                n1413 = local write "P2 CH2"(FALSE ("Power")) -> ()
              }
              frame #1 {
                n1414 = Wait (ms)(milliseconds to wait=u32 100 ("Wait_parry, ms")) -> ()  [unwired: 1 out]
              }
              frame #2 {
                n1415 = local write "P2 CH2"(TRUE ("Power")) -> ()
              }
            }
          }
        }
      }
      frame #3 {
        n1416 = local read "System Stop"() -> (w2260:bool)
      }
    }
  }
  n1417 = while {
    tunnel: w8 -> [_]
    stop <- w2263 stop-if-true
    n1418 = Wait (ms)(milliseconds to wait=u32 100) -> ()  [unwired: 1 out]
    n1419 = case shown="True" "HMI Stop" {
      selector: "HMI Stop" -> [w2264 _]
      tunnel: [w2264 w2265] -> w2263
      frame False {
      }
      frame True {
        n1420 = local read "Glass Meas Cycle Running"() -> (w2270:bool)
        n1421 = local read "Meas Running"() -> (w2268:bool)
        n1422 = Not(x=w2270) -> (.not. x?=w2267:bool)
        n1423 = Not(x=w2268) -> (.not. x?=w2269:bool)
        n1424 = Compound Arithmetic op=AND(w2267, w2269) -> (w2266:bool)
        n1425 = case shown="False" w2266 {
          selector: w2266 -> [w2271 w2276]
          tunnel: [w2271 w2276] -> w2265
          frame False {
            n1426 = One Button Dialog(message="Please, wait for the measurement to complete.", button name ("OK")="Oh, shit, I'm sorry.") -> (true=w2275:bool)
            n1427 = Not(x=w2275) -> (.not. x?=w2274:bool)
            n1428 = local write "HMI Stop"(w2274) -> ()
          }
          frame True {
            n1429 = local write "System Stop"(w2276) -> ()
          }
        }
      }
    }
  }
  n1430 = flat-sequence {
    tunnel: w42 -> [w2284]
    tunnel: w37 -> [w2283]
    tunnel: w5 -> [w2282]
    tunnel: w1 -> [_]
    tunnel: w35 -> [w2281]
    tunnel: w4 -> [w2280]
    tunnel: w3 -> [w2278]
    tunnel: w2 -> [w2277]
    frame #0 {
      w2279 = T7."Enabled" ("Disabled")
      # "STOP"
      n1431 = case shown="True" w2278 {
        tunnel: w2283 -> [_ w2293]
        tunnel: w2281 -> [_ w2292]
        frame False {
        }
        frame True {
          n1432 = call <instrlib>:"niDCPower Close.vi"("error in (no error)"=w2292, "instrument handle"=w2293) -> ("error out"=w2291:errorcluster)  [unwired: 9 in]
          n1433 = call <vilib>:"Simple Error Handler.vi"("error in (no error)"=w2291) -> ("error out"=w2290:errorcluster)  [unwired: 1 in, 7 out]
          n1434 = local write "DC Power 1 error out"(w2290) -> ()
        }
      }
      n1435 = Close File(refnum=w2284) -> ()  [unwired: 1 in, 2 out]
      n1436 = case shown="True" w2277 {
        tunnel: w2282 -> [_ w2289]
        tunnel: w2280 -> [_ w2288]
        frame False {
        }
        frame True {
          n1437 = call <instrlib>:"niDCPower Close.vi"("error in (no error)"=w2288, "instrument handle"=w2289) -> ("error out"=w2287:errorcluster)  [unwired: 9 in]
          n1438 = call <vilib>:"Simple Error Handler.vi"("error in (no error)"=w2287) -> ("error out"=w2286:errorcluster)  [unwired: 1 in, 7 out]
          n1439 = local write "DC Power 2 error out"(w2286) -> ()
        }
      }
      n1440 = Wait (ms)(milliseconds to wait=u32 1) -> ()  [unwired: 1 out]
      n1441 = property on="NI Scope Tab" class="TabCtl (strict)"("DisabledEnum"=w2279) -> ()  [unwired: 2 in, 2 out]
      n1442 = property on="NI DMM 1 Tab" class="TabCtl (strict)"("DisabledEnum"=w2279) -> ()  [unwired: 2 in, 2 out]
      n1443 = property on="NI DMM 2 Tab" class="TabCtl (strict)"("DisabledEnum"=w2279) -> ()  [unwired: 2 in, 2 out]
      n1444 = property on="NI DMM 3 Tab" class="TabCtl (strict)"("DisabledEnum"=w2279) -> ()  [unwired: 2 in, 2 out]
      n1445 = property on="Tab DC Power 1" class="TabCtl (strict)"("DisabledEnum"=w2279) -> ()  [unwired: 2 in, 2 out]
      n1446 = property on="Tab DC Power 2" class="TabCtl (strict)"("DisabledEnum"=w2279) -> ()  [unwired: 2 in, 2 out]
      n1447 = property on="Ophir 1 Tab" class="TabCtl (strict)"("DisabledEnum"=w2279) -> ()  [unwired: 2 in, 2 out]
      n1448 = property on="Ophir 2 Tab" class="TabCtl (strict)"("DisabledEnum"=w2279) -> ()  [unwired: 2 in, 2 out]
      n1449 = property on="Stepper Motor Control" class="TabCtl (strict)"("DisabledEnum"=w2279) -> ()  [unwired: 2 in, 2 out]
      n1450 = property on="Table Tab" class="TabCtl (strict)"("DisabledEnum"=w2279) -> ()  [unwired: 2 in, 2 out]
    }
  }
  n1451 = case shown="True" w23 {
    tunnel: w10 -> [_ w2295]
    frame False {
    }
    frame True {
      n1452 = local read "Ophir 2 dup Visa Session"() -> (w2297:refnum<visa-resource-name>)
      n1453 = local read "Ophir 2 error out"() -> (w2296:errorcluster)
      n1454 = while {
        tunnel: [w2308] -> w2299
        tunnel: [w2302] -> w2298
        tunnel: w2297 -> [w2306]
        tunnel: w2296 -> [w2305]
        tunnel: w2295 -> [_]
        shift-right: [w2303] -> _
        shift-left: 0.0 -> [w2304]
        stop <- w2307 stop-if-true
        n1455 = Wait (ms)(milliseconds to wait="Ophir 2 Wait") -> ()  [unwired: 1 out]
        n1456 = stacked-sequence {
          tunnel: [w2324] -> w2308
          tunnel: [w2309] -> w2307
          tunnel: w2306 -> [w2310]
          tunnel: w2305 -> [w2319]
          tunnel: w2304 -> [w2313]
          tunnel: [w2311] -> w2303
          tunnel: [w2310] -> w2302
          frame #0 {
            n1457 = Fract/Exp String To Number(string="Ophir 2 units") -> (number=w2312:dbl)  [unwired: 3 in, 1 out]
            n1458 = call "Ophir SendPower.vi"("Visa Session"=w2310, "error in (no error)"=w2319) -> ("Value Number"=w2321:dbl, "Value String"=w2322:string, "error out"=w2324:errorcluster)  [unwired: 1 out]
            "Ophir 2 Real Optical Power" <- w2321
            n1459 = call "Ophir Over.vi"("Value String"=w2322) -> ("Overrange"=→"Ophir 2 Over Range":bool)
            n1460 = Multiply(x=w2321, y=w2312) -> (x*y=w2317:dbl)
            "Ophir 2 Char" <- w2317
            "Ophir 2 Optical Power" <- w2317
            n1461 = Greater Or Equal?(x=w2317, y=w2313) -> (x >= y?=w2318:bool)
            n1462 = Select(t=0.0, s="Ophir 2 Clear", f=w2313) -> (s? t:f=w2316:dbl)
            n1463 = Select(t=w2317, s=w2318, f=w2316) -> (s? t:f=w2311:dbl)
            "Ophir 2 MAX" <- w2311
            n1464 = local read "System Stop"() -> (w2309:bool)
          }
        }
      }
      n1465 = VISA Close(VISA resource name=w2298, error in (no error)=w2299) -> (error out=w2300:errorcluster)
      n1466 = call "Ophir Error Message.vi"("error in (no error)"=w2300) -> ()  [unwired: 3 in, 4 out]
    }
  }
  n1467 = case shown="True" w24 {
    tunnel: w10 -> [_ w2326]
    frame False {
    }
    frame True {
      n1468 = local read "Ophir 1 dup Visa Session"() -> (w2328:refnum<visa-resource-name>)
      n1469 = local read "Ophir 1 error out"() -> (w2327:errorcluster)
      n1470 = while {
        tunnel: [w2339] -> w2330
        tunnel: [w2333] -> w2329
        tunnel: w2328 -> [w2337]
        tunnel: w2327 -> [w2336]
        tunnel: w2326 -> [_]
        shift-right: [w2334] -> _
        shift-left: 0.0 -> [w2335]
        stop <- w2338 stop-if-true
        n1471 = Wait (ms)(milliseconds to wait="Ophir 1 Wait") -> ()  [unwired: 1 out]
        n1472 = stacked-sequence {
          tunnel: [w2355] -> w2339
          tunnel: [w2340] -> w2338
          tunnel: w2337 -> [w2342]
          tunnel: w2336 -> [w2351]
          tunnel: w2335 -> [w2345]
          tunnel: [w2343] -> w2334
          tunnel: [w2342] -> w2333
          frame #0 {
            n1473 = Fract/Exp String To Number(string="Ophir 1 units") -> (number=w2344:dbl)  [unwired: 3 in, 1 out]
            n1474 = call "Ophir SendPower.vi"("Visa Session"=w2342, "error in (no error)"=w2351) -> ("Value Number"=w2341:dbl, "Value String"=w2353:string, "error out"=w2355:errorcluster)  [unwired: 1 out]
            "Ophir 1 Real Optical Power" <- w2341
            n1475 = call "Ophir Over.vi"("Value String"=w2353) -> ("Overrange"=→"Ophir 1 Over Range":bool)
            n1476 = Multiply(x=w2341, y=w2344) -> (x*y=w2349:dbl)
            "Ophir 1 Char" <- w2349
            "Ophir 1 Optical Power" <- w2349
            n1477 = Greater Or Equal?(x=w2349, y=w2345) -> (x >= y?=w2350:bool)
            n1478 = Select(t=0.0, s="Ophir 1 Clear", f=w2345) -> (s? t:f=w2348:dbl)
            n1479 = Select(t=w2349, s=w2350, f=w2348) -> (s? t:f=w2343:dbl)
            "Ophir 1 MAX" <- w2343
            n1480 = local read "System Stop"() -> (w2340:bool)
          }
        }
      }
      n1481 = VISA Close(VISA resource name=w2329, error in (no error)=w2330) -> (error out=w2331:errorcluster)
      n1482 = call "Ophir Error Message.vi"("error in (no error)"=w2331) -> ()  [unwired: 3 in, 4 out]
    }
  }
